vi "OCV Histogram 4309.vi"(8 "Error In":errorcluster, 10 "Results Input":T4={"V ch0 Array"=[], "V ch1 Array"=[], "V ch2 Array"=[], "V ch3 Array"=[], "V ch4 Array"=[], "Elapsed Time (ms)"=11164, "DMM Fault Array"=[]}) -> (0 "Error Out":errorcluster, 1 "mean values of channels":dbl[](array[numeric])=[-6.648192609520545e-06, -2.6579412172609335e-06, 5.730660716698524e-06, 9.480335334891014e-06, -2.6031729589807576e-07] format="%#_7p", 2 "std dev":dbl=4.593584714427233e-07 format="%.3p", 3 "range":dbl=1.8604783993401584e-06 format="%.3p", 4 "Results Output":T3={"ch3 range"=1.5284304409643419e-06, "ch3 std dev"=3.7432297421944963e-07, "ch3 mean"=9.480335334891014e-06, "Histogram Graph ch3"={"X Values"=[8.804122636382775e-06, 8.956965680479209e-06, 9.109808724575643e-06, 9.262651768672077e-06, 9.415494812768511e-06, 9.568337856864946e-06, 9.72118090096138e-06, 9.874023945057814e-06, 1.0026866989154248e-05, 1.0179710033250682e-05], "Histogram: h(x)"=[2, 4, 3, 7, 5, 3, 7, 6, 1, 2]}, "ch2 range"=1.9041594218219493e-06, "ch2 std dev"=4.1579103732429095e-07, "ch2 mean"=5.730660716698524e-06, "Histogram Graph ch2"={"X Values"=[4.8417078226500296e-06, 5.032123764832224e-06, 5.222539707014419e-06, 5.412955649196613e-06, 5.603371591378808e-06, 5.7937875335610025e-06, 5.984203475743197e-06, 6.174619417925392e-06, 6.365035360107586e-06, 6.555451302289781e-06], "Histogram: h(x)"=[2, 2, 4, 3, 5, 8, 9, 5, 1, 1]}, "ch1 range"=1.7442902903444177e-06, "ch1 std dev"=4.468204660544414e-07, "ch1 mean"=-2.6579412172609335e-06, "Histogram Graph ch1"={"X Values"=[-3.3982864936427982e-06, -3.2238574646083565e-06, -3.0494284355739147e-06, -2.874999406539473e-06, -2.700570377505031e-06, -2.5261413484705894e-06, -2.3517123194361476e-06, -2.177283290401706e-06, -2.002854261367264e-06, -1.8284252323328223e-06], "Histogram: h(x)"=[4, 3, 5, 1, 6, 8, 4, 5, 3, 1]}, "ch0 range"=1.9838415017287296e-06, "ch0 std dev"=5.022029434534627e-07, "ch0 mean"=-6.648192609520545e-06, "Histogram Graph ch0"={"X Values"=[-7.4214795585101575e-06, -7.223095408337285e-06, -7.024711258164412e-06, -6.82632710799154e-06, -6.627942957818667e-06, -6.4295588076457944e-06, -6.231174657472922e-06, -6.032790507300049e-06, -5.8344063571271766e-06, -5.636022206954304e-06], "Histogram: h(x)"=[5, 3, 4, 6, 4, 8, 4, 1, 4, 1]}, "Waveform Chart ch1"=[-2.622437675041801e-06, -2.1054414953660847e-06, -2.3277676624794484e-06, -2.558376653803712e-06, -2.2236999675494533e-06, -2.589016451053761e-06, -2.6354278960691e-06, -2.7367192087189563e-06, -2.424017879995447e-06, -3.0489161443253215e-06, -3.1442148467963687e-06, -2.4032855210096374e-06, -2.569647882839888e-06, -2.4698150005498013e-06, -3.0781658817195746e-06, -2.377010372332436e-06, -2.0435595699758798e-06, -2.106839167327596e-06, -1.7412107178156014e-06, -3.2480049993772076e-06, -1.9805074376907754e-06, -2.5608807141114243e-06, -2.18054640635336e-06, -3.099457174386434e-06, -3.102303246629032e-06, -3.2920758007788295e-06, -3.3778499352142414e-06, -3.3187560901861313e-06, -3.484840052811922e-06, -3.485501008160019e-06, -2.8728971850629594e-06, -2.6623123946996634e-06, -2.187546597757112e-06, -2.5467930720162336e-06, -2.7862697099761513e-06, -2.528638777412977e-06, -2.0537236385737207e-06, -2.5329982714180255e-06, -2.7424337661967574e-06, -3.067742416854491e-06], "Waveform Chart ch2"=[5.544446756924017e-06, 5.893818847440082e-06, 5.6959361744068e-06, 6.353655436755351e-06, 6.650659273380882e-06, 6.187390686867271e-06, 6.20360970192913e-06, 5.7770612172558695e-06, 5.816303483036932e-06, 5.681492261411933e-06, 5.92762437831725e-06, 6.190843181120228e-06, 5.928079790707314e-06, 6.068116911256402e-06, 6.161619546592655e-06, 5.5543262999422065e-06, 6.17040032539053e-06, 5.4655577958543896e-06, 5.76704970728763e-06, 6.0194055222271105e-06, 5.783390336812049e-06, 5.768011867723238e-06, 6.0153044120154e-06, 6.001437704705948e-06, 5.911709913790112e-06, 5.830095407868431e-06, 5.25398022881523e-06, 5.15697143423068e-06, 4.826305970962092e-06, 5.462550730311096e-06, 5.059430867978049e-06, 5.682513029845579e-06, 5.851683523904261e-06, 5.099226732675129e-06, 5.2309820281174504e-06, 5.22374278950658e-06, 5.829274618675769e-06, 4.746499851558932e-06, 5.396447289671177e-06, 6.039472630669777e-06], "Waveform Chart ch0"=[-6.482741875349764e-06, -6.609674165618734e-06, -6.233203080218623e-06, -6.613210951394088e-06, -5.909245924550351e-06, -6.1328996888307884e-06, -6.358200673203053e-06, -6.870973185430456e-06, -6.243427483099904e-06, -5.953840097279857e-06, -6.577614794730629e-06, -5.768388563769013e-06, -5.889962020259323e-06, -5.91212430154465e-06, -6.419565311385181e-06, -6.50829315132552e-06, -5.536830131867864e-06, -6.271011369459595e-06, -6.937542782195293e-06, -7.44168991871554e-06, -6.8984467501811205e-06, -7.4441074466820366e-06, -6.884514522294152e-06, -7.229455884586274e-06, -7.204633996616539e-06, -7.520671633596594e-06, -7.348344858091178e-06, -7.026224856705287e-06, -6.4957495291395714e-06, -6.9697185324009035e-06, -6.64170832689038e-06, -6.516226556717238e-06, -6.80187883727134e-06, -7.473746530800666e-06, -6.8019074543289836e-06, -6.421730747707948e-06, -6.915517716049444e-06, -7.233306065769019e-06, -6.9335647318597554e-06, -6.495809932905111e-06], "Waveform Chart ch3"=[9.329772359568193e-06, 9.772186603754015e-06, 9.974785258468733e-06, 1.02561315552989e-05, 9.495402230894659e-06, 9.736598828932665e-06, 9.898850155608759e-06, 1.0197036488504313e-05, 9.305987891150035e-06, 9.316802834906767e-06, 9.746712874470878e-06, 9.737416581604666e-06, 9.867514527065477e-06, 9.509080464808271e-06, 9.481845866845764e-06, 9.70755176396829e-06, 8.885838770613302e-06, 9.475699672125386e-06, 9.258180372816345e-06, 9.834891872602234e-06, 9.402243918552161e-06, 9.713205786936326e-06, 9.876491292911543e-06, 9.871789580104262e-06, 9.650930388911628e-06, 9.41118365911455e-06, 9.575353492249282e-06, 9.196921234035763e-06, 9.15123272945548e-06, 8.949563027841687e-06, 9.474861956745276e-06, 8.825224921180636e-06, 8.727701114334558e-06, 9.16860173648142e-06, 8.905227736485157e-06, 9.144446889757383e-06, 8.885482293855075e-06, 9.859395612279415e-06, 9.32444154185109e-06, 9.310827508550253e-06]} {"ch3 range" format="%#_6p"; "ch3 std dev" format="%#.3p"; "ch3 mean" format="%#.6p"; "ch2 range" format="%#_6p"; "ch2 std dev" format="%#.3p"; "ch2 mean" format="%#.6p"; "ch1 range" format="%#_6p"; "ch1 std dev" format="%#.3p"; "ch1 mean" format="%#.6p"; "ch0 range" format="%#_6p"; "ch0 std dev" format="%#.3p"; "ch0 mean" format="%#.6p"}, 5 "Elapsed Time (ms)":u32)   [LabVIEW 2019]
uses:
  OCVResults.ctl
  Chart_Graph_Mean_Range_StdDev.ctl
  VIs/MeasurementServer_OCVRawData.ctl
  VIs/MeasurementServer_ErrorOutData.ctl
  <vilib>/Analysis/baseanly.llb/Mean (DBL).vi
  <vilib>/Analysis/NI_AALBase.lvlib
  <vilib>/gmath/NI_Gmath.lvlib
  VIs/labview-grpc-measurement-server.lvlib
panel:
  in  "OCVResults":T1[](array[typedef])=[{"battery1voltage"=3.4816353, "battery2voltage"=3.4830456, "battery3voltage"=3.4783695, "battery4voltage"=3.482367, "battery5voltage"=3.4843996, "battery6voltage"=0.0, "battery7voltage"=0.0, "battery8voltage"=0.0, "battery9voltage"=0.0, "battery10voltage"=0.0, "battery11voltage"=0.0, "battery12voltage"=0.0, "battery13voltage"=0.0, "battery14voltage"=0.0, "battery15voltage"=0.0, "battery16voltage"=0.0, "battery17voltage"=0.0, "battery18voltage"=0.0, "battery19voltage"=0.0, "battery20voltage"=0.0, "battery21voltage"=0.0, "battery22voltage"=0.0, "battery23voltage"=0.0, "battery24voltage"=0.0, "ErrorOutData"={"ErrorCode"=0, "ErrorMessage"=""}}, {"battery1voltage"=3.4816356, "battery2voltage"=3.4830368, "battery3voltage"=3.4783683, "battery4voltage"=3.4823706, "battery5voltage"=3.4844058, "battery6voltage"=0.0, "battery7voltage"=0.0, "battery8voltage"=0.0, "battery9voltage"=0.0, "battery10voltage"=0.0, "battery11voltage"=0.0, "battery12voltage"=0.0, "battery13voltage"=0.0, "battery14voltage"=0.0, "battery15voltage"=0.0, "battery16voltage"=0.0, "battery17voltage"=0.0, "battery18voltage"=0.0, "battery19voltage"=0.0, "battery20voltage"=0.0, "battery21voltage"=0.0, "battery22voltage"=0.0, "battery23voltage"=0.0, "battery24voltage"=0.0, "ErrorOutData"={"ErrorCode"=0, "ErrorMessage"=""}}, {"battery1voltage"=3.4816363, "battery2voltage"=3.4830387, "battery3voltage"=3.478373, "battery4voltage"=3.4823644, "battery5voltage"=3.4844077, "battery6voltage"=0.0, "battery7voltage"=0.0, "battery8voltage"=0.0, "battery9voltage"=0.0, "battery10voltage"=0.0, "battery11voltage"=0.0, "battery12voltage"=0.0, "battery13voltage"=0.0, "battery14voltage"=0.0, "battery15voltage"=0.0, "battery16voltage"=0.0, "battery17voltage"=0.0, "battery18voltage"=0.0, "battery19voltage"=0.0, "battery20voltage"=0.0, "battery21voltage"=0.0, "battery22voltage"=0.0, "battery23voltage"=0.0, "battery24voltage"=0.0, "ErrorOutData"={"ErrorCode"=0, "ErrorMessage"=""}}, {"battery1voltage"=3.4816382, "battery2voltage"=3.4830468, "battery3voltage"=3.478372, "battery4voltage"=3.4823663, "battery5voltage"=3.4844036, "battery6voltage"=0.0, "battery7voltage"=0.0, "battery8voltage"=0.0, "battery9voltage"=0.0, "battery10voltage"=0.0, "battery11voltage"=0.0, "battery12voltage"=0.0, "battery13voltage"=0.0, "battery14voltage"=0.0, "battery15voltage"=0.0, "battery16voltage"=0.0, "battery17voltage"=0.0, "battery18voltage"=0.0, "battery19voltage"=0.0, "battery20voltage"=0.0, "battery21voltage"=0.0, "battery22voltage"=0.0, "battery23voltage"=0.0, "battery24voltage"=0.0, "ErrorOutData"={"ErrorCode"=0, "ErrorMessage"=""}}, {"battery1voltage"=3.4816408, "battery2voltage"=3.4830465, "battery3voltage"=3.478378, "battery4voltage"=3.48237, "battery5voltage"=3.4843988, "battery6voltage"=0.0, "battery7voltage"=0.0, "battery8voltage"=0.0, "battery9voltage"=0.0, "battery10voltage"=0.0, "battery11voltage"=0.0, "battery12voltage"=0.0, "battery13voltage"=0.0, "battery14voltage"=0.0, "battery15voltage"=0.0, "battery16voltage"=0.0, "battery17voltage"=0.0, "battery18voltage"=0.0, "battery19voltage"=0.0, "battery20voltage"=0.0, "battery21voltage"=0.0, "battery22voltage"=0.0, "battery23voltage"=0.0, "battery24voltage"=0.0, "ErrorOutData"={"ErrorCode"=0, "ErrorMessage"=""}}, {"battery1voltage"=3.48164, "battery2voltage"=3.4830382, "battery3voltage"=3.4783747, "battery4voltage"=3.4823658, "battery5voltage"=3.4843998, "battery6voltage"=0.0, "battery7voltage"=0.0, "battery8voltage"=0.0, "battery9voltage"=0.0, "battery10voltage"=0.0, "battery11voltage"=0.0, "battery12voltage"=0.0, "battery13voltage"=0.0, "battery14voltage"=0.0, "battery15voltage"=0.0, "battery16voltage"=0.0, "battery17voltage"=0.0, "battery18voltage"=0.0, "battery19voltage"=0.0, "battery20voltage"=0.0, "battery21voltage"=0.0, "battery22voltage"=0.0, "battery23voltage"=0.0, "battery24voltage"=0.0, "ErrorOutData"={"ErrorCode"=0, "ErrorMessage"=""}}, {"battery1voltage"=3.481639, "battery2voltage"=3.4830444, "battery3voltage"=3.4783697, "battery4voltage"=3.482369, "battery5voltage"=3.4844058, "battery6voltage"=0.0, "battery7voltage"=0.0, "battery8voltage"=0.0, "battery9voltage"=0.0, "battery10voltage"=0.0, "battery11voltage"=0.0, "battery12voltage"=0.0, "battery13voltage"=0.0, "battery14voltage"=0.0, "battery15voltage"=0.0, "battery16voltage"=0.0, "battery17voltage"=0.0, "battery18voltage"=0.0, "battery19voltage"=0.0, "battery20voltage"=0.0, "battery21voltage"=0.0, "battery22voltage"=0.0, "battery23voltage"=0.0, "battery24voltage"=0.0, "ErrorOutData"={"ErrorCode"=0, "ErrorMessage"=""}}, {"battery1voltage"=3.4816341, "battery2voltage"=3.483041, "battery3voltage"=3.4783704, "battery4voltage"=3.4823651, "battery5voltage"=3.4844072, "battery6voltage"=0.0, "battery7voltage"=0.0, "battery8voltage"=0.0, "battery9voltage"=0.0, "battery10voltage"=0.0, "battery11voltage"=0.0, "battery12voltage"=0.0, "battery13voltage"=0.0, "battery14voltage"=0.0, "battery15voltage"=0.0, "battery16voltage"=0.0, "battery17voltage"=0.0, "battery18voltage"=0.0, "battery19voltage"=0.0, "battery20voltage"=0.0, "battery21voltage"=0.0, "battery22voltage"=0.0, "battery23voltage"=0.0, "battery24voltage"=0.0, "ErrorOutData"={"ErrorCode"=0, "ErrorMessage"=""}}, {"battery1voltage"=3.481641, "battery2voltage"=3.4830418, "battery3voltage"=3.4783719, "battery4voltage"=3.482372, "battery5voltage"=3.4844098, "battery6voltage"=0.0, "battery7voltage"=0.0, "battery8voltage"=0.0, "battery9voltage"=0.0, "battery10voltage"=0.0, "battery11voltage"=0.0, "battery12voltage"=0.0, "battery13voltage"=0.0, "battery14voltage"=0.0, "battery15voltage"=0.0, "battery16voltage"=0.0, "battery17voltage"=0.0, "battery18voltage"=0.0, "battery19voltage"=0.0, "battery20voltage"=0.0, "battery21voltage"=0.0, "battery22voltage"=0.0, "battery23voltage"=0.0, "battery24voltage"=0.0, "ErrorOutData"={"ErrorCode"=0, "ErrorMessage"=""}}, {"battery1voltage"=3.4816356, "battery2voltage"=3.4830396, "battery3voltage"=3.478371, "battery4voltage"=3.4823728, "battery5voltage"=3.4844012, "battery6voltage"=0.0, "battery7voltage"=0.0, "battery8voltage"=0.0, "battery9voltage"=0.0, "battery10voltage"=0.0, "battery11voltage"=0.0, "battery12voltage"=0.0, "battery13voltage"=0.0, "battery14voltage"=0.0, "battery15voltage"=0.0, "battery16voltage"=0.0, "battery17voltage"=0.0, "battery18voltage"=0.0, "battery19voltage"=0.0, "battery20voltage"=0.0, "battery21voltage"=0.0, "battery22voltage"=0.0, "battery23voltage"=0.0, "battery24voltage"=0.0, "ErrorOutData"={"ErrorCode"=0, "ErrorMessage"=""}}, {"battery1voltage"=3.4816346, "battery2voltage"=3.483039, "battery3voltage"=3.478373, "battery4voltage"=3.4823637, "battery5voltage"=3.4844048, "battery6voltage"=0.0, "battery7voltage"=0.0, "battery8voltage"=0.0, "battery9voltage"=0.0, "battery10voltage"=0.0, "battery11voltage"=0.0, "battery12voltage"=0.0, "battery13voltage"=0.0, "battery14voltage"=0.0, "battery15voltage"=0.0, "battery16voltage"=0.0, "battery17voltage"=0.0, "battery18voltage"=0.0, "battery19voltage"=0.0, "battery20voltage"=0.0, "battery21voltage"=0.0, "battery22voltage"=0.0, "battery23voltage"=0.0, "battery24voltage"=0.0, "ErrorOutData"={"ErrorCode"=0, "ErrorMessage"=""}}, {"battery1voltage"=3.4816375, "battery2voltage"=3.4830399, "battery3voltage"=3.4783738, "battery4voltage"=3.4823651, "battery5voltage"=3.4844062, "battery6voltage"=0.0, "battery7voltage"=0.0, "battery8voltage"=0.0, "battery9voltage"=0.0, "battery10voltage"=0.0, "battery11voltage"=0.0, "battery12voltage"=0.0, "battery13voltage"=0.0, "battery14voltage"=0.0, "battery15voltage"=0.0, "battery16voltage"=0.0, "battery17voltage"=0.0, "battery18voltage"=0.0, "battery19voltage"=0.0, "battery20voltage"=0.0, "battery21voltage"=0.0, "battery22voltage"=0.0, "battery23voltage"=0.0, "battery24voltage"=0.0, "ErrorOutData"={"ErrorCode"=0, "ErrorMessage"=""}}, {"battery1voltage"=3.4816372, "battery2voltage"=3.4830463, "battery3voltage"=3.478377, "battery4voltage"=3.4823728, "battery5voltage"=3.484404, "battery6voltage"=0.0, "battery7voltage"=0.0, "battery8voltage"=0.0, "battery9voltage"=0.0, "battery10voltage"=0.0, "battery11voltage"=0.0, "battery12voltage"=0.0, "battery13voltage"=0.0, "battery14voltage"=0.0, "battery15voltage"=0.0, "battery16voltage"=0.0, "battery17voltage"=0.0, "battery18voltage"=0.0, "battery19voltage"=0.0, "battery20voltage"=0.0, "battery21voltage"=0.0, "battery22voltage"=0.0, "battery23voltage"=0.0, "battery24voltage"=0.0, "ErrorOutData"={"ErrorCode"=0, "ErrorMessage"=""}}, {"battery1voltage"=3.481637, "battery2voltage"=3.4830413, "battery3voltage"=3.4783728, "battery4voltage"=3.482369, "battery5voltage"=3.484405, "battery6voltage"=0.0, "battery7voltage"=0.0, "battery8voltage"=0.0, "battery9voltage"=0.0, "battery10voltage"=0.0, "battery11voltage"=0.0, "battery12voltage"=0.0, "battery13voltage"=0.0, "battery14voltage"=0.0, "battery15voltage"=0.0, "battery16voltage"=0.0, "battery17voltage"=0.0, "battery18voltage"=0.0, "battery19voltage"=0.0, "battery20voltage"=0.0, "battery21voltage"=0.0, "battery22voltage"=0.0, "battery23voltage"=0.0, "battery24voltage"=0.0, "ErrorOutData"={"ErrorCode"=0, "ErrorMessage"=""}}, {"battery1voltage"=3.4816399, "battery2voltage"=3.4830387, "battery3voltage"=3.4783702, "battery4voltage"=3.4823713, "battery5voltage"=3.4844084, "battery6voltage"=0.0, "battery7voltage"=0.0, "battery8voltage"=0.0, "battery9voltage"=0.0, "battery10voltage"=0.0, "battery11voltage"=0.0, "battery12voltage"=0.0, "battery13voltage"=0.0, "battery14voltage"=0.0, "battery15voltage"=0.0, "battery16voltage"=0.0, "battery17voltage"=0.0, "battery18voltage"=0.0, "battery19voltage"=0.0, "battery20voltage"=0.0, "battery21voltage"=0.0, "battery22voltage"=0.0, "battery23voltage"=0.0, "battery24voltage"=0.0, "ErrorOutData"={"ErrorCode"=0, "ErrorMessage"=""}}, {"battery1voltage"=3.4816375, "battery2voltage"=3.4830422, "battery3voltage"=3.4783688, "battery4voltage"=3.4823675, "battery5voltage"=3.4843993, "battery6voltage"=0.0, "battery7voltage"=0.0, "battery8voltage"=0.0, "battery9voltage"=0.0, "battery10voltage"=0.0, "battery11voltage"=0.0, "battery12voltage"=0.0, "battery13voltage"=0.0, "battery14voltage"=0.0, "battery15voltage"=0.0, "battery16voltage"=0.0, "battery17voltage"=0.0, "battery18voltage"=0.0, "battery19voltage"=0.0, "battery20voltage"=0.0, "battery21voltage"=0.0, "battery22voltage"=0.0, "battery23voltage"=0.0, "battery24voltage"=0.0, "ErrorOutData"={"ErrorCode"=0, "ErrorMessage"=""}}, {"battery1voltage"=3.4816432, "battery2voltage"=3.4830387, "battery3voltage"=3.478373, "battery4voltage"=3.482368, "battery5voltage"=3.484403, "battery6voltage"=0.0, "battery7voltage"=0.0, "battery8voltage"=0.0, "battery9voltage"=0.0, "battery10voltage"=0.0, "battery11voltage"=0.0, "battery12voltage"=0.0, "battery13voltage"=0.0, "battery14voltage"=0.0, "battery15voltage"=0.0, "battery16voltage"=0.0, "battery17voltage"=0.0, "battery18voltage"=0.0, "battery19voltage"=0.0, "battery20voltage"=0.0, "battery21voltage"=0.0, "battery22voltage"=0.0, "battery23voltage"=0.0, "battery24voltage"=0.0, "ErrorOutData"={"ErrorCode"=0, "ErrorMessage"=""}}, {"battery1voltage"=3.4816358, "battery2voltage"=3.483043, "battery3voltage"=3.4783685, "battery4voltage"=3.4823685, "battery5voltage"=3.484403, "battery6voltage"=0.0, "battery7voltage"=0.0, "battery8voltage"=0.0, "battery9voltage"=0.0, "battery10voltage"=0.0, "battery11voltage"=0.0, "battery12voltage"=0.0, "battery13voltage"=0.0, "battery14voltage"=0.0, "battery15voltage"=0.0, "battery16voltage"=0.0, "battery17voltage"=0.0, "battery18voltage"=0.0, "battery19voltage"=0.0, "battery20voltage"=0.0, "battery21voltage"=0.0, "battery22voltage"=0.0, "battery23voltage"=0.0, "battery24voltage"=0.0, "ErrorOutData"={"ErrorCode"=0, "ErrorMessage"=""}}, {"battery1voltage"=3.4816375, "battery2voltage"=3.483041, "battery3voltage"=3.4783714, "battery4voltage"=3.4823701, "battery5voltage"=3.484405, "battery6voltage"=0.0, "battery7voltage"=0.0, "battery8voltage"=0.0, "battery9voltage"=0.0, "battery10voltage"=0.0, "battery11voltage"=0.0, "battery12voltage"=0.0, "battery13voltage"=0.0, "battery14voltage"=0.0, "battery15voltage"=0.0, "battery16voltage"=0.0, "battery17voltage"=0.0, "battery18voltage"=0.0, "battery19voltage"=0.0, "battery20voltage"=0.0, "battery21voltage"=0.0, "battery22voltage"=0.0, "battery23voltage"=0.0, "battery24voltage"=0.0, "ErrorOutData"={"ErrorCode"=0, "ErrorMessage"=""}}, {"battery1voltage"=3.48164, "battery2voltage"=3.4830444, "battery3voltage"=3.4783697, "battery4voltage"=3.4823718, "battery5voltage"=3.4844031, "battery6voltage"=0.0, "battery7voltage"=0.0, "battery8voltage"=0.0, "battery9voltage"=0.0, "battery10voltage"=0.0, "battery11voltage"=0.0, "battery12voltage"=0.0, "battery13voltage"=0.0, "battery14voltage"=0.0, "battery15voltage"=0.0, "battery16voltage"=0.0, "battery17voltage"=0.0, "battery18voltage"=0.0, "battery19voltage"=0.0, "battery20voltage"=0.0, "battery21voltage"=0.0, "battery22voltage"=0.0, "battery23voltage"=0.0, "battery24voltage"=0.0, "ErrorOutData"={"ErrorCode"=0, "ErrorMessage"=""}}, {"battery1voltage"=3.4816394, "battery2voltage"=3.4830453, "battery3voltage"=3.4783723, "battery4voltage"=3.4823713, "battery5voltage"=3.4843984, "battery6voltage"=0.0, "battery7voltage"=0.0, "battery8voltage"=0.0, "battery9voltage"=0.0, "battery10voltage"=0.0, "battery11voltage"=0.0, "battery12voltage"=0.0, "battery13voltage"=0.0, "battery14voltage"=0.0, "battery15voltage"=0.0, "battery16voltage"=0.0, "battery17voltage"=0.0, "battery18voltage"=0.0, "battery19voltage"=0.0, "battery20voltage"=0.0, "battery21voltage"=0.0, "battery22voltage"=0.0, "battery23voltage"=0.0, "battery24voltage"=0.0, "ErrorOutData"={"ErrorCode"=0, "ErrorMessage"=""}}, {"battery1voltage"=3.4816341, "battery2voltage"=3.4830413, "battery3voltage"=3.4783728, "battery4voltage"=3.4823737, "battery5voltage"=3.4844046, "battery6voltage"=0.0, "battery7voltage"=0.0, "battery8voltage"=0.0, "battery9voltage"=0.0, "battery10voltage"=0.0, "battery11voltage"=0.0, "battery12voltage"=0.0, "battery13voltage"=0.0, "battery14voltage"=0.0, "battery15voltage"=0.0, "battery16voltage"=0.0, "battery17voltage"=0.0, "battery18voltage"=0.0, "battery19voltage"=0.0, "battery20voltage"=0.0, "battery21voltage"=0.0, "battery22voltage"=0.0, "battery23voltage"=0.0, "battery24voltage"=0.0, "ErrorOutData"={"ErrorCode"=0, "ErrorMessage"=""}}, {"battery1voltage"=3.4816387, "battery2voltage"=3.4830446, "battery3voltage"=3.4783685, "battery4voltage"=3.482368, "battery5voltage"=3.4844067, "battery6voltage"=0.0, "battery7voltage"=0.0, "battery8voltage"=0.0, "battery9voltage"=0.0, "battery10voltage"=0.0, "battery11voltage"=0.0, "battery12voltage"=0.0, "battery13voltage"=0.0, "battery14voltage"=0.0, "battery15voltage"=0.0, "battery16voltage"=0.0, "battery17voltage"=0.0, "battery18voltage"=0.0, "battery19voltage"=0.0, "battery20voltage"=0.0, "battery21voltage"=0.0, "battery22voltage"=0.0, "battery23voltage"=0.0, "battery24voltage"=0.0, "ErrorOutData"={"ErrorCode"=0, "ErrorMessage"=""}}, {"battery1voltage"=3.4816349, "battery2voltage"=3.48304, "battery3voltage"=3.4783728, "battery4voltage"=3.482367, "battery5voltage"=3.4844062, "battery6voltage"=0.0, "battery7voltage"=0.0, "battery8voltage"=0.0, "battery9voltage"=0.0, "battery10voltage"=0.0, "battery11voltage"=0.0, "battery12voltage"=0.0, "battery13voltage"=0.0, "battery14voltage"=0.0, "battery15voltage"=0.0, "battery16voltage"=0.0, "battery17voltage"=0.0, "battery18voltage"=0.0, "battery19voltage"=0.0, "battery20voltage"=0.0, "battery21voltage"=0.0, "battery22voltage"=0.0, "battery23voltage"=0.0, "battery24voltage"=0.0, "ErrorOutData"={"ErrorCode"=0, "ErrorMessage"=""}}, {"battery1voltage"=3.4816382, "battery2voltage"=3.483041, "battery3voltage"=3.4783733, "battery4voltage"=3.4823716, "battery5voltage"=3.4844053, "battery6voltage"=0.0, "battery7voltage"=0.0, "battery8voltage"=0.0, "battery9voltage"=0.0, "battery10voltage"=0.0, "battery11voltage"=0.0, "battery12voltage"=0.0, "battery13voltage"=0.0, "battery14voltage"=0.0, "battery15voltage"=0.0, "battery16voltage"=0.0, "battery17voltage"=0.0, "battery18voltage"=0.0, "battery19voltage"=0.0, "battery20voltage"=0.0, "battery21voltage"=0.0, "battery22voltage"=0.0, "battery23voltage"=0.0, "battery24voltage"=0.0, "ErrorOutData"={"ErrorCode"=0, "ErrorMessage"=""}}, {"battery1voltage"=3.481638, "battery2voltage"=3.4830427, "battery3voltage"=3.4783704, "battery4voltage"=3.4823666, "battery5voltage"=3.4844048, "battery6voltage"=0.0, "battery7voltage"=0.0, "battery8voltage"=0.0, "battery9voltage"=0.0, "battery10voltage"=0.0, "battery11voltage"=0.0, "battery12voltage"=0.0, "battery13voltage"=0.0, "battery14voltage"=0.0, "battery15voltage"=0.0, "battery16voltage"=0.0, "battery17voltage"=0.0, "battery18voltage"=0.0, "battery19voltage"=0.0, "battery20voltage"=0.0, "battery21voltage"=0.0, "battery22voltage"=0.0, "battery23voltage"=0.0, "battery24voltage"=0.0, "ErrorOutData"={"ErrorCode"=0, "ErrorMessage"=""}}, {"battery1voltage"=3.4816375, "battery2voltage"=3.4830396, "battery3voltage"=3.4783683, "battery4voltage"=3.482369, "battery5voltage"=3.4844077, "battery6voltage"=0.0, "battery7voltage"=0.0, "battery8voltage"=0.0, "battery9voltage"=0.0, "battery10voltage"=0.0, "battery11voltage"=0.0, "battery12voltage"=0.0, "battery13voltage"=0.0, "battery14voltage"=0.0, "battery15voltage"=0.0, "battery16voltage"=0.0, "battery17voltage"=0.0, "battery18voltage"=0.0, "battery19voltage"=0.0, "battery20voltage"=0.0, "battery21voltage"=0.0, "battery22voltage"=0.0, "battery23voltage"=0.0, "battery24voltage"=0.0, "ErrorOutData"={"ErrorCode"=0, "ErrorMessage"=""}}, {"battery1voltage"=3.4816344, "battery2voltage"=3.4830408, "battery3voltage"=3.4783728, "battery4voltage"=3.4823692, "battery5voltage"=3.4844024, "battery6voltage"=0.0, "battery7voltage"=0.0, "battery8voltage"=0.0, "battery9voltage"=0.0, "battery10voltage"=0.0, "battery11voltage"=0.0, "battery12voltage"=0.0, "battery13voltage"=0.0, "battery14voltage"=0.0, "battery15voltage"=0.0, "battery16voltage"=0.0, "battery17voltage"=0.0, "battery18voltage"=0.0, "battery19voltage"=0.0, "battery20voltage"=0.0, "battery21voltage"=0.0, "battery22voltage"=0.0, "battery23voltage"=0.0, "battery24voltage"=0.0, "ErrorOutData"={"ErrorCode"=0, "ErrorMessage"=""}}, {"battery1voltage"=3.4816382, "battery2voltage"=3.483045, "battery3voltage"=3.478367, "battery4voltage"=3.4823682, "battery5voltage"=3.484407, "battery6voltage"=0.0, "battery7voltage"=0.0, "battery8voltage"=0.0, "battery9voltage"=0.0, "battery10voltage"=0.0, "battery11voltage"=0.0, "battery12voltage"=0.0, "battery13voltage"=0.0, "battery14voltage"=0.0, "battery15voltage"=0.0, "battery16voltage"=0.0, "battery17voltage"=0.0, "battery18voltage"=0.0, "battery19voltage"=0.0, "battery20voltage"=0.0, "battery21voltage"=0.0, "battery22voltage"=0.0, "battery23voltage"=0.0, "battery24voltage"=0.0, "ErrorOutData"={"ErrorCode"=0, "ErrorMessage"=""}}, {"battery1voltage"=3.4816399, "battery2voltage"=3.483045, "battery3voltage"=3.4783711, "battery4voltage"=3.482368, "battery5voltage"=3.4843976, "battery6voltage"=0.0, "battery7voltage"=0.0, "battery8voltage"=0.0, "battery9voltage"=0.0, "battery10voltage"=0.0, "battery11voltage"=0.0, "battery12voltage"=0.0, "battery13voltage"=0.0, "battery14voltage"=0.0, "battery15voltage"=0.0, "battery16voltage"=0.0, "battery17voltage"=0.0, "battery18voltage"=0.0, "battery19voltage"=0.0, "battery20voltage"=0.0, "battery21voltage"=0.0, "battery22voltage"=0.0, "battery23voltage"=0.0, "battery24voltage"=0.0, "ErrorOutData"={"ErrorCode"=0, "ErrorMessage"=""}}, {"battery1voltage"=3.4816442, "battery2voltage"=3.4830372, "battery3voltage"=3.4783738, "battery4voltage"=3.482372, "battery5voltage"=3.4844053, "battery6voltage"=0.0, "battery7voltage"=0.0, "battery8voltage"=0.0, "battery9voltage"=0.0, "battery10voltage"=0.0, "battery11voltage"=0.0, "battery12voltage"=0.0, "battery13voltage"=0.0, "battery14voltage"=0.0, "battery15voltage"=0.0, "battery16voltage"=0.0, "battery17voltage"=0.0, "battery18voltage"=0.0, "battery19voltage"=0.0, "battery20voltage"=0.0, "battery21voltage"=0.0, "battery22voltage"=0.0, "battery23voltage"=0.0, "battery24voltage"=0.0, "ErrorOutData"={"ErrorCode"=0, "ErrorMessage"=""}}, {"battery1voltage"=3.4816413, "battery2voltage"=3.4830437, "battery3voltage"=3.4783747, "battery4voltage"=3.482368, "battery5voltage"=3.4843984, "battery6voltage"=0.0, "battery7voltage"=0.0, "battery8voltage"=0.0, "battery9voltage"=0.0, "battery10voltage"=0.0, "battery11voltage"=0.0, "battery12voltage"=0.0, "battery13voltage"=0.0, "battery14voltage"=0.0, "battery15voltage"=0.0, "battery16voltage"=0.0, "battery17voltage"=0.0, "battery18voltage"=0.0, "battery19voltage"=0.0, "battery20voltage"=0.0, "battery21voltage"=0.0, "battery22voltage"=0.0, "battery23voltage"=0.0, "battery24voltage"=0.0, "ErrorOutData"={"ErrorCode"=0, "ErrorMessage"=""}}, {"battery1voltage"=3.481636, "battery2voltage"=3.4830418, "battery3voltage"=3.4783738, "battery4voltage"=3.482369, "battery5voltage"=3.4844093, "battery6voltage"=0.0, "battery7voltage"=0.0, "battery8voltage"=0.0, "battery9voltage"=0.0, "battery10voltage"=0.0, "battery11voltage"=0.0, "battery12voltage"=0.0, "battery13voltage"=0.0, "battery14voltage"=0.0, "battery15voltage"=0.0, "battery16voltage"=0.0, "battery17voltage"=0.0, "battery18voltage"=0.0, "battery19voltage"=0.0, "battery20voltage"=0.0, "battery21voltage"=0.0, "battery22voltage"=0.0, "battery23voltage"=0.0, "battery24voltage"=0.0, "ErrorOutData"={"ErrorCode"=0, "ErrorMessage"=""}}, {"battery1voltage"=3.4816372, "battery2voltage"=3.4830408, "battery3voltage"=3.4783714, "battery4voltage"=3.4823658, "battery5voltage"=3.4844065, "battery6voltage"=0.0, "battery7voltage"=0.0, "battery8voltage"=0.0, "battery9voltage"=0.0, "battery10voltage"=0.0, "battery11voltage"=0.0, "battery12voltage"=0.0, "battery13voltage"=0.0, "battery14voltage"=0.0, "battery15voltage"=0.0, "battery16voltage"=0.0, "battery17voltage"=0.0, "battery18voltage"=0.0, "battery19voltage"=0.0, "battery20voltage"=0.0, "battery21voltage"=0.0, "battery22voltage"=0.0, "battery23voltage"=0.0, "battery24voltage"=0.0, "ErrorOutData"={"ErrorCode"=0, "ErrorMessage"=""}}, {"battery1voltage"=3.4816327, "battery2voltage"=3.4830406, "battery3voltage"=3.47837, "battery4voltage"=3.48237, "battery5voltage"=3.4844074, "battery6voltage"=0.0, "battery7voltage"=0.0, "battery8voltage"=0.0, "battery9voltage"=0.0, "battery10voltage"=0.0, "battery11voltage"=0.0, "battery12voltage"=0.0, "battery13voltage"=0.0, "battery14voltage"=0.0, "battery15voltage"=0.0, "battery16voltage"=0.0, "battery17voltage"=0.0, "battery18voltage"=0.0, "battery19voltage"=0.0, "battery20voltage"=0.0, "battery21voltage"=0.0, "battery22voltage"=0.0, "battery23voltage"=0.0, "battery24voltage"=0.0, "ErrorOutData"={"ErrorCode"=0, "ErrorMessage"=""}}, {"battery1voltage"=3.4816341, "battery2voltage"=3.4830384, "battery3voltage"=3.4783652, "battery4voltage"=3.4823718, "battery5voltage"=3.4844053, "battery6voltage"=0.0, "battery7voltage"=0.0, "battery8voltage"=0.0, "battery9voltage"=0.0, "battery10voltage"=0.0, "battery11voltage"=0.0, "battery12voltage"=0.0, "battery13voltage"=0.0, "battery14voltage"=0.0, "battery15voltage"=0.0, "battery16voltage"=0.0, "battery17voltage"=0.0, "battery18voltage"=0.0, "battery19voltage"=0.0, "battery20voltage"=0.0, "battery21voltage"=0.0, "battery22voltage"=0.0, "battery23voltage"=0.0, "battery24voltage"=0.0, "ErrorOutData"={"ErrorCode"=0, "ErrorMessage"=""}}, {"battery1voltage"=3.4816403, "battery2voltage"=3.4830394, "battery3voltage"=3.4783738, "battery4voltage"=3.482369, "battery5voltage"=3.4843953, "battery6voltage"=0.0, "battery7voltage"=0.0, "battery8voltage"=0.0, "battery9voltage"=0.0, "battery10voltage"=0.0, "battery11voltage"=0.0, "battery12voltage"=0.0, "battery13voltage"=0.0, "battery14voltage"=0.0, "battery15voltage"=0.0, "battery16voltage"=0.0, "battery17voltage"=0.0, "battery18voltage"=0.0, "battery19voltage"=0.0, "battery20voltage"=0.0, "battery21voltage"=0.0, "battery22voltage"=0.0, "battery23voltage"=0.0, "battery24voltage"=0.0, "ErrorOutData"={"ErrorCode"=0, "ErrorMessage"=""}}, {"battery1voltage"=3.4816394, "battery2voltage"=3.4830453, "battery3voltage"=3.4783702, "battery4voltage"=3.4823678, "battery5voltage"=3.4844062, "battery6voltage"=0.0, "battery7voltage"=0.0, "battery8voltage"=0.0, "battery9voltage"=0.0, "battery10voltage"=0.0, "battery11voltage"=0.0, "battery12voltage"=0.0, "battery13voltage"=0.0, "battery14voltage"=0.0, "battery15voltage"=0.0, "battery16voltage"=0.0, "battery17voltage"=0.0, "battery18voltage"=0.0, "battery19voltage"=0.0, "battery20voltage"=0.0, "battery21voltage"=0.0, "battery22voltage"=0.0, "battery23voltage"=0.0, "battery24voltage"=0.0, "ErrorOutData"={"ErrorCode"=0, "ErrorMessage"=""}}, {"battery1voltage"=3.4816413, "battery2voltage"=3.4830458, "battery3voltage"=3.478368, "battery4voltage"=3.482369, "battery5voltage"=3.4844098, "battery6voltage"=0.0, "battery7voltage"=0.0, "battery8voltage"=0.0, "battery9voltage"=0.0, "battery10voltage"=0.0, "battery11voltage"=0.0, "battery12voltage"=0.0, "battery13voltage"=0.0, "battery14voltage"=0.0, "battery15voltage"=0.0, "battery16voltage"=0.0, "battery17voltage"=0.0, "battery18voltage"=0.0, "battery19voltage"=0.0, "battery20voltage"=0.0, "battery21voltage"=0.0, "battery22voltage"=0.0, "battery23voltage"=0.0, "battery24voltage"=0.0, "ErrorOutData"={"ErrorCode"=0, "ErrorMessage"=""}}, {"battery1voltage"=3.4816415, "battery2voltage"=3.4830437, "battery3voltage"=3.4783766, "battery4voltage"=3.4823713, "battery5voltage"=3.4844012, "battery6voltage"=0.0, "battery7voltage"=0.0, "battery8voltage"=0.0, "battery9voltage"=0.0, "battery10voltage"=0.0, "battery11voltage"=0.0, "battery12voltage"=0.0, "battery13voltage"=0.0, "battery14voltage"=0.0, "battery15voltage"=0.0, "battery16voltage"=0.0, "battery17voltage"=0.0, "battery18voltage"=0.0, "battery19voltage"=0.0, "battery20voltage"=0.0, "battery21voltage"=0.0, "battery22voltage"=0.0, "battery23voltage"=0.0, "battery24voltage"=0.0, "ErrorOutData"={"ErrorCode"=0, "ErrorMessage"=""}}, {"battery1voltage"=3.4816406, "battery2voltage"=3.4830434, "battery3voltage"=3.4783766, "battery4voltage"=3.4823692, "battery5voltage"=3.4844048, "battery6voltage"=0.0, "battery7voltage"=0.0, "battery8voltage"=0.0, "battery9voltage"=0.0, "battery10voltage"=0.0, "battery11voltage"=0.0, "battery12voltage"=0.0, "battery13voltage"=0.0, "battery14voltage"=0.0, "battery15voltage"=0.0, "battery16voltage"=0.0, "battery17voltage"=0.0, "battery18voltage"=0.0, "battery19voltage"=0.0, "battery20voltage"=0.0, "battery21voltage"=0.0, "battery22voltage"=0.0, "battery23voltage"=0.0, "battery24voltage"=0.0, "ErrorOutData"={"ErrorCode"=0, "ErrorMessage"=""}}, {"battery1voltage"=3.481637, "battery2voltage"=3.4830406, "battery3voltage"=3.478371, "battery4voltage"=3.4823666, "battery5voltage"=3.4844093, "battery6voltage"=0.0, "battery7voltage"=0.0, "battery8voltage"=0.0, "battery9voltage"=0.0, "battery10voltage"=0.0, "battery11voltage"=0.0, "battery12voltage"=0.0, "battery13voltage"=0.0, "battery14voltage"=0.0, "battery15voltage"=0.0, "battery16voltage"=0.0, "battery17voltage"=0.0, "battery18voltage"=0.0, "battery19voltage"=0.0, "battery20voltage"=0.0, "battery21voltage"=0.0, "battery22voltage"=0.0, "battery23voltage"=0.0, "battery24voltage"=0.0, "ErrorOutData"={"ErrorCode"=0, "ErrorMessage"=""}}, {"battery1voltage"=3.4816372, "battery2voltage"=3.4830427, "battery3voltage"=3.4783697, "battery4voltage"=3.4823666, "battery5voltage"=3.4844093, "battery6voltage"=0.0, "battery7voltage"=0.0, "battery8voltage"=0.0, "battery9voltage"=0.0, "battery10voltage"=0.0, "battery11voltage"=0.0, "battery12voltage"=0.0, "battery13voltage"=0.0, "battery14voltage"=0.0, "battery15voltage"=0.0, "battery16voltage"=0.0, "battery17voltage"=0.0, "battery18voltage"=0.0, "battery19voltage"=0.0, "battery20voltage"=0.0, "battery21voltage"=0.0, "battery22voltage"=0.0, "battery23voltage"=0.0, "battery24voltage"=0.0, "ErrorOutData"={"ErrorCode"=0, "ErrorMessage"=""}}, {"battery1voltage"=3.4816396, "battery2voltage"=3.483044, "battery3voltage"=3.4783752, "battery4voltage"=3.4823713, "battery5voltage"=3.4844036, "battery6voltage"=0.0, "battery7voltage"=0.0, "battery8voltage"=0.0, "battery9voltage"=0.0, "battery10voltage"=0.0, "battery11voltage"=0.0, "battery12voltage"=0.0, "battery13voltage"=0.0, "battery14voltage"=0.0, "battery15voltage"=0.0, "battery16voltage"=0.0, "battery17voltage"=0.0, "battery18voltage"=0.0, "battery19voltage"=0.0, "battery20voltage"=0.0, "battery21voltage"=0.0, "battery22voltage"=0.0, "battery23voltage"=0.0, "battery24voltage"=0.0, "ErrorOutData"={"ErrorCode"=0, "ErrorMessage"=""}}, {"battery1voltage"=3.4816391, "battery2voltage"=3.4830427, "battery3voltage"=3.478371, "battery4voltage"=3.482368, "battery5voltage"=3.4844048, "battery6voltage"=0.0, "battery7voltage"=0.0, "battery8voltage"=0.0, "battery9voltage"=0.0, "battery10voltage"=0.0, "battery11voltage"=0.0, "battery12voltage"=0.0, "battery13voltage"=0.0, "battery14voltage"=0.0, "battery15voltage"=0.0, "battery16voltage"=0.0, "battery17voltage"=0.0, "battery18voltage"=0.0, "battery19voltage"=0.0, "battery20voltage"=0.0, "battery21voltage"=0.0, "battery22voltage"=0.0, "battery23voltage"=0.0, "battery24voltage"=0.0, "ErrorOutData"={"ErrorCode"=0, "ErrorMessage"=""}}, {"battery1voltage"=3.481643, "battery2voltage"=3.4830446, "battery3voltage"=3.4783757, "battery4voltage"=3.482366, "battery5voltage"=3.4843988, "battery6voltage"=0.0, "battery7voltage"=0.0, "battery8voltage"=0.0, "battery9voltage"=0.0, "battery10voltage"=0.0, "battery11voltage"=0.0, "battery12voltage"=0.0, "battery13voltage"=0.0, "battery14voltage"=0.0, "battery15voltage"=0.0, "battery16voltage"=0.0, "battery17voltage"=0.0, "battery18voltage"=0.0, "battery19voltage"=0.0, "battery20voltage"=0.0, "battery21voltage"=0.0, "battery22voltage"=0.0, "battery23voltage"=0.0, "battery24voltage"=0.0, "ErrorOutData"={"ErrorCode"=0, "ErrorMessage"=""}}, {"battery1voltage"=3.4816375, "battery2voltage"=3.4830432, "battery3voltage"=3.47837, "battery4voltage"=3.482367, "battery5voltage"=3.4844115, "battery6voltage"=0.0, "battery7voltage"=0.0, "battery8voltage"=0.0, "battery9voltage"=0.0, "battery10voltage"=0.0, "battery11voltage"=0.0, "battery12voltage"=0.0, "battery13voltage"=0.0, "battery14voltage"=0.0, "battery15voltage"=0.0, "battery16voltage"=0.0, "battery17voltage"=0.0, "battery18voltage"=0.0, "battery19voltage"=0.0, "battery20voltage"=0.0, "battery21voltage"=0.0, "battery22voltage"=0.0, "battery23voltage"=0.0, "battery24voltage"=0.0, "ErrorOutData"={"ErrorCode"=0, "ErrorMessage"=""}}, {"battery1voltage"=3.4816341, "battery2voltage"=3.4830444, "battery3voltage"=3.4783678, "battery4voltage"=3.48237, "battery5voltage"=3.4844046, "battery6voltage"=0.0, "battery7voltage"=0.0, "battery8voltage"=0.0, "battery9voltage"=0.0, "battery10voltage"=0.0, "battery11voltage"=0.0, "battery12voltage"=0.0, "battery13voltage"=0.0, "battery14voltage"=0.0, "battery15voltage"=0.0, "battery16voltage"=0.0, "battery17voltage"=0.0, "battery18voltage"=0.0, "battery19voltage"=0.0, "battery20voltage"=0.0, "battery21voltage"=0.0, "battery22voltage"=0.0, "battery23voltage"=0.0, "battery24voltage"=0.0, "ErrorOutData"={"ErrorCode"=0, "ErrorMessage"=""}}, {"battery1voltage"=3.4816446, "battery2voltage"=3.4830422, "battery3voltage"=3.4783723, "battery4voltage"=3.4823694, "battery5voltage"=3.4844015, "battery6voltage"=0.0, "battery7voltage"=0.0, "battery8voltage"=0.0, "battery9voltage"=0.0, "battery10voltage"=0.0, "battery11voltage"=0.0, "battery12voltage"=0.0, "battery13voltage"=0.0, "battery14voltage"=0.0, "battery15voltage"=0.0, "battery16voltage"=0.0, "battery17voltage"=0.0, "battery18voltage"=0.0, "battery19voltage"=0.0, "battery20voltage"=0.0, "battery21voltage"=0.0, "battery22voltage"=0.0, "battery23voltage"=0.0, "battery24voltage"=0.0, "ErrorOutData"={"ErrorCode"=0, "ErrorMessage"=""}}, {"battery1voltage"=3.4816337, "battery2voltage"=3.483039, "battery3voltage"=3.4783669, "battery4voltage"=3.4823694, "battery5voltage"=3.4844108, "battery6voltage"=0.0, "battery7voltage"=0.0, "battery8voltage"=0.0, "battery9voltage"=0.0, "battery10voltage"=0.0, "battery11voltage"=0.0, "battery12voltage"=0.0, "battery13voltage"=0.0, "battery14voltage"=0.0, "battery15voltage"=0.0, "battery16voltage"=0.0, "battery17voltage"=0.0, "battery18voltage"=0.0, "battery19voltage"=0.0, "battery20voltage"=0.0, "battery21voltage"=0.0, "battery22voltage"=0.0, "battery23voltage"=0.0, "battery24voltage"=0.0, "ErrorOutData"={"ErrorCode"=0, "ErrorMessage"=""}}, {"battery1voltage"=3.4816325, "battery2voltage"=3.4830413, "battery3voltage"=3.4783652, "battery4voltage"=3.4823673, "battery5voltage"=3.4844015, "battery6voltage"=0.0, "battery7voltage"=0.0, "battery8voltage"=0.0, "battery9voltage"=0.0, "battery10voltage"=0.0, "battery11voltage"=0.0, "battery12voltage"=0.0, "battery13voltage"=0.0, "battery14voltage"=0.0, "battery15voltage"=0.0, "battery16voltage"=0.0, "battery17voltage"=0.0, "battery18voltage"=0.0, "battery19voltage"=0.0, "battery20voltage"=0.0, "battery21voltage"=0.0, "battery22voltage"=0.0, "battery23voltage"=0.0, "battery24voltage"=0.0, "ErrorOutData"={"ErrorCode"=0, "ErrorMessage"=""}}, {"battery1voltage"=3.4816356, "battery2voltage"=3.483046, "battery3voltage"=3.478368, "battery4voltage"=3.482366, "battery5voltage"=3.4844065, "battery6voltage"=0.0, "battery7voltage"=0.0, "battery8voltage"=0.0, "battery9voltage"=0.0, "battery10voltage"=0.0, "battery11voltage"=0.0, "battery12voltage"=0.0, "battery13voltage"=0.0, "battery14voltage"=0.0, "battery15voltage"=0.0, "battery16voltage"=0.0, "battery17voltage"=0.0, "battery18voltage"=0.0, "battery19voltage"=0.0, "battery20voltage"=0.0, "battery21voltage"=0.0, "battery22voltage"=0.0, "battery23voltage"=0.0, "battery24voltage"=0.0, "ErrorOutData"={"ErrorCode"=0, "ErrorMessage"=""}}, {"battery1voltage"=3.4816365, "battery2voltage"=3.4830458, "battery3voltage"=3.4783702, "battery4voltage"=3.4823682, "battery5voltage"=3.484401, "battery6voltage"=0.0, "battery7voltage"=0.0, "battery8voltage"=0.0, "battery9voltage"=0.0, "battery10voltage"=0.0, "battery11voltage"=0.0, "battery12voltage"=0.0, "battery13voltage"=0.0, "battery14voltage"=0.0, "battery15voltage"=0.0, "battery16voltage"=0.0, "battery17voltage"=0.0, "battery18voltage"=0.0, "battery19voltage"=0.0, "battery20voltage"=0.0, "battery21voltage"=0.0, "battery22voltage"=0.0, "battery23voltage"=0.0, "battery24voltage"=0.0, "ErrorOutData"={"ErrorCode"=0, "ErrorMessage"=""}}, {"battery1voltage"=3.4816322, "battery2voltage"=3.4830444, "battery3voltage"=3.4783752, "battery4voltage"=3.4823666, "battery5voltage"=3.4844022, "battery6voltage"=0.0, "battery7voltage"=0.0, "battery8voltage"=0.0, "battery9voltage"=0.0, "battery10voltage"=0.0, "battery11voltage"=0.0, "battery12voltage"=0.0, "battery13voltage"=0.0, "battery14voltage"=0.0, "battery15voltage"=0.0, "battery16voltage"=0.0, "battery17voltage"=0.0, "battery18voltage"=0.0, "battery19voltage"=0.0, "battery20voltage"=0.0, "battery21voltage"=0.0, "battery22voltage"=0.0, "battery23voltage"=0.0, "battery24voltage"=0.0, "ErrorOutData"={"ErrorCode"=0, "ErrorMessage"=""}}, {"battery1voltage"=3.4816391, "battery2voltage"=3.4830413, "battery3voltage"=3.4783728, "battery4voltage"=3.4823685, "battery5voltage"=3.4844005, "battery6voltage"=0.0, "battery7voltage"=0.0, "battery8voltage"=0.0, "battery9voltage"=0.0, "battery10voltage"=0.0, "battery11voltage"=0.0, "battery12voltage"=0.0, "battery13voltage"=0.0, "battery14voltage"=0.0, "battery15voltage"=0.0, "battery16voltage"=0.0, "battery17voltage"=0.0, "battery18voltage"=0.0, "battery19voltage"=0.0, "battery20voltage"=0.0, "battery21voltage"=0.0, "battery22voltage"=0.0, "battery23voltage"=0.0, "battery24voltage"=0.0, "ErrorOutData"={"ErrorCode"=0, "ErrorMessage"=""}}, {"battery1voltage"=3.481637, "battery2voltage"=3.4830399, "battery3voltage"=3.4783745, "battery4voltage"=3.482366, "battery5voltage"=3.4844046, "battery6voltage"=0.0, "battery7voltage"=0.0, "battery8voltage"=0.0, "battery9voltage"=0.0, "battery10voltage"=0.0, "battery11voltage"=0.0, "battery12voltage"=0.0, "battery13voltage"=0.0, "battery14voltage"=0.0, "battery15voltage"=0.0, "battery16voltage"=0.0, "battery17voltage"=0.0, "battery18voltage"=0.0, "battery19voltage"=0.0, "battery20voltage"=0.0, "battery21voltage"=0.0, "battery22voltage"=0.0, "battery23voltage"=0.0, "battery24voltage"=0.0, "ErrorOutData"={"ErrorCode"=0, "ErrorMessage"=""}}, {"battery1voltage"=3.4816382, "battery2voltage"=3.4830427, "battery3voltage"=3.4783697, "battery4voltage"=3.48237, "battery5voltage"=3.4844015, "battery6voltage"=0.0, "battery7voltage"=0.0, "battery8voltage"=0.0, "battery9voltage"=0.0, "battery10voltage"=0.0, "battery11voltage"=0.0, "battery12voltage"=0.0, "battery13voltage"=0.0, "battery14voltage"=0.0, "battery15voltage"=0.0, "battery16voltage"=0.0, "battery17voltage"=0.0, "battery18voltage"=0.0, "battery19voltage"=0.0, "battery20voltage"=0.0, "battery21voltage"=0.0, "battery22voltage"=0.0, "battery23voltage"=0.0, "battery24voltage"=0.0, "ErrorOutData"={"ErrorCode"=0, "ErrorMessage"=""}}, {"battery1voltage"=3.4816358, "battery2voltage"=3.4830434, "battery3voltage"=3.4783742, "battery4voltage"=3.4823682, "battery5voltage"=3.4844017, "battery6voltage"=0.0, "battery7voltage"=0.0, "battery8voltage"=0.0, "battery9voltage"=0.0, "battery10voltage"=0.0, "battery11voltage"=0.0, "battery12voltage"=0.0, "battery13voltage"=0.0, "battery14voltage"=0.0, "battery15voltage"=0.0, "battery16voltage"=0.0, "battery17voltage"=0.0, "battery18voltage"=0.0, "battery19voltage"=0.0, "battery20voltage"=0.0, "battery21voltage"=0.0, "battery22voltage"=0.0, "battery23voltage"=0.0, "battery24voltage"=0.0, "ErrorOutData"={"ErrorCode"=0, "ErrorMessage"=""}}, {"battery1voltage"=3.4816394, "battery2voltage"=3.483044, "battery3voltage"=3.4783754, "battery4voltage"=3.4823692, "battery5voltage"=3.4844005, "battery6voltage"=0.0, "battery7voltage"=0.0, "battery8voltage"=0.0, "battery9voltage"=0.0, "battery10voltage"=0.0, "battery11voltage"=0.0, "battery12voltage"=0.0, "battery13voltage"=0.0, "battery14voltage"=0.0, "battery15voltage"=0.0, "battery16voltage"=0.0, "battery17voltage"=0.0, "battery18voltage"=0.0, "battery19voltage"=0.0, "battery20voltage"=0.0, "battery21voltage"=0.0, "battery22voltage"=0.0, "battery23voltage"=0.0, "battery24voltage"=0.0, "ErrorOutData"={"ErrorCode"=0, "ErrorMessage"=""}}, {"battery1voltage"=3.481634, "battery2voltage"=3.4830408, "battery3voltage"=3.4783669, "battery4voltage"=3.4823651, "battery5voltage"=3.4844038, "battery6voltage"=0.0, "battery7voltage"=0.0, "battery8voltage"=0.0, "battery9voltage"=0.0, "battery10voltage"=0.0, "battery11voltage"=0.0, "battery12voltage"=0.0, "battery13voltage"=0.0, "battery14voltage"=0.0, "battery15voltage"=0.0, "battery16voltage"=0.0, "battery17voltage"=0.0, "battery18voltage"=0.0, "battery19voltage"=0.0, "battery20voltage"=0.0, "battery21voltage"=0.0, "battery22voltage"=0.0, "battery23voltage"=0.0, "battery24voltage"=0.0, "ErrorOutData"={"ErrorCode"=0, "ErrorMessage"=""}}, {"battery1voltage"=3.4816377, "battery2voltage"=3.4830425, "battery3voltage"=3.4783716, "battery4voltage"=3.482369, "battery5voltage"=3.484401, "battery6voltage"=0.0, "battery7voltage"=0.0, "battery8voltage"=0.0, "battery9voltage"=0.0, "battery10voltage"=0.0, "battery11voltage"=0.0, "battery12voltage"=0.0, "battery13voltage"=0.0, "battery14voltage"=0.0, "battery15voltage"=0.0, "battery16voltage"=0.0, "battery17voltage"=0.0, "battery18voltage"=0.0, "battery19voltage"=0.0, "battery20voltage"=0.0, "battery21voltage"=0.0, "battery22voltage"=0.0, "battery23voltage"=0.0, "battery24voltage"=0.0, "ErrorOutData"={"ErrorCode"=0, "ErrorMessage"=""}}, {"battery1voltage"=3.481638, "battery2voltage"=3.483039, "battery3voltage"=3.4783654, "battery4voltage"=3.48237, "battery5voltage"=3.4844065, "battery6voltage"=0.0, "battery7voltage"=0.0, "battery8voltage"=0.0, "battery9voltage"=0.0, "battery10voltage"=0.0, "battery11voltage"=0.0, "battery12voltage"=0.0, "battery13voltage"=0.0, "battery14voltage"=0.0, "battery15voltage"=0.0, "battery16voltage"=0.0, "battery17voltage"=0.0, "battery18voltage"=0.0, "battery19voltage"=0.0, "battery20voltage"=0.0, "battery21voltage"=0.0, "battery22voltage"=0.0, "battery23voltage"=0.0, "battery24voltage"=0.0, "ErrorOutData"={"ErrorCode"=0, "ErrorMessage"=""}}, {"battery1voltage"=3.4816375, "battery2voltage"=3.4830475, "battery3voltage"=3.4783783, "battery4voltage"=3.4823647, "battery5voltage"=3.4844038, "battery6voltage"=0.0, "battery7voltage"=0.0, "battery8voltage"=0.0, "battery9voltage"=0.0, "battery10voltage"=0.0, "battery11voltage"=0.0, "battery12voltage"=0.0, "battery13voltage"=0.0, "battery14voltage"=0.0, "battery15voltage"=0.0, "battery16voltage"=0.0, "battery17voltage"=0.0, "battery18voltage"=0.0, "battery19voltage"=0.0, "battery20voltage"=0.0, "battery21voltage"=0.0, "battery22voltage"=0.0, "battery23voltage"=0.0, "battery24voltage"=0.0, "ErrorOutData"={"ErrorCode"=0, "ErrorMessage"=""}}, {"battery1voltage"=3.4816403, "battery2voltage"=3.4830472, "battery3voltage"=3.4783723, "battery4voltage"=3.4823694, "battery5voltage"=3.4843976, "battery6voltage"=0.0, "battery7voltage"=0.0, "battery8voltage"=0.0, "battery9voltage"=0.0, "battery10voltage"=0.0, "battery11voltage"=0.0, "battery12voltage"=0.0, "battery13voltage"=0.0, "battery14voltage"=0.0, "battery15voltage"=0.0, "battery16voltage"=0.0, "battery17voltage"=0.0, "battery18voltage"=0.0, "battery19voltage"=0.0, "battery20voltage"=0.0, "battery21voltage"=0.0, "battery22voltage"=0.0, "battery23voltage"=0.0, "battery24voltage"=0.0, "ErrorOutData"={"ErrorCode"=0, "ErrorMessage"=""}}, {"battery1voltage"=3.4816413, "battery2voltage"=3.4830482, "battery3voltage"=3.4783695, "battery4voltage"=3.482367, "battery5voltage"=3.4844043, "battery6voltage"=0.0, "battery7voltage"=0.0, "battery8voltage"=0.0, "battery9voltage"=0.0, "battery10voltage"=0.0, "battery11voltage"=0.0, "battery12voltage"=0.0, "battery13voltage"=0.0, "battery14voltage"=0.0, "battery15voltage"=0.0, "battery16voltage"=0.0, "battery17voltage"=0.0, "battery18voltage"=0.0, "battery19voltage"=0.0, "battery20voltage"=0.0, "battery21voltage"=0.0, "battery22voltage"=0.0, "battery23voltage"=0.0, "battery24voltage"=0.0, "ErrorOutData"={"ErrorCode"=0, "ErrorMessage"=""}}, {"battery1voltage"=3.4816382, "battery2voltage"=3.4830446, "battery3voltage"=3.4783735, "battery4voltage"=3.4823701, "battery5voltage"=3.4843962, "battery6voltage"=0.0, "battery7voltage"=0.0, "battery8voltage"=0.0, "battery9voltage"=0.0, "battery10voltage"=0.0, "battery11voltage"=0.0, "battery12voltage"=0.0, "battery13voltage"=0.0, "battery14voltage"=0.0, "battery15voltage"=0.0, "battery16voltage"=0.0, "battery17voltage"=0.0, "battery18voltage"=0.0, "battery19voltage"=0.0, "battery20voltage"=0.0, "battery21voltage"=0.0, "battery22voltage"=0.0, "battery23voltage"=0.0, "battery24voltage"=0.0, "ErrorOutData"={"ErrorCode"=0, "ErrorMessage"=""}}, {"battery1voltage"=3.481636, "battery2voltage"=3.4830408, "battery3voltage"=3.4783683, "battery4voltage"=3.482367, "battery5voltage"=3.484406, "battery6voltage"=0.0, "battery7voltage"=0.0, "battery8voltage"=0.0, "battery9voltage"=0.0, "battery10voltage"=0.0, "battery11voltage"=0.0, "battery12voltage"=0.0, "battery13voltage"=0.0, "battery14voltage"=0.0, "battery15voltage"=0.0, "battery16voltage"=0.0, "battery17voltage"=0.0, "battery18voltage"=0.0, "battery19voltage"=0.0, "battery20voltage"=0.0, "battery21voltage"=0.0, "battery22voltage"=0.0, "battery23voltage"=0.0, "battery24voltage"=0.0, "ErrorOutData"={"ErrorCode"=0, "ErrorMessage"=""}}, {"battery1voltage"=3.4816418, "battery2voltage"=3.4830418, "battery3voltage"=3.4783669, "battery4voltage"=3.482368, "battery5voltage"=3.484411, "battery6voltage"=0.0, "battery7voltage"=0.0, "battery8voltage"=0.0, "battery9voltage"=0.0, "battery10voltage"=0.0, "battery11voltage"=0.0, "battery12voltage"=0.0, "battery13voltage"=0.0, "battery14voltage"=0.0, "battery15voltage"=0.0, "battery16voltage"=0.0, "battery17voltage"=0.0, "battery18voltage"=0.0, "battery19voltage"=0.0, "battery20voltage"=0.0, "battery21voltage"=0.0, "battery22voltage"=0.0, "battery23voltage"=0.0, "battery24voltage"=0.0, "ErrorOutData"={"ErrorCode"=0, "ErrorMessage"=""}}, {"battery1voltage"=3.4816382, "battery2voltage"=3.483042, "battery3voltage"=3.4783723, "battery4voltage"=3.4823678, "battery5voltage"=3.4844053, "battery6voltage"=0.0, "battery7voltage"=0.0, "battery8voltage"=0.0, "battery9voltage"=0.0, "battery10voltage"=0.0, "battery11voltage"=0.0, "battery12voltage"=0.0, "battery13voltage"=0.0, "battery14voltage"=0.0, "battery15voltage"=0.0, "battery16voltage"=0.0, "battery17voltage"=0.0, "battery18voltage"=0.0, "battery19voltage"=0.0, "battery20voltage"=0.0, "battery21voltage"=0.0, "battery22voltage"=0.0, "battery23voltage"=0.0, "battery24voltage"=0.0, "ErrorOutData"={"ErrorCode"=0, "ErrorMessage"=""}}, {"battery1voltage"=3.4816322, "battery2voltage"=3.4830375, "battery3voltage"=3.478369, "battery4voltage"=3.4823651, "battery5voltage"=3.484405, "battery6voltage"=0.0, "battery7voltage"=0.0, "battery8voltage"=0.0, "battery9voltage"=0.0, "battery10voltage"=0.0, "battery11voltage"=0.0, "battery12voltage"=0.0, "battery13voltage"=0.0, "battery14voltage"=0.0, "battery15voltage"=0.0, "battery16voltage"=0.0, "battery17voltage"=0.0, "battery18voltage"=0.0, "battery19voltage"=0.0, "battery20voltage"=0.0, "battery21voltage"=0.0, "battery22voltage"=0.0, "battery23voltage"=0.0, "battery24voltage"=0.0, "ErrorOutData"={"ErrorCode"=0, "ErrorMessage"=""}}, {"battery1voltage"=3.4816375, "battery2voltage"=3.4830382, "battery3voltage"=3.478371, "battery4voltage"=3.4823635, "battery5voltage"=3.4844062, "battery6voltage"=0.0, "battery7voltage"=0.0, "battery8voltage"=0.0, "battery9voltage"=0.0, "battery10voltage"=0.0, "battery11voltage"=0.0, "battery12voltage"=0.0, "battery13voltage"=0.0, "battery14voltage"=0.0, "battery15voltage"=0.0, "battery16voltage"=0.0, "battery17voltage"=0.0, "battery18voltage"=0.0, "battery19voltage"=0.0, "battery20voltage"=0.0, "battery21voltage"=0.0, "battery22voltage"=0.0, "battery23voltage"=0.0, "battery24voltage"=0.0, "ErrorOutData"={"ErrorCode"=0, "ErrorMessage"=""}}, {"battery1voltage"=3.4816356, "battery2voltage"=3.4830391, "battery3voltage"=3.4783695, "battery4voltage"=3.482366, "battery5voltage"=3.4844058, "battery6voltage"=0.0, "battery7voltage"=0.0, "battery8voltage"=0.0, "battery9voltage"=0.0, "battery10voltage"=0.0, "battery11voltage"=0.0, "battery12voltage"=0.0, "battery13voltage"=0.0, "battery14voltage"=0.0, "battery15voltage"=0.0, "battery16voltage"=0.0, "battery17voltage"=0.0, "battery18voltage"=0.0, "battery19voltage"=0.0, "battery20voltage"=0.0, "battery21voltage"=0.0, "battery22voltage"=0.0, "battery23voltage"=0.0, "battery24voltage"=0.0, "ErrorOutData"={"ErrorCode"=0, "ErrorMessage"=""}}, {"battery1voltage"=3.481642, "battery2voltage"=3.483044, "battery3voltage"=3.4783707, "battery4voltage"=3.482366, "battery5voltage"=3.4844027, "battery6voltage"=0.0, "battery7voltage"=0.0, "battery8voltage"=0.0, "battery9voltage"=0.0, "battery10voltage"=0.0, "battery11voltage"=0.0, "battery12voltage"=0.0, "battery13voltage"=0.0, "battery14voltage"=0.0, "battery15voltage"=0.0, "battery16voltage"=0.0, "battery17voltage"=0.0, "battery18voltage"=0.0, "battery19voltage"=0.0, "battery20voltage"=0.0, "battery21voltage"=0.0, "battery22voltage"=0.0, "battery23voltage"=0.0, "battery24voltage"=0.0, "ErrorOutData"={"ErrorCode"=0, "ErrorMessage"=""}}, {"battery1voltage"=3.4816384, "battery2voltage"=3.483043, "battery3voltage"=3.4783728, "battery4voltage"=3.4823685, "battery5voltage"=3.4844081, "battery6voltage"=0.0, "battery7voltage"=0.0, "battery8voltage"=0.0, "battery9voltage"=0.0, "battery10voltage"=0.0, "battery11voltage"=0.0, "battery12voltage"=0.0, "battery13voltage"=0.0, "battery14voltage"=0.0, "battery15voltage"=0.0, "battery16voltage"=0.0, "battery17voltage"=0.0, "battery18voltage"=0.0, "battery19voltage"=0.0, "battery20voltage"=0.0, "battery21voltage"=0.0, "battery22voltage"=0.0, "battery23voltage"=0.0, "battery24voltage"=0.0, "ErrorOutData"={"ErrorCode"=0, "ErrorMessage"=""}}, {"battery1voltage"=3.4816382, "battery2voltage"=3.4830403, "battery3voltage"=3.4783695, "battery4voltage"=3.4823694, "battery5voltage"=3.4844038, "battery6voltage"=0.0, "battery7voltage"=0.0, "battery8voltage"=0.0, "battery9voltage"=0.0, "battery10voltage"=0.0, "battery11voltage"=0.0, "battery12voltage"=0.0, "battery13voltage"=0.0, "battery14voltage"=0.0, "battery15voltage"=0.0, "battery16voltage"=0.0, "battery17voltage"=0.0, "battery18voltage"=0.0, "battery19voltage"=0.0, "battery20voltage"=0.0, "battery21voltage"=0.0, "battery22voltage"=0.0, "battery23voltage"=0.0, "battery24voltage"=0.0, "ErrorOutData"={"ErrorCode"=0, "ErrorMessage"=""}}, {"battery1voltage"=3.4816365, "battery2voltage"=3.4830384, "battery3voltage"=3.4783714, "battery4voltage"=3.4823656, "battery5voltage"=3.484406, "battery6voltage"=0.0, "battery7voltage"=0.0, "battery8voltage"=0.0, "battery9voltage"=0.0, "battery10voltage"=0.0, "battery11voltage"=0.0, "battery12voltage"=0.0, "battery13voltage"=0.0, "battery14voltage"=0.0, "battery15voltage"=0.0, "battery16voltage"=0.0, "battery17voltage"=0.0, "battery18voltage"=0.0, "battery19voltage"=0.0, "battery20voltage"=0.0, "battery21voltage"=0.0, "battery22voltage"=0.0, "battery23voltage"=0.0, "battery24voltage"=0.0, "ErrorOutData"={"ErrorCode"=0, "ErrorMessage"=""}}, {"battery1voltage"=3.481637, "battery2voltage"=3.4830413, "battery3voltage"=3.478368, "battery4voltage"=3.4823709, "battery5voltage"=3.4844017, "battery6voltage"=0.0, "battery7voltage"=0.0, "battery8voltage"=0.0, "battery9voltage"=0.0, "battery10voltage"=0.0, "battery11voltage"=0.0, "battery12voltage"=0.0, "battery13voltage"=0.0, "battery14voltage"=0.0, "battery15voltage"=0.0, "battery16voltage"=0.0, "battery17voltage"=0.0, "battery18voltage"=0.0, "battery19voltage"=0.0, "battery20voltage"=0.0, "battery21voltage"=0.0, "battery22voltage"=0.0, "battery23voltage"=0.0, "battery24voltage"=0.0, "ErrorOutData"={"ErrorCode"=0, "ErrorMessage"=""}}, {"battery1voltage"=3.4816353, "battery2voltage"=3.483047, "battery3voltage"=3.4783692, "battery4voltage"=3.4823658, "battery5voltage"=3.4844015, "battery6voltage"=0.0, "battery7voltage"=0.0, "battery8voltage"=0.0, "battery9voltage"=0.0, "battery10voltage"=0.0, "battery11voltage"=0.0, "battery12voltage"=0.0, "battery13voltage"=0.0, "battery14voltage"=0.0, "battery15voltage"=0.0, "battery16voltage"=0.0, "battery17voltage"=0.0, "battery18voltage"=0.0, "battery19voltage"=0.0, "battery20voltage"=0.0, "battery21voltage"=0.0, "battery22voltage"=0.0, "battery23voltage"=0.0, "battery24voltage"=0.0, "ErrorOutData"={"ErrorCode"=0, "ErrorMessage"=""}}, {"battery1voltage"=3.4816394, "battery2voltage"=3.4830372, "battery3voltage"=3.4783678, "battery4voltage"=3.4823673, "battery5voltage"=3.4844034, "battery6voltage"=0.0, "battery7voltage"=0.0, "battery8voltage"=0.0, "battery9voltage"=0.0, "battery10voltage"=0.0, "battery11voltage"=0.0, "battery12voltage"=0.0, "battery13voltage"=0.0, "battery14voltage"=0.0, "battery15voltage"=0.0, "battery16voltage"=0.0, "battery17voltage"=0.0, "battery18voltage"=0.0, "battery19voltage"=0.0, "battery20voltage"=0.0, "battery21voltage"=0.0, "battery22voltage"=0.0, "battery23voltage"=0.0, "battery24voltage"=0.0, "ErrorOutData"={"ErrorCode"=0, "ErrorMessage"=""}}, {"battery1voltage"=3.4816382, "battery2voltage"=3.4830408, "battery3voltage"=3.4783669, "battery4voltage"=3.4823682, "battery5voltage"=3.4844112, "battery6voltage"=0.0, "battery7voltage"=0.0, "battery8voltage"=0.0, "battery9voltage"=0.0, "battery10voltage"=0.0, "battery11voltage"=0.0, "battery12voltage"=0.0, "battery13voltage"=0.0, "battery14voltage"=0.0, "battery15voltage"=0.0, "battery16voltage"=0.0, "battery17voltage"=0.0, "battery18voltage"=0.0, "battery19voltage"=0.0, "battery20voltage"=0.0, "battery21voltage"=0.0, "battery22voltage"=0.0, "battery23voltage"=0.0, "battery24voltage"=0.0, "ErrorOutData"={"ErrorCode"=0, "ErrorMessage"=""}}, {"battery1voltage"=3.4816437, "battery2voltage"=3.483042, "battery3voltage"=3.4783704, "battery4voltage"=3.4823694, "battery5voltage"=3.4844022, "battery6voltage"=0.0, "battery7voltage"=0.0, "battery8voltage"=0.0, "battery9voltage"=0.0, "battery10voltage"=0.0, "battery11voltage"=0.0, "battery12voltage"=0.0, "battery13voltage"=0.0, "battery14voltage"=0.0, "battery15voltage"=0.0, "battery16voltage"=0.0, "battery17voltage"=0.0, "battery18voltage"=0.0, "battery19voltage"=0.0, "battery20voltage"=0.0, "battery21voltage"=0.0, "battery22voltage"=0.0, "battery23voltage"=0.0, "battery24voltage"=0.0, "ErrorOutData"={"ErrorCode"=0, "ErrorMessage"=""}}, {"battery1voltage"=3.4816415, "battery2voltage"=3.483049, "battery3voltage"=3.4783702, "battery4voltage"=3.482367, "battery5voltage"=3.4844034, "battery6voltage"=0.0, "battery7voltage"=0.0, "battery8voltage"=0.0, "battery9voltage"=0.0, "battery10voltage"=0.0, "battery11voltage"=0.0, "battery12voltage"=0.0, "battery13voltage"=0.0, "battery14voltage"=0.0, "battery15voltage"=0.0, "battery16voltage"=0.0, "battery17voltage"=0.0, "battery18voltage"=0.0, "battery19voltage"=0.0, "battery20voltage"=0.0, "battery21voltage"=0.0, "battery22voltage"=0.0, "battery23voltage"=0.0, "battery24voltage"=0.0, "ErrorOutData"={"ErrorCode"=0, "ErrorMessage"=""}}, {"battery1voltage"=3.4816375, "battery2voltage"=3.4830372, "battery3voltage"=3.4783695, "battery4voltage"=3.482367, "battery5voltage"=3.4844053, "battery6voltage"=0.0, "battery7voltage"=0.0, "battery8voltage"=0.0, "battery9voltage"=0.0, "battery10voltage"=0.0, "battery11voltage"=0.0, "battery12voltage"=0.0, "battery13voltage"=0.0, "battery14voltage"=0.0, "battery15voltage"=0.0, "battery16voltage"=0.0, "battery17voltage"=0.0, "battery18voltage"=0.0, "battery19voltage"=0.0, "battery20voltage"=0.0, "battery21voltage"=0.0, "battery22voltage"=0.0, "battery23voltage"=0.0, "battery24voltage"=0.0, "ErrorOutData"={"ErrorCode"=0, "ErrorMessage"=""}}, {"battery1voltage"=3.4816375, "battery2voltage"=3.483041, "battery3voltage"=3.4783754, "battery4voltage"=3.4823663, "battery5voltage"=3.4843974, "battery6voltage"=0.0, "battery7voltage"=0.0, "battery8voltage"=0.0, "battery9voltage"=0.0, "battery10voltage"=0.0, "battery11voltage"=0.0, "battery12voltage"=0.0, "battery13voltage"=0.0, "battery14voltage"=0.0, "battery15voltage"=0.0, "battery16voltage"=0.0, "battery17voltage"=0.0, "battery18voltage"=0.0, "battery19voltage"=0.0, "battery20voltage"=0.0, "battery21voltage"=0.0, "battery22voltage"=0.0, "battery23voltage"=0.0, "battery24voltage"=0.0, "ErrorOutData"={"ErrorCode"=0, "ErrorMessage"=""}}, {"battery1voltage"=3.4816418, "battery2voltage"=3.4830368, "battery3voltage"=3.4783688, "battery4voltage"=3.4823596, "battery5voltage"=3.484408, "battery6voltage"=0.0, "battery7voltage"=0.0, "battery8voltage"=0.0, "battery9voltage"=0.0, "battery10voltage"=0.0, "battery11voltage"=0.0, "battery12voltage"=0.0, "battery13voltage"=0.0, "battery14voltage"=0.0, "battery15voltage"=0.0, "battery16voltage"=0.0, "battery17voltage"=0.0, "battery18voltage"=0.0, "battery19voltage"=0.0, "battery20voltage"=0.0, "battery21voltage"=0.0, "battery22voltage"=0.0, "battery23voltage"=0.0, "battery24voltage"=0.0, "ErrorOutData"={"ErrorCode"=0, "ErrorMessage"=""}}, {"battery1voltage"=3.4816406, "battery2voltage"=3.4830463, "battery3voltage"=3.4783697, "battery4voltage"=3.4823644, "battery5voltage"=3.484399, "battery6voltage"=0.0, "battery7voltage"=0.0, "battery8voltage"=0.0, "battery9voltage"=0.0, "battery10voltage"=0.0, "battery11voltage"=0.0, "battery12voltage"=0.0, "battery13voltage"=0.0, "battery14voltage"=0.0, "battery15voltage"=0.0, "battery16voltage"=0.0, "battery17voltage"=0.0, "battery18voltage"=0.0, "battery19voltage"=0.0, "battery20voltage"=0.0, "battery21voltage"=0.0, "battery22voltage"=0.0, "battery23voltage"=0.0, "battery24voltage"=0.0, "ErrorOutData"={"ErrorCode"=0, "ErrorMessage"=""}}, {"battery1voltage"=3.4816408, "battery2voltage"=3.4830425, "battery3voltage"=3.4783728, "battery4voltage"=3.4823697, "battery5voltage"=3.484402, "battery6voltage"=0.0, "battery7voltage"=0.0, "battery8voltage"=0.0, "battery9voltage"=0.0, "battery10voltage"=0.0, "battery11voltage"=0.0, "battery12voltage"=0.0, "battery13voltage"=0.0, "battery14voltage"=0.0, "battery15voltage"=0.0, "battery16voltage"=0.0, "battery17voltage"=0.0, "battery18voltage"=0.0, "battery19voltage"=0.0, "battery20voltage"=0.0, "battery21voltage"=0.0, "battery22voltage"=0.0, "battery23voltage"=0.0, "battery24voltage"=0.0, "ErrorOutData"={"ErrorCode"=0, "ErrorMessage"=""}}, {"battery1voltage"=3.4816415, "battery2voltage"=3.483043, "battery3voltage"=3.4783738, "battery4voltage"=3.4823694, "battery5voltage"=3.4843986, "battery6voltage"=0.0, "battery7voltage"=0.0, "battery8voltage"=0.0, "battery9voltage"=0.0, "battery10voltage"=0.0, "battery11voltage"=0.0, "battery12voltage"=0.0, "battery13voltage"=0.0, "battery14voltage"=0.0, "battery15voltage"=0.0, "battery16voltage"=0.0, "battery17voltage"=0.0, "battery18voltage"=0.0, "battery19voltage"=0.0, "battery20voltage"=0.0, "battery21voltage"=0.0, "battery22voltage"=0.0, "battery23voltage"=0.0, "battery24voltage"=0.0, "ErrorOutData"={"ErrorCode"=0, "ErrorMessage"=""}}, {"battery1voltage"=3.4816391, "battery2voltage"=3.4830441, "battery3voltage"=3.4783683, "battery4voltage"=3.482368, "battery5voltage"=3.4843988, "battery6voltage"=0.0, "battery7voltage"=0.0, "battery8voltage"=0.0, "battery9voltage"=0.0, "battery10voltage"=0.0, "battery11voltage"=0.0, "battery12voltage"=0.0, "battery13voltage"=0.0, "battery14voltage"=0.0, "battery15voltage"=0.0, "battery16voltage"=0.0, "battery17voltage"=0.0, "battery18voltage"=0.0, "battery19voltage"=0.0, "battery20voltage"=0.0, "battery21voltage"=0.0, "battery22voltage"=0.0, "battery23voltage"=0.0, "battery24voltage"=0.0, "ErrorOutData"={"ErrorCode"=0, "ErrorMessage"=""}}, {"battery1voltage"=3.4816394, "battery2voltage"=3.4830391, "battery3voltage"=3.4783738, "battery4voltage"=3.4823668, "battery5voltage"=3.4844034, "battery6voltage"=0.0, "battery7voltage"=0.0, "battery8voltage"=0.0, "battery9voltage"=0.0, "battery10voltage"=0.0, "battery11voltage"=0.0, "battery12voltage"=0.0, "battery13voltage"=0.0, "battery14voltage"=0.0, "battery15voltage"=0.0, "battery16voltage"=0.0, "battery17voltage"=0.0, "battery18voltage"=0.0, "battery19voltage"=0.0, "battery20voltage"=0.0, "battery21voltage"=0.0, "battery22voltage"=0.0, "battery23voltage"=0.0, "battery24voltage"=0.0, "ErrorOutData"={"ErrorCode"=0, "ErrorMessage"=""}}, {"battery1voltage"=3.4816334, "battery2voltage"=3.4830399, "battery3voltage"=3.478371, "battery4voltage"=3.4823647, "battery5voltage"=3.4844007, "battery6voltage"=0.0, "battery7voltage"=0.0, "battery8voltage"=0.0, "battery9voltage"=0.0, "battery10voltage"=0.0, "battery11voltage"=0.0, "battery12voltage"=0.0, "battery13voltage"=0.0, "battery14voltage"=0.0, "battery15voltage"=0.0, "battery16voltage"=0.0, "battery17voltage"=0.0, "battery18voltage"=0.0, "battery19voltage"=0.0, "battery20voltage"=0.0, "battery21voltage"=0.0, "battery22voltage"=0.0, "battery23voltage"=0.0, "battery24voltage"=0.0, "ErrorOutData"={"ErrorCode"=0, "ErrorMessage"=""}}, {"battery1voltage"=3.48164, "battery2voltage"=3.4830377, "battery3voltage"=3.4783707, "battery4voltage"=3.4823644, "battery5voltage"=3.484406, "battery6voltage"=0.0, "battery7voltage"=0.0, "battery8voltage"=0.0, "battery9voltage"=0.0, "battery10voltage"=0.0, "battery11voltage"=0.0, "battery12voltage"=0.0, "battery13voltage"=0.0, "battery14voltage"=0.0, "battery15voltage"=0.0, "battery16voltage"=0.0, "battery17voltage"=0.0, "battery18voltage"=0.0, "battery19voltage"=0.0, "battery20voltage"=0.0, "battery21voltage"=0.0, "battery22voltage"=0.0, "battery23voltage"=0.0, "battery24voltage"=0.0, "ErrorOutData"={"ErrorCode"=0, "ErrorMessage"=""}}, {"battery1voltage"=3.4816394, "battery2voltage"=3.4830437, "battery3voltage"=3.4783745, "battery4voltage"=3.482364, "battery5voltage"=3.4843996, "battery6voltage"=0.0, "battery7voltage"=0.0, "battery8voltage"=0.0, "battery9voltage"=0.0, "battery10voltage"=0.0, "battery11voltage"=0.0, "battery12voltage"=0.0, "battery13voltage"=0.0, "battery14voltage"=0.0, "battery15voltage"=0.0, "battery16voltage"=0.0, "battery17voltage"=0.0, "battery18voltage"=0.0, "battery19voltage"=0.0, "battery20voltage"=0.0, "battery21voltage"=0.0, "battery22voltage"=0.0, "battery23voltage"=0.0, "battery24voltage"=0.0, "ErrorOutData"={"ErrorCode"=0, "ErrorMessage"=""}}, {"battery1voltage"=3.481636, "battery2voltage"=3.48304, "battery3voltage"=3.4783669, "battery4voltage"=3.4823663, "battery5voltage"=3.484407, "battery6voltage"=0.0, "battery7voltage"=0.0, "battery8voltage"=0.0, "battery9voltage"=0.0, "battery10voltage"=0.0, "battery11voltage"=0.0, "battery12voltage"=0.0, "battery13voltage"=0.0, "battery14voltage"=0.0, "battery15voltage"=0.0, "battery16voltage"=0.0, "battery17voltage"=0.0, "battery18voltage"=0.0, "battery19voltage"=0.0, "battery20voltage"=0.0, "battery21voltage"=0.0, "battery22voltage"=0.0, "battery23voltage"=0.0, "battery24voltage"=0.0, "ErrorOutData"={"ErrorCode"=0, "ErrorMessage"=""}}, {"battery1voltage"=3.4816372, "battery2voltage"=3.4830394, "battery3voltage"=3.478374, "battery4voltage"=3.4823635, "battery5voltage"=3.4844058, "battery6voltage"=0.0, "battery7voltage"=0.0, "battery8voltage"=0.0, "battery9voltage"=0.0, "battery10voltage"=0.0, "battery11voltage"=0.0, "battery12voltage"=0.0, "battery13voltage"=0.0, "battery14voltage"=0.0, "battery15voltage"=0.0, "battery16voltage"=0.0, "battery17voltage"=0.0, "battery18voltage"=0.0, "battery19voltage"=0.0, "battery20voltage"=0.0, "battery21voltage"=0.0, "battery22voltage"=0.0, "battery23voltage"=0.0, "battery24voltage"=0.0, "ErrorOutData"={"ErrorCode"=0, "ErrorMessage"=""}}, {"battery1voltage"=3.4816384, "battery2voltage"=3.483045, "battery3voltage"=3.4783728, "battery4voltage"=3.4823613, "battery5voltage"=3.4844007, "battery6voltage"=0.0, "battery7voltage"=0.0, "battery8voltage"=0.0, "battery9voltage"=0.0, "battery10voltage"=0.0, "battery11voltage"=0.0, "battery12voltage"=0.0, "battery13voltage"=0.0, "battery14voltage"=0.0, "battery15voltage"=0.0, "battery16voltage"=0.0, "battery17voltage"=0.0, "battery18voltage"=0.0, "battery19voltage"=0.0, "battery20voltage"=0.0, "battery21voltage"=0.0, "battery22voltage"=0.0, "battery23voltage"=0.0, "battery24voltage"=0.0, "ErrorOutData"={"ErrorCode"=0, "ErrorMessage"=""}}, {"battery1voltage"=3.4816353, "battery2voltage"=3.4830418, "battery3voltage"=3.4783728, "battery4voltage"=3.482367, "battery5voltage"=3.4844005, "battery6voltage"=0.0, "battery7voltage"=0.0, "battery8voltage"=0.0, "battery9voltage"=0.0, "battery10voltage"=0.0, "battery11voltage"=0.0, "battery12voltage"=0.0, "battery13voltage"=0.0, "battery14voltage"=0.0, "battery15voltage"=0.0, "battery16voltage"=0.0, "battery17voltage"=0.0, "battery18voltage"=0.0, "battery19voltage"=0.0, "battery20voltage"=0.0, "battery21voltage"=0.0, "battery22voltage"=0.0, "battery23voltage"=0.0, "battery24voltage"=0.0, "ErrorOutData"={"ErrorCode"=0, "ErrorMessage"=""}}, {"battery1voltage"=3.4816396, "battery2voltage"=3.4830475, "battery3voltage"=3.4783695, "battery4voltage"=3.4823625, "battery5voltage"=3.4844, "battery6voltage"=0.0, "battery7voltage"=0.0, "battery8voltage"=0.0, "battery9voltage"=0.0, "battery10voltage"=0.0, "battery11voltage"=0.0, "battery12voltage"=0.0, "battery13voltage"=0.0, "battery14voltage"=0.0, "battery15voltage"=0.0, "battery16voltage"=0.0, "battery17voltage"=0.0, "battery18voltage"=0.0, "battery19voltage"=0.0, "battery20voltage"=0.0, "battery21voltage"=0.0, "battery22voltage"=0.0, "battery23voltage"=0.0, "battery24voltage"=0.0, "ErrorOutData"={"ErrorCode"=0, "ErrorMessage"=""}}, {"battery1voltage"=3.4816408, "battery2voltage"=3.4830441, "battery3voltage"=3.4783738, "battery4voltage"=3.4823687, "battery5voltage"=3.4844046, "battery6voltage"=0.0, "battery7voltage"=0.0, "battery8voltage"=0.0, "battery9voltage"=0.0, "battery10voltage"=0.0, "battery11voltage"=0.0, "battery12voltage"=0.0, "battery13voltage"=0.0, "battery14voltage"=0.0, "battery15voltage"=0.0, "battery16voltage"=0.0, "battery17voltage"=0.0, "battery18voltage"=0.0, "battery19voltage"=0.0, "battery20voltage"=0.0, "battery21voltage"=0.0, "battery22voltage"=0.0, "battery23voltage"=0.0, "battery24voltage"=0.0, "ErrorOutData"={"ErrorCode"=0, "ErrorMessage"=""}}, {"battery1voltage"=3.481637, "battery2voltage"=3.4830446, "battery3voltage"=3.4783685, "battery4voltage"=3.482369, "battery5voltage"=3.4844081, "battery6voltage"=0.0, "battery7voltage"=0.0, "battery8voltage"=0.0, "battery9voltage"=0.0, "battery10voltage"=0.0, "battery11voltage"=0.0, "battery12voltage"=0.0, "battery13voltage"=0.0, "battery14voltage"=0.0, "battery15voltage"=0.0, "battery16voltage"=0.0, "battery17voltage"=0.0, "battery18voltage"=0.0, "battery19voltage"=0.0, "battery20voltage"=0.0, "battery21voltage"=0.0, "battery22voltage"=0.0, "battery23voltage"=0.0, "battery24voltage"=0.0, "ErrorOutData"={"ErrorCode"=0, "ErrorMessage"=""}}, {"battery1voltage"=3.4816346, "battery2voltage"=3.4830363, "battery3voltage"=3.47837, "battery4voltage"=3.4823632, "battery5voltage"=3.4844027, "battery6voltage"=0.0, "battery7voltage"=0.0, "battery8voltage"=0.0, "battery9voltage"=0.0, "battery10voltage"=0.0, "battery11voltage"=0.0, "battery12voltage"=0.0, "battery13voltage"=0.0, "battery14voltage"=0.0, "battery15voltage"=0.0, "battery16voltage"=0.0, "battery17voltage"=0.0, "battery18voltage"=0.0, "battery19voltage"=0.0, "battery20voltage"=0.0, "battery21voltage"=0.0, "battery22voltage"=0.0, "battery23voltage"=0.0, "battery24voltage"=0.0, "ErrorOutData"={"ErrorCode"=0, "ErrorMessage"=""}}, {"battery1voltage"=3.4816408, "battery2voltage"=3.483043, "battery3voltage"=3.4783766, "battery4voltage"=3.4823682, "battery5voltage"=3.4843986, "battery6voltage"=0.0, "battery7voltage"=0.0, "battery8voltage"=0.0, "battery9voltage"=0.0, "battery10voltage"=0.0, "battery11voltage"=0.0, "battery12voltage"=0.0, "battery13voltage"=0.0, "battery14voltage"=0.0, "battery15voltage"=0.0, "battery16voltage"=0.0, "battery17voltage"=0.0, "battery18voltage"=0.0, "battery19voltage"=0.0, "battery20voltage"=0.0, "battery21voltage"=0.0, "battery22voltage"=0.0, "battery23voltage"=0.0, "battery24voltage"=0.0, "ErrorOutData"={"ErrorCode"=0, "ErrorMessage"=""}}, {"battery1voltage"=3.4816375, "battery2voltage"=3.483044, "battery3voltage"=3.478373, "battery4voltage"=3.4823718, "battery5voltage"=3.4844017, "battery6voltage"=0.0, "battery7voltage"=0.0, "battery8voltage"=0.0, "battery9voltage"=0.0, "battery10voltage"=0.0, "battery11voltage"=0.0, "battery12voltage"=0.0, "battery13voltage"=0.0, "battery14voltage"=0.0, "battery15voltage"=0.0, "battery16voltage"=0.0, "battery17voltage"=0.0, "battery18voltage"=0.0, "battery19voltage"=0.0, "battery20voltage"=0.0, "battery21voltage"=0.0, "battery22voltage"=0.0, "battery23voltage"=0.0, "battery24voltage"=0.0, "ErrorOutData"={"ErrorCode"=0, "ErrorMessage"=""}}, {"battery1voltage"=3.4816356, "battery2voltage"=3.483043, "battery3voltage"=3.4783678, "battery4voltage"=3.4823654, "battery5voltage"=3.4844036, "battery6voltage"=0.0, "battery7voltage"=0.0, "battery8voltage"=0.0, "battery9voltage"=0.0, "battery10voltage"=0.0, "battery11voltage"=0.0, "battery12voltage"=0.0, "battery13voltage"=0.0, "battery14voltage"=0.0, "battery15voltage"=0.0, "battery16voltage"=0.0, "battery17voltage"=0.0, "battery18voltage"=0.0, "battery19voltage"=0.0, "battery20voltage"=0.0, "battery21voltage"=0.0, "battery22voltage"=0.0, "battery23voltage"=0.0, "battery24voltage"=0.0, "ErrorOutData"={"ErrorCode"=0, "ErrorMessage"=""}}, {"battery1voltage"=3.481638, "battery2voltage"=3.4830418, "battery3voltage"=3.4783711, "battery4voltage"=3.48237, "battery5voltage"=3.4843993, "battery6voltage"=0.0, "battery7voltage"=0.0, "battery8voltage"=0.0, "battery9voltage"=0.0, "battery10voltage"=0.0, "battery11voltage"=0.0, "battery12voltage"=0.0, "battery13voltage"=0.0, "battery14voltage"=0.0, "battery15voltage"=0.0, "battery16voltage"=0.0, "battery17voltage"=0.0, "battery18voltage"=0.0, "battery19voltage"=0.0, "battery20voltage"=0.0, "battery21voltage"=0.0, "battery22voltage"=0.0, "battery23voltage"=0.0, "battery24voltage"=0.0, "ErrorOutData"={"ErrorCode"=0, "ErrorMessage"=""}}, {"battery1voltage"=3.4816396, "battery2voltage"=3.4830391, "battery3voltage"=3.478367, "battery4voltage"=3.482371, "battery5voltage"=3.4844043, "battery6voltage"=0.0, "battery7voltage"=0.0, "battery8voltage"=0.0, "battery9voltage"=0.0, "battery10voltage"=0.0, "battery11voltage"=0.0, "battery12voltage"=0.0, "battery13voltage"=0.0, "battery14voltage"=0.0, "battery15voltage"=0.0, "battery16voltage"=0.0, "battery17voltage"=0.0, "battery18voltage"=0.0, "battery19voltage"=0.0, "battery20voltage"=0.0, "battery21voltage"=0.0, "battery22voltage"=0.0, "battery23voltage"=0.0, "battery24voltage"=0.0, "ErrorOutData"={"ErrorCode"=0, "ErrorMessage"=""}}, {"battery1voltage"=3.4816358, "battery2voltage"=3.4830422, "battery3voltage"=3.478368, "battery4voltage"=3.4823675, "battery5voltage"=3.4844017, "battery6voltage"=0.0, "battery7voltage"=0.0, "battery8voltage"=0.0, "battery9voltage"=0.0, "battery10voltage"=0.0, "battery11voltage"=0.0, "battery12voltage"=0.0, "battery13voltage"=0.0, "battery14voltage"=0.0, "battery15voltage"=0.0, "battery16voltage"=0.0, "battery17voltage"=0.0, "battery18voltage"=0.0, "battery19voltage"=0.0, "battery20voltage"=0.0, "battery21voltage"=0.0, "battery22voltage"=0.0, "battery23voltage"=0.0, "battery24voltage"=0.0, "ErrorOutData"={"ErrorCode"=0, "ErrorMessage"=""}}, {"battery1voltage"=3.4816408, "battery2voltage"=3.4830387, "battery3voltage"=3.4783654, "battery4voltage"=3.4823616, "battery5voltage"=3.4844038, "battery6voltage"=0.0, "battery7voltage"=0.0, "battery8voltage"=0.0, "battery9voltage"=0.0, "battery10voltage"=0.0, "battery11voltage"=0.0, "battery12voltage"=0.0, "battery13voltage"=0.0, "battery14voltage"=0.0, "battery15voltage"=0.0, "battery16voltage"=0.0, "battery17voltage"=0.0, "battery18voltage"=0.0, "battery19voltage"=0.0, "battery20voltage"=0.0, "battery21voltage"=0.0, "battery22voltage"=0.0, "battery23voltage"=0.0, "battery24voltage"=0.0, "ErrorOutData"={"ErrorCode"=0, "ErrorMessage"=""}}, {"battery1voltage"=3.4816396, "battery2voltage"=3.4830444, "battery3voltage"=3.478378, "battery4voltage"=3.4823694, "battery5voltage"=3.4844, "battery6voltage"=0.0, "battery7voltage"=0.0, "battery8voltage"=0.0, "battery9voltage"=0.0, "battery10voltage"=0.0, "battery11voltage"=0.0, "battery12voltage"=0.0, "battery13voltage"=0.0, "battery14voltage"=0.0, "battery15voltage"=0.0, "battery16voltage"=0.0, "battery17voltage"=0.0, "battery18voltage"=0.0, "battery19voltage"=0.0, "battery20voltage"=0.0, "battery21voltage"=0.0, "battery22voltage"=0.0, "battery23voltage"=0.0, "battery24voltage"=0.0, "ErrorOutData"={"ErrorCode"=0, "ErrorMessage"=""}}, {"battery1voltage"=3.4816313, "battery2voltage"=3.4830422, "battery3voltage"=3.4783711, "battery4voltage"=3.482364, "battery5voltage"=3.4844058, "battery6voltage"=0.0, "battery7voltage"=0.0, "battery8voltage"=0.0, "battery9voltage"=0.0, "battery10voltage"=0.0, "battery11voltage"=0.0, "battery12voltage"=0.0, "battery13voltage"=0.0, "battery14voltage"=0.0, "battery15voltage"=0.0, "battery16voltage"=0.0, "battery17voltage"=0.0, "battery18voltage"=0.0, "battery19voltage"=0.0, "battery20voltage"=0.0, "battery21voltage"=0.0, "battery22voltage"=0.0, "battery23voltage"=0.0, "battery24voltage"=0.0, "ErrorOutData"={"ErrorCode"=0, "ErrorMessage"=""}}, {"battery1voltage"=3.481634, "battery2voltage"=3.483035, "battery3voltage"=3.4783714, "battery4voltage"=3.4823709, "battery5voltage"=3.4844048, "battery6voltage"=0.0, "battery7voltage"=0.0, "battery8voltage"=0.0, "battery9voltage"=0.0, "battery10voltage"=0.0, "battery11voltage"=0.0, "battery12voltage"=0.0, "battery13voltage"=0.0, "battery14voltage"=0.0, "battery15voltage"=0.0, "battery16voltage"=0.0, "battery17voltage"=0.0, "battery18voltage"=0.0, "battery19voltage"=0.0, "battery20voltage"=0.0, "battery21voltage"=0.0, "battery22voltage"=0.0, "battery23voltage"=0.0, "battery24voltage"=0.0, "ErrorOutData"={"ErrorCode"=0, "ErrorMessage"=""}}, {"battery1voltage"=3.4816365, "battery2voltage"=3.483043, "battery3voltage"=3.478366, "battery4voltage"=3.4823658, "battery5voltage"=3.484407, "battery6voltage"=0.0, "battery7voltage"=0.0, "battery8voltage"=0.0, "battery9voltage"=0.0, "battery10voltage"=0.0, "battery11voltage"=0.0, "battery12voltage"=0.0, "battery13voltage"=0.0, "battery14voltage"=0.0, "battery15voltage"=0.0, "battery16voltage"=0.0, "battery17voltage"=0.0, "battery18voltage"=0.0, "battery19voltage"=0.0, "battery20voltage"=0.0, "battery21voltage"=0.0, "battery22voltage"=0.0, "battery23voltage"=0.0, "battery24voltage"=0.0, "ErrorOutData"={"ErrorCode"=0, "ErrorMessage"=""}}, {"battery1voltage"=3.481638, "battery2voltage"=3.4830425, "battery3voltage"=3.4783754, "battery4voltage"=3.4823692, "battery5voltage"=3.4844003, "battery6voltage"=0.0, "battery7voltage"=0.0, "battery8voltage"=0.0, "battery9voltage"=0.0, "battery10voltage"=0.0, "battery11voltage"=0.0, "battery12voltage"=0.0, "battery13voltage"=0.0, "battery14voltage"=0.0, "battery15voltage"=0.0, "battery16voltage"=0.0, "battery17voltage"=0.0, "battery18voltage"=0.0, "battery19voltage"=0.0, "battery20voltage"=0.0, "battery21voltage"=0.0, "battery22voltage"=0.0, "battery23voltage"=0.0, "battery24voltage"=0.0, "ErrorOutData"={"ErrorCode"=0, "ErrorMessage"=""}}, {"battery1voltage"=3.4816403, "battery2voltage"=3.483042, "battery3voltage"=3.4783745, "battery4voltage"=3.4823651, "battery5voltage"=3.4844043, "battery6voltage"=0.0, "battery7voltage"=0.0, "battery8voltage"=0.0, "battery9voltage"=0.0, "battery10voltage"=0.0, "battery11voltage"=0.0, "battery12voltage"=0.0, "battery13voltage"=0.0, "battery14voltage"=0.0, "battery15voltage"=0.0, "battery16voltage"=0.0, "battery17voltage"=0.0, "battery18voltage"=0.0, "battery19voltage"=0.0, "battery20voltage"=0.0, "battery21voltage"=0.0, "battery22voltage"=0.0, "battery23voltage"=0.0, "battery24voltage"=0.0, "ErrorOutData"={"ErrorCode"=0, "ErrorMessage"=""}}, {"battery1voltage"=3.4816394, "battery2voltage"=3.483042, "battery3voltage"=3.4783716, "battery4voltage"=3.4823654, "battery5voltage"=3.4844031, "battery6voltage"=0.0, "battery7voltage"=0.0, "battery8voltage"=0.0, "battery9voltage"=0.0, "battery10voltage"=0.0, "battery11voltage"=0.0, "battery12voltage"=0.0, "battery13voltage"=0.0, "battery14voltage"=0.0, "battery15voltage"=0.0, "battery16voltage"=0.0, "battery17voltage"=0.0, "battery18voltage"=0.0, "battery19voltage"=0.0, "battery20voltage"=0.0, "battery21voltage"=0.0, "battery22voltage"=0.0, "battery23voltage"=0.0, "battery24voltage"=0.0, "ErrorOutData"={"ErrorCode"=0, "ErrorMessage"=""}}, {"battery1voltage"=3.4816377, "battery2voltage"=3.4830356, "battery3voltage"=3.4783716, "battery4voltage"=3.4823618, "battery5voltage"=3.484405, "battery6voltage"=0.0, "battery7voltage"=0.0, "battery8voltage"=0.0, "battery9voltage"=0.0, "battery10voltage"=0.0, "battery11voltage"=0.0, "battery12voltage"=0.0, "battery13voltage"=0.0, "battery14voltage"=0.0, "battery15voltage"=0.0, "battery16voltage"=0.0, "battery17voltage"=0.0, "battery18voltage"=0.0, "battery19voltage"=0.0, "battery20voltage"=0.0, "battery21voltage"=0.0, "battery22voltage"=0.0, "battery23voltage"=0.0, "battery24voltage"=0.0, "ErrorOutData"={"ErrorCode"=0, "ErrorMessage"=""}}, {"battery1voltage"=3.4816372, "battery2voltage"=3.4830413, "battery3voltage"=3.4783735, "battery4voltage"=3.4823678, "battery5voltage"=3.4844072, "battery6voltage"=0.0, "battery7voltage"=0.0, "battery8voltage"=0.0, "battery9voltage"=0.0, "battery10voltage"=0.0, "battery11voltage"=0.0, "battery12voltage"=0.0, "battery13voltage"=0.0, "battery14voltage"=0.0, "battery15voltage"=0.0, "battery16voltage"=0.0, "battery17voltage"=0.0, "battery18voltage"=0.0, "battery19voltage"=0.0, "battery20voltage"=0.0, "battery21voltage"=0.0, "battery22voltage"=0.0, "battery23voltage"=0.0, "battery24voltage"=0.0, "ErrorOutData"={"ErrorCode"=0, "ErrorMessage"=""}}, {"battery1voltage"=3.4816365, "battery2voltage"=3.4830425, "battery3voltage"=3.4783704, "battery4voltage"=3.4823644, "battery5voltage"=3.484408, "battery6voltage"=0.0, "battery7voltage"=0.0, "battery8voltage"=0.0, "battery9voltage"=0.0, "battery10voltage"=0.0, "battery11voltage"=0.0, "battery12voltage"=0.0, "battery13voltage"=0.0, "battery14voltage"=0.0, "battery15voltage"=0.0, "battery16voltage"=0.0, "battery17voltage"=0.0, "battery18voltage"=0.0, "battery19voltage"=0.0, "battery20voltage"=0.0, "battery21voltage"=0.0, "battery22voltage"=0.0, "battery23voltage"=0.0, "battery24voltage"=0.0, "ErrorOutData"={"ErrorCode"=0, "ErrorMessage"=""}}, {"battery1voltage"=3.4816365, "battery2voltage"=3.483042, "battery3voltage"=3.4783669, "battery4voltage"=3.4823694, "battery5voltage"=3.4844058, "battery6voltage"=0.0, "battery7voltage"=0.0, "battery8voltage"=0.0, "battery9voltage"=0.0, "battery10voltage"=0.0, "battery11voltage"=0.0, "battery12voltage"=0.0, "battery13voltage"=0.0, "battery14voltage"=0.0, "battery15voltage"=0.0, "battery16voltage"=0.0, "battery17voltage"=0.0, "battery18voltage"=0.0, "battery19voltage"=0.0, "battery20voltage"=0.0, "battery21voltage"=0.0, "battery22voltage"=0.0, "battery23voltage"=0.0, "battery24voltage"=0.0, "ErrorOutData"={"ErrorCode"=0, "ErrorMessage"=""}}, {"battery1voltage"=3.4816382, "battery2voltage"=3.4830441, "battery3voltage"=3.4783742, "battery4voltage"=3.4823668, "battery5voltage"=3.4844027, "battery6voltage"=0.0, "battery7voltage"=0.0, "battery8voltage"=0.0, "battery9voltage"=0.0, "battery10voltage"=0.0, "battery11voltage"=0.0, "battery12voltage"=0.0, "battery13voltage"=0.0, "battery14voltage"=0.0, "battery15voltage"=0.0, "battery16voltage"=0.0, "battery17voltage"=0.0, "battery18voltage"=0.0, "battery19voltage"=0.0, "battery20voltage"=0.0, "battery21voltage"=0.0, "battery22voltage"=0.0, "battery23voltage"=0.0, "battery24voltage"=0.0, "ErrorOutData"={"ErrorCode"=0, "ErrorMessage"=""}}, {"battery1voltage"=3.481635, "battery2voltage"=3.4830391, "battery3voltage"=3.4783745, "battery4voltage"=3.482365, "battery5voltage"=3.4843988, "battery6voltage"=0.0, "battery7voltage"=0.0, "battery8voltage"=0.0, "battery9voltage"=0.0, "battery10voltage"=0.0, "battery11voltage"=0.0, "battery12voltage"=0.0, "battery13voltage"=0.0, "battery14voltage"=0.0, "battery15voltage"=0.0, "battery16voltage"=0.0, "battery17voltage"=0.0, "battery18voltage"=0.0, "battery19voltage"=0.0, "battery20voltage"=0.0, "battery21voltage"=0.0, "battery22voltage"=0.0, "battery23voltage"=0.0, "battery24voltage"=0.0, "ErrorOutData"={"ErrorCode"=0, "ErrorMessage"=""}}, {"battery1voltage"=3.481638, "battery2voltage"=3.483047, "battery3voltage"=3.478372, "battery4voltage"=3.4823606, "battery5voltage"=3.4844024, "battery6voltage"=0.0, "battery7voltage"=0.0, "battery8voltage"=0.0, "battery9voltage"=0.0, "battery10voltage"=0.0, "battery11voltage"=0.0, "battery12voltage"=0.0, "battery13voltage"=0.0, "battery14voltage"=0.0, "battery15voltage"=0.0, "battery16voltage"=0.0, "battery17voltage"=0.0, "battery18voltage"=0.0, "battery19voltage"=0.0, "battery20voltage"=0.0, "battery21voltage"=0.0, "battery22voltage"=0.0, "battery23voltage"=0.0, "battery24voltage"=0.0, "ErrorOutData"={"ErrorCode"=0, "ErrorMessage"=""}}, {"battery1voltage"=3.481636, "battery2voltage"=3.4830415, "battery3voltage"=3.4783747, "battery4voltage"=3.4823675, "battery5voltage"=3.4844072, "battery6voltage"=0.0, "battery7voltage"=0.0, "battery8voltage"=0.0, "battery9voltage"=0.0, "battery10voltage"=0.0, "battery11voltage"=0.0, "battery12voltage"=0.0, "battery13voltage"=0.0, "battery14voltage"=0.0, "battery15voltage"=0.0, "battery16voltage"=0.0, "battery17voltage"=0.0, "battery18voltage"=0.0, "battery19voltage"=0.0, "battery20voltage"=0.0, "battery21voltage"=0.0, "battery22voltage"=0.0, "battery23voltage"=0.0, "battery24voltage"=0.0, "ErrorOutData"={"ErrorCode"=0, "ErrorMessage"=""}}, {"battery1voltage"=3.4816415, "battery2voltage"=3.4830403, "battery3voltage"=3.4783728, "battery4voltage"=3.4823725, "battery5voltage"=3.4844048, "battery6voltage"=0.0, "battery7voltage"=0.0, "battery8voltage"=0.0, "battery9voltage"=0.0, "battery10voltage"=0.0, "battery11voltage"=0.0, "battery12voltage"=0.0, "battery13voltage"=0.0, "battery14voltage"=0.0, "battery15voltage"=0.0, "battery16voltage"=0.0, "battery17voltage"=0.0, "battery18voltage"=0.0, "battery19voltage"=0.0, "battery20voltage"=0.0, "battery21voltage"=0.0, "battery22voltage"=0.0, "battery23voltage"=0.0, "battery24voltage"=0.0, "ErrorOutData"={"ErrorCode"=0, "ErrorMessage"=""}}, {"battery1voltage"=3.481636, "battery2voltage"=3.4830406, "battery3voltage"=3.4783697, "battery4voltage"=3.4823642, "battery5voltage"=3.4844031, "battery6voltage"=0.0, "battery7voltage"=0.0, "battery8voltage"=0.0, "battery9voltage"=0.0, "battery10voltage"=0.0, "battery11voltage"=0.0, "battery12voltage"=0.0, "battery13voltage"=0.0, "battery14voltage"=0.0, "battery15voltage"=0.0, "battery16voltage"=0.0, "battery17voltage"=0.0, "battery18voltage"=0.0, "battery19voltage"=0.0, "battery20voltage"=0.0, "battery21voltage"=0.0, "battery22voltage"=0.0, "battery23voltage"=0.0, "battery24voltage"=0.0, "ErrorOutData"={"ErrorCode"=0, "ErrorMessage"=""}}, {"battery1voltage"=3.4816332, "battery2voltage"=3.4830465, "battery3voltage"=3.4783716, "battery4voltage"=3.4823651, "battery5voltage"=3.4843996, "battery6voltage"=0.0, "battery7voltage"=0.0, "battery8voltage"=0.0, "battery9voltage"=0.0, "battery10voltage"=0.0, "battery11voltage"=0.0, "battery12voltage"=0.0, "battery13voltage"=0.0, "battery14voltage"=0.0, "battery15voltage"=0.0, "battery16voltage"=0.0, "battery17voltage"=0.0, "battery18voltage"=0.0, "battery19voltage"=0.0, "battery20voltage"=0.0, "battery21voltage"=0.0, "battery22voltage"=0.0, "battery23voltage"=0.0, "battery24voltage"=0.0, "ErrorOutData"={"ErrorCode"=0, "ErrorMessage"=""}}, {"battery1voltage"=3.4816341, "battery2voltage"=3.4830444, "battery3voltage"=3.4783695, "battery4voltage"=3.4823678, "battery5voltage"=3.4844015, "battery6voltage"=0.0, "battery7voltage"=0.0, "battery8voltage"=0.0, "battery9voltage"=0.0, "battery10voltage"=0.0, "battery11voltage"=0.0, "battery12voltage"=0.0, "battery13voltage"=0.0, "battery14voltage"=0.0, "battery15voltage"=0.0, "battery16voltage"=0.0, "battery17voltage"=0.0, "battery18voltage"=0.0, "battery19voltage"=0.0, "battery20voltage"=0.0, "battery21voltage"=0.0, "battery22voltage"=0.0, "battery23voltage"=0.0, "battery24voltage"=0.0, "ErrorOutData"={"ErrorCode"=0, "ErrorMessage"=""}}, {"battery1voltage"=3.4816382, "battery2voltage"=3.483038, "battery3voltage"=3.478367, "battery4voltage"=3.4823651, "battery5voltage"=3.4843996, "battery6voltage"=0.0, "battery7voltage"=0.0, "battery8voltage"=0.0, "battery9voltage"=0.0, "battery10voltage"=0.0, "battery11voltage"=0.0, "battery12voltage"=0.0, "battery13voltage"=0.0, "battery14voltage"=0.0, "battery15voltage"=0.0, "battery16voltage"=0.0, "battery17voltage"=0.0, "battery18voltage"=0.0, "battery19voltage"=0.0, "battery20voltage"=0.0, "battery21voltage"=0.0, "battery22voltage"=0.0, "battery23voltage"=0.0, "battery24voltage"=0.0, "ErrorOutData"={"ErrorCode"=0, "ErrorMessage"=""}}, {"battery1voltage"=3.4816413, "battery2voltage"=3.4830396, "battery3voltage"=3.4783747, "battery4voltage"=3.4823666, "battery5voltage"=3.4844053, "battery6voltage"=0.0, "battery7voltage"=0.0, "battery8voltage"=0.0, "battery9voltage"=0.0, "battery10voltage"=0.0, "battery11voltage"=0.0, "battery12voltage"=0.0, "battery13voltage"=0.0, "battery14voltage"=0.0, "battery15voltage"=0.0, "battery16voltage"=0.0, "battery17voltage"=0.0, "battery18voltage"=0.0, "battery19voltage"=0.0, "battery20voltage"=0.0, "battery21voltage"=0.0, "battery22voltage"=0.0, "battery23voltage"=0.0, "battery24voltage"=0.0, "ErrorOutData"={"ErrorCode"=0, "ErrorMessage"=""}}, {"battery1voltage"=3.4816377, "battery2voltage"=3.483037, "battery3voltage"=3.4783723, "battery4voltage"=3.4823637, "battery5voltage"=3.4844053, "battery6voltage"=0.0, "battery7voltage"=0.0, "battery8voltage"=0.0, "battery9voltage"=0.0, "battery10voltage"=0.0, "battery11voltage"=0.0, "battery12voltage"=0.0, "battery13voltage"=0.0, "battery14voltage"=0.0, "battery15voltage"=0.0, "battery16voltage"=0.0, "battery17voltage"=0.0, "battery18voltage"=0.0, "battery19voltage"=0.0, "battery20voltage"=0.0, "battery21voltage"=0.0, "battery22voltage"=0.0, "battery23voltage"=0.0, "battery24voltage"=0.0, "ErrorOutData"={"ErrorCode"=0, "ErrorMessage"=""}}, {"battery1voltage"=3.4816337, "battery2voltage"=3.4830418, "battery3voltage"=3.4783666, "battery4voltage"=3.4823608, "battery5voltage"=3.484405, "battery6voltage"=0.0, "battery7voltage"=0.0, "battery8voltage"=0.0, "battery9voltage"=0.0, "battery10voltage"=0.0, "battery11voltage"=0.0, "battery12voltage"=0.0, "battery13voltage"=0.0, "battery14voltage"=0.0, "battery15voltage"=0.0, "battery16voltage"=0.0, "battery17voltage"=0.0, "battery18voltage"=0.0, "battery19voltage"=0.0, "battery20voltage"=0.0, "battery21voltage"=0.0, "battery22voltage"=0.0, "battery23voltage"=0.0, "battery24voltage"=0.0, "ErrorOutData"={"ErrorCode"=0, "ErrorMessage"=""}}, {"battery1voltage"=3.4816344, "battery2voltage"=3.483046, "battery3voltage"=3.4783738, "battery4voltage"=3.4823682, "battery5voltage"=3.4844005, "battery6voltage"=0.0, "battery7voltage"=0.0, "battery8voltage"=0.0, "battery9voltage"=0.0, "battery10voltage"=0.0, "battery11voltage"=0.0, "battery12voltage"=0.0, "battery13voltage"=0.0, "battery14voltage"=0.0, "battery15voltage"=0.0, "battery16voltage"=0.0, "battery17voltage"=0.0, "battery18voltage"=0.0, "battery19voltage"=0.0, "battery20voltage"=0.0, "battery21voltage"=0.0, "battery22voltage"=0.0, "battery23voltage"=0.0, "battery24voltage"=0.0, "ErrorOutData"={"ErrorCode"=0, "ErrorMessage"=""}}, {"battery1voltage"=3.4816356, "battery2voltage"=3.483044, "battery3voltage"=3.4783733, "battery4voltage"=3.4823635, "battery5voltage"=3.4844043, "battery6voltage"=0.0, "battery7voltage"=0.0, "battery8voltage"=0.0, "battery9voltage"=0.0, "battery10voltage"=0.0, "battery11voltage"=0.0, "battery12voltage"=0.0, "battery13voltage"=0.0, "battery14voltage"=0.0, "battery15voltage"=0.0, "battery16voltage"=0.0, "battery17voltage"=0.0, "battery18voltage"=0.0, "battery19voltage"=0.0, "battery20voltage"=0.0, "battery21voltage"=0.0, "battery22voltage"=0.0, "battery23voltage"=0.0, "battery24voltage"=0.0, "ErrorOutData"={"ErrorCode"=0, "ErrorMessage"=""}}, {"battery1voltage"=3.4816418, "battery2voltage"=3.4830456, "battery3voltage"=3.4783714, "battery4voltage"=3.4823654, "battery5voltage"=3.4844022, "battery6voltage"=0.0, "battery7voltage"=0.0, "battery8voltage"=0.0, "battery9voltage"=0.0, "battery10voltage"=0.0, "battery11voltage"=0.0, "battery12voltage"=0.0, "battery13voltage"=0.0, "battery14voltage"=0.0, "battery15voltage"=0.0, "battery16voltage"=0.0, "battery17voltage"=0.0, "battery18voltage"=0.0, "battery19voltage"=0.0, "battery20voltage"=0.0, "battery21voltage"=0.0, "battery22voltage"=0.0, "battery23voltage"=0.0, "battery24voltage"=0.0, "ErrorOutData"={"ErrorCode"=0, "ErrorMessage"=""}}, {"battery1voltage"=3.4816408, "battery2voltage"=3.4830449, "battery3voltage"=3.4783735, "battery4voltage"=3.4823651, "battery5voltage"=3.4844015, "battery6voltage"=0.0, "battery7voltage"=0.0, "battery8voltage"=0.0, "battery9voltage"=0.0, "battery10voltage"=0.0, "battery11voltage"=0.0, "battery12voltage"=0.0, "battery13voltage"=0.0, "battery14voltage"=0.0, "battery15voltage"=0.0, "battery16voltage"=0.0, "battery17voltage"=0.0, "battery18voltage"=0.0, "battery19voltage"=0.0, "battery20voltage"=0.0, "battery21voltage"=0.0, "battery22voltage"=0.0, "battery23voltage"=0.0, "battery24voltage"=0.0, "ErrorOutData"={"ErrorCode"=0, "ErrorMessage"=""}}, {"battery1voltage"=3.4816337, "battery2voltage"=3.4830387, "battery3voltage"=3.478374, "battery4voltage"=3.4823635, "battery5voltage"=3.484406, "battery6voltage"=0.0, "battery7voltage"=0.0, "battery8voltage"=0.0, "battery9voltage"=0.0, "battery10voltage"=0.0, "battery11voltage"=0.0, "battery12voltage"=0.0, "battery13voltage"=0.0, "battery14voltage"=0.0, "battery15voltage"=0.0, "battery16voltage"=0.0, "battery17voltage"=0.0, "battery18voltage"=0.0, "battery19voltage"=0.0, "battery20voltage"=0.0, "battery21voltage"=0.0, "battery22voltage"=0.0, "battery23voltage"=0.0, "battery24voltage"=0.0, "ErrorOutData"={"ErrorCode"=0, "ErrorMessage"=""}}, {"battery1voltage"=3.4816363, "battery2voltage"=3.483043, "battery3voltage"=3.4783645, "battery4voltage"=3.482366, "battery5voltage"=3.484409, "battery6voltage"=0.0, "battery7voltage"=0.0, "battery8voltage"=0.0, "battery9voltage"=0.0, "battery10voltage"=0.0, "battery11voltage"=0.0, "battery12voltage"=0.0, "battery13voltage"=0.0, "battery14voltage"=0.0, "battery15voltage"=0.0, "battery16voltage"=0.0, "battery17voltage"=0.0, "battery18voltage"=0.0, "battery19voltage"=0.0, "battery20voltage"=0.0, "battery21voltage"=0.0, "battery22voltage"=0.0, "battery23voltage"=0.0, "battery24voltage"=0.0, "ErrorOutData"={"ErrorCode"=0, "ErrorMessage"=""}}, {"battery1voltage"=3.481636, "battery2voltage"=3.4830484, "battery3voltage"=3.4783742, "battery4voltage"=3.482362, "battery5voltage"=3.4843972, "battery6voltage"=0.0, "battery7voltage"=0.0, "battery8voltage"=0.0, "battery9voltage"=0.0, "battery10voltage"=0.0, "battery11voltage"=0.0, "battery12voltage"=0.0, "battery13voltage"=0.0, "battery14voltage"=0.0, "battery15voltage"=0.0, "battery16voltage"=0.0, "battery17voltage"=0.0, "battery18voltage"=0.0, "battery19voltage"=0.0, "battery20voltage"=0.0, "battery21voltage"=0.0, "battery22voltage"=0.0, "battery23voltage"=0.0, "battery24voltage"=0.0, "ErrorOutData"={"ErrorCode"=0, "ErrorMessage"=""}}, {"battery1voltage"=3.481641, "battery2voltage"=3.4830406, "battery3voltage"=3.4783664, "battery4voltage"=3.4823654, "battery5voltage"=3.4843993, "battery6voltage"=0.0, "battery7voltage"=0.0, "battery8voltage"=0.0, "battery9voltage"=0.0, "battery10voltage"=0.0, "battery11voltage"=0.0, "battery12voltage"=0.0, "battery13voltage"=0.0, "battery14voltage"=0.0, "battery15voltage"=0.0, "battery16voltage"=0.0, "battery17voltage"=0.0, "battery18voltage"=0.0, "battery19voltage"=0.0, "battery20voltage"=0.0, "battery21voltage"=0.0, "battery22voltage"=0.0, "battery23voltage"=0.0, "battery24voltage"=0.0, "ErrorOutData"={"ErrorCode"=0, "ErrorMessage"=""}}, {"battery1voltage"=3.4816375, "battery2voltage"=3.4830456, "battery3voltage"=3.4783711, "battery4voltage"=3.4823697, "battery5voltage"=3.4843976, "battery6voltage"=0.0, "battery7voltage"=0.0, "battery8voltage"=0.0, "battery9voltage"=0.0, "battery10voltage"=0.0, "battery11voltage"=0.0, "battery12voltage"=0.0, "battery13voltage"=0.0, "battery14voltage"=0.0, "battery15voltage"=0.0, "battery16voltage"=0.0, "battery17voltage"=0.0, "battery18voltage"=0.0, "battery19voltage"=0.0, "battery20voltage"=0.0, "battery21voltage"=0.0, "battery22voltage"=0.0, "battery23voltage"=0.0, "battery24voltage"=0.0, "ErrorOutData"={"ErrorCode"=0, "ErrorMessage"=""}}, {"battery1voltage"=3.4816408, "battery2voltage"=3.4830403, "battery3voltage"=3.478377, "battery4voltage"=3.4823678, "battery5voltage"=3.484401, "battery6voltage"=0.0, "battery7voltage"=0.0, "battery8voltage"=0.0, "battery9voltage"=0.0, "battery10voltage"=0.0, "battery11voltage"=0.0, "battery12voltage"=0.0, "battery13voltage"=0.0, "battery14voltage"=0.0, "battery15voltage"=0.0, "battery16voltage"=0.0, "battery17voltage"=0.0, "battery18voltage"=0.0, "battery19voltage"=0.0, "battery20voltage"=0.0, "battery21voltage"=0.0, "battery22voltage"=0.0, "battery23voltage"=0.0, "battery24voltage"=0.0, "ErrorOutData"={"ErrorCode"=0, "ErrorMessage"=""}}, {"battery1voltage"=3.4816346, "battery2voltage"=3.483044, "battery3voltage"=3.4783707, "battery4voltage"=3.482368, "battery5voltage"=3.484405, "battery6voltage"=0.0, "battery7voltage"=0.0, "battery8voltage"=0.0, "battery9voltage"=0.0, "battery10voltage"=0.0, "battery11voltage"=0.0, "battery12voltage"=0.0, "battery13voltage"=0.0, "battery14voltage"=0.0, "battery15voltage"=0.0, "battery16voltage"=0.0, "battery17voltage"=0.0, "battery18voltage"=0.0, "battery19voltage"=0.0, "battery20voltage"=0.0, "battery21voltage"=0.0, "battery22voltage"=0.0, "battery23voltage"=0.0, "battery24voltage"=0.0, "ErrorOutData"={"ErrorCode"=0, "ErrorMessage"=""}}, {"battery1voltage"=3.4816341, "battery2voltage"=3.4830408, "battery3voltage"=3.4783692, "battery4voltage"=3.4823656, "battery5voltage"=3.4844005, "battery6voltage"=0.0, "battery7voltage"=0.0, "battery8voltage"=0.0, "battery9voltage"=0.0, "battery10voltage"=0.0, "battery11voltage"=0.0, "battery12voltage"=0.0, "battery13voltage"=0.0, "battery14voltage"=0.0, "battery15voltage"=0.0, "battery16voltage"=0.0, "battery17voltage"=0.0, "battery18voltage"=0.0, "battery19voltage"=0.0, "battery20voltage"=0.0, "battery21voltage"=0.0, "battery22voltage"=0.0, "battery23voltage"=0.0, "battery24voltage"=0.0, "ErrorOutData"={"ErrorCode"=0, "ErrorMessage"=""}}, {"battery1voltage"=3.4816403, "battery2voltage"=3.4830394, "battery3voltage"=3.478372, "battery4voltage"=3.4823704, "battery5voltage"=3.4844024, "battery6voltage"=0.0, "battery7voltage"=0.0, "battery8voltage"=0.0, "battery9voltage"=0.0, "battery10voltage"=0.0, "battery11voltage"=0.0, "battery12voltage"=0.0, "battery13voltage"=0.0, "battery14voltage"=0.0, "battery15voltage"=0.0, "battery16voltage"=0.0, "battery17voltage"=0.0, "battery18voltage"=0.0, "battery19voltage"=0.0, "battery20voltage"=0.0, "battery21voltage"=0.0, "battery22voltage"=0.0, "battery23voltage"=0.0, "battery24voltage"=0.0, "ErrorOutData"={"ErrorCode"=0, "ErrorMessage"=""}}, {"battery1voltage"=3.4816408, "battery2voltage"=3.483041, "battery3voltage"=3.4783754, "battery4voltage"=3.4823687, "battery5voltage"=3.4843972, "battery6voltage"=0.0, "battery7voltage"=0.0, "battery8voltage"=0.0, "battery9voltage"=0.0, "battery10voltage"=0.0, "battery11voltage"=0.0, "battery12voltage"=0.0, "battery13voltage"=0.0, "battery14voltage"=0.0, "battery15voltage"=0.0, "battery16voltage"=0.0, "battery17voltage"=0.0, "battery18voltage"=0.0, "battery19voltage"=0.0, "battery20voltage"=0.0, "battery21voltage"=0.0, "battery22voltage"=0.0, "battery23voltage"=0.0, "battery24voltage"=0.0, "ErrorOutData"={"ErrorCode"=0, "ErrorMessage"=""}}, {"battery1voltage"=3.4816437, "battery2voltage"=3.4830434, "battery3voltage"=3.4783714, "battery4voltage"=3.482368, "battery5voltage"=3.4844015, "battery6voltage"=0.0, "battery7voltage"=0.0, "battery8voltage"=0.0, "battery9voltage"=0.0, "battery10voltage"=0.0, "battery11voltage"=0.0, "battery12voltage"=0.0, "battery13voltage"=0.0, "battery14voltage"=0.0, "battery15voltage"=0.0, "battery16voltage"=0.0, "battery17voltage"=0.0, "battery18voltage"=0.0, "battery19voltage"=0.0, "battery20voltage"=0.0, "battery21voltage"=0.0, "battery22voltage"=0.0, "battery23voltage"=0.0, "battery24voltage"=0.0, "ErrorOutData"={"ErrorCode"=0, "ErrorMessage"=""}}, {"battery1voltage"=3.4816349, "battery2voltage"=3.4830441, "battery3voltage"=3.4783683, "battery4voltage"=3.4823687, "battery5voltage"=3.4844038, "battery6voltage"=0.0, "battery7voltage"=0.0, "battery8voltage"=0.0, "battery9voltage"=0.0, "battery10voltage"=0.0, "battery11voltage"=0.0, "battery12voltage"=0.0, "battery13voltage"=0.0, "battery14voltage"=0.0, "battery15voltage"=0.0, "battery16voltage"=0.0, "battery17voltage"=0.0, "battery18voltage"=0.0, "battery19voltage"=0.0, "battery20voltage"=0.0, "battery21voltage"=0.0, "battery22voltage"=0.0, "battery23voltage"=0.0, "battery24voltage"=0.0, "ErrorOutData"={"ErrorCode"=0, "ErrorMessage"=""}}, {"battery1voltage"=3.481637, "battery2voltage"=3.4830406, "battery3voltage"=3.4783692, "battery4voltage"=3.4823644, "battery5voltage"=3.4843986, "battery6voltage"=0.0, "battery7voltage"=0.0, "battery8voltage"=0.0, "battery9voltage"=0.0, "battery10voltage"=0.0, "battery11voltage"=0.0, "battery12voltage"=0.0, "battery13voltage"=0.0, "battery14voltage"=0.0, "battery15voltage"=0.0, "battery16voltage"=0.0, "battery17voltage"=0.0, "battery18voltage"=0.0, "battery19voltage"=0.0, "battery20voltage"=0.0, "battery21voltage"=0.0, "battery22voltage"=0.0, "battery23voltage"=0.0, "battery24voltage"=0.0, "ErrorOutData"={"ErrorCode"=0, "ErrorMessage"=""}}, {"battery1voltage"=3.4816344, "battery2voltage"=3.4830406, "battery3voltage"=3.4783664, "battery4voltage"=3.4823673, "battery5voltage"=3.4844007, "battery6voltage"=0.0, "battery7voltage"=0.0, "battery8voltage"=0.0, "battery9voltage"=0.0, "battery10voltage"=0.0, "battery11voltage"=0.0, "battery12voltage"=0.0, "battery13voltage"=0.0, "battery14voltage"=0.0, "battery15voltage"=0.0, "battery16voltage"=0.0, "battery17voltage"=0.0, "battery18voltage"=0.0, "battery19voltage"=0.0, "battery20voltage"=0.0, "battery21voltage"=0.0, "battery22voltage"=0.0, "battery23voltage"=0.0, "battery24voltage"=0.0, "ErrorOutData"={"ErrorCode"=0, "ErrorMessage"=""}}, {"battery1voltage"=3.481637, "battery2voltage"=3.4830468, "battery3voltage"=3.4783728, "battery4voltage"=3.4823682, "battery5voltage"=3.4843998, "battery6voltage"=0.0, "battery7voltage"=0.0, "battery8voltage"=0.0, "battery9voltage"=0.0, "battery10voltage"=0.0, "battery11voltage"=0.0, "battery12voltage"=0.0, "battery13voltage"=0.0, "battery14voltage"=0.0, "battery15voltage"=0.0, "battery16voltage"=0.0, "battery17voltage"=0.0, "battery18voltage"=0.0, "battery19voltage"=0.0, "battery20voltage"=0.0, "battery21voltage"=0.0, "battery22voltage"=0.0, "battery23voltage"=0.0, "battery24voltage"=0.0, "ErrorOutData"={"ErrorCode"=0, "ErrorMessage"=""}}, {"battery1voltage"=3.4816344, "battery2voltage"=3.483043, "battery3voltage"=3.4783688, "battery4voltage"=3.48237, "battery5voltage"=3.4844058, "battery6voltage"=0.0, "battery7voltage"=0.0, "battery8voltage"=0.0, "battery9voltage"=0.0, "battery10voltage"=0.0, "battery11voltage"=0.0, "battery12voltage"=0.0, "battery13voltage"=0.0, "battery14voltage"=0.0, "battery15voltage"=0.0, "battery16voltage"=0.0, "battery17voltage"=0.0, "battery18voltage"=0.0, "battery19voltage"=0.0, "battery20voltage"=0.0, "battery21voltage"=0.0, "battery22voltage"=0.0, "battery23voltage"=0.0, "battery24voltage"=0.0, "ErrorOutData"={"ErrorCode"=0, "ErrorMessage"=""}}, {"battery1voltage"=3.4816406, "battery2voltage"=3.4830477, "battery3voltage"=3.4783762, "battery4voltage"=3.4823701, "battery5voltage"=3.4844017, "battery6voltage"=0.0, "battery7voltage"=0.0, "battery8voltage"=0.0, "battery9voltage"=0.0, "battery10voltage"=0.0, "battery11voltage"=0.0, "battery12voltage"=0.0, "battery13voltage"=0.0, "battery14voltage"=0.0, "battery15voltage"=0.0, "battery16voltage"=0.0, "battery17voltage"=0.0, "battery18voltage"=0.0, "battery19voltage"=0.0, "battery20voltage"=0.0, "battery21voltage"=0.0, "battery22voltage"=0.0, "battery23voltage"=0.0, "battery24voltage"=0.0, "ErrorOutData"={"ErrorCode"=0, "ErrorMessage"=""}}, {"battery1voltage"=3.4816418, "battery2voltage"=3.4830415, "battery3voltage"=3.478373, "battery4voltage"=3.4823663, "battery5voltage"=3.4843976, "battery6voltage"=0.0, "battery7voltage"=0.0, "battery8voltage"=0.0, "battery9voltage"=0.0, "battery10voltage"=0.0, "battery11voltage"=0.0, "battery12voltage"=0.0, "battery13voltage"=0.0, "battery14voltage"=0.0, "battery15voltage"=0.0, "battery16voltage"=0.0, "battery17voltage"=0.0, "battery18voltage"=0.0, "battery19voltage"=0.0, "battery20voltage"=0.0, "battery21voltage"=0.0, "battery22voltage"=0.0, "battery23voltage"=0.0, "battery24voltage"=0.0, "ErrorOutData"={"ErrorCode"=0, "ErrorMessage"=""}}, {"battery1voltage"=3.481639, "battery2voltage"=3.483044, "battery3voltage"=3.4783707, "battery4voltage"=3.4823632, "battery5voltage"=3.4843986, "battery6voltage"=0.0, "battery7voltage"=0.0, "battery8voltage"=0.0, "battery9voltage"=0.0, "battery10voltage"=0.0, "battery11voltage"=0.0, "battery12voltage"=0.0, "battery13voltage"=0.0, "battery14voltage"=0.0, "battery15voltage"=0.0, "battery16voltage"=0.0, "battery17voltage"=0.0, "battery18voltage"=0.0, "battery19voltage"=0.0, "battery20voltage"=0.0, "battery21voltage"=0.0, "battery22voltage"=0.0, "battery23voltage"=0.0, "battery24voltage"=0.0, "ErrorOutData"={"ErrorCode"=0, "ErrorMessage"=""}}, {"battery1voltage"=3.481636, "battery2voltage"=3.4830396, "battery3voltage"=3.4783642, "battery4voltage"=3.482362, "battery5voltage"=3.4844024, "battery6voltage"=0.0, "battery7voltage"=0.0, "battery8voltage"=0.0, "battery9voltage"=0.0, "battery10voltage"=0.0, "battery11voltage"=0.0, "battery12voltage"=0.0, "battery13voltage"=0.0, "battery14voltage"=0.0, "battery15voltage"=0.0, "battery16voltage"=0.0, "battery17voltage"=0.0, "battery18voltage"=0.0, "battery19voltage"=0.0, "battery20voltage"=0.0, "battery21voltage"=0.0, "battery22voltage"=0.0, "battery23voltage"=0.0, "battery24voltage"=0.0, "ErrorOutData"={"ErrorCode"=0, "ErrorMessage"=""}}, {"battery1voltage"=3.4816332, "battery2voltage"=3.483045, "battery3voltage"=3.4783719, "battery4voltage"=3.4823678, "battery5voltage"=3.4844031, "battery6voltage"=0.0, "battery7voltage"=0.0, "battery8voltage"=0.0, "battery9voltage"=0.0, "battery10voltage"=0.0, "battery11voltage"=0.0, "battery12voltage"=0.0, "battery13voltage"=0.0, "battery14voltage"=0.0, "battery15voltage"=0.0, "battery16voltage"=0.0, "battery17voltage"=0.0, "battery18voltage"=0.0, "battery19voltage"=0.0, "battery20voltage"=0.0, "battery21voltage"=0.0, "battery22voltage"=0.0, "battery23voltage"=0.0, "battery24voltage"=0.0, "ErrorOutData"={"ErrorCode"=0, "ErrorMessage"=""}}, {"battery1voltage"=3.481638, "battery2voltage"=3.4830458, "battery3voltage"=3.4783735, "battery4voltage"=3.4823663, "battery5voltage"=3.4843988, "battery6voltage"=0.0, "battery7voltage"=0.0, "battery8voltage"=0.0, "battery9voltage"=0.0, "battery10voltage"=0.0, "battery11voltage"=0.0, "battery12voltage"=0.0, "battery13voltage"=0.0, "battery14voltage"=0.0, "battery15voltage"=0.0, "battery16voltage"=0.0, "battery17voltage"=0.0, "battery18voltage"=0.0, "battery19voltage"=0.0, "battery20voltage"=0.0, "battery21voltage"=0.0, "battery22voltage"=0.0, "battery23voltage"=0.0, "battery24voltage"=0.0, "ErrorOutData"={"ErrorCode"=0, "ErrorMessage"=""}}, {"battery1voltage"=3.4816372, "battery2voltage"=3.4830472, "battery3voltage"=3.4783738, "battery4voltage"=3.482365, "battery5voltage"=3.4843976, "battery6voltage"=0.0, "battery7voltage"=0.0, "battery8voltage"=0.0, "battery9voltage"=0.0, "battery10voltage"=0.0, "battery11voltage"=0.0, "battery12voltage"=0.0, "battery13voltage"=0.0, "battery14voltage"=0.0, "battery15voltage"=0.0, "battery16voltage"=0.0, "battery17voltage"=0.0, "battery18voltage"=0.0, "battery19voltage"=0.0, "battery20voltage"=0.0, "battery21voltage"=0.0, "battery22voltage"=0.0, "battery23voltage"=0.0, "battery24voltage"=0.0, "ErrorOutData"={"ErrorCode"=0, "ErrorMessage"=""}}, {"battery1voltage"=3.481633, "battery2voltage"=3.4830394, "battery3voltage"=3.4783714, "battery4voltage"=3.4823642, "battery5voltage"=3.4843976, "battery6voltage"=0.0, "battery7voltage"=0.0, "battery8voltage"=0.0, "battery9voltage"=0.0, "battery10voltage"=0.0, "battery11voltage"=0.0, "battery12voltage"=0.0, "battery13voltage"=0.0, "battery14voltage"=0.0, "battery15voltage"=0.0, "battery16voltage"=0.0, "battery17voltage"=0.0, "battery18voltage"=0.0, "battery19voltage"=0.0, "battery20voltage"=0.0, "battery21voltage"=0.0, "battery22voltage"=0.0, "battery23voltage"=0.0, "battery24voltage"=0.0, "ErrorOutData"={"ErrorCode"=0, "ErrorMessage"=""}}, {"battery1voltage"=3.4816353, "battery2voltage"=3.4830425, "battery3voltage"=3.4783754, "battery4voltage"=3.4823697, "battery5voltage"=3.4844024, "battery6voltage"=0.0, "battery7voltage"=0.0, "battery8voltage"=0.0, "battery9voltage"=0.0, "battery10voltage"=0.0, "battery11voltage"=0.0, "battery12voltage"=0.0, "battery13voltage"=0.0, "battery14voltage"=0.0, "battery15voltage"=0.0, "battery16voltage"=0.0, "battery17voltage"=0.0, "battery18voltage"=0.0, "battery19voltage"=0.0, "battery20voltage"=0.0, "battery21voltage"=0.0, "battery22voltage"=0.0, "battery23voltage"=0.0, "battery24voltage"=0.0, "ErrorOutData"={"ErrorCode"=0, "ErrorMessage"=""}}, {"battery1voltage"=3.4816415, "battery2voltage"=3.4830449, "battery3voltage"=3.4783792, "battery4voltage"=3.4823642, "battery5voltage"=3.4843974, "battery6voltage"=0.0, "battery7voltage"=0.0, "battery8voltage"=0.0, "battery9voltage"=0.0, "battery10voltage"=0.0, "battery11voltage"=0.0, "battery12voltage"=0.0, "battery13voltage"=0.0, "battery14voltage"=0.0, "battery15voltage"=0.0, "battery16voltage"=0.0, "battery17voltage"=0.0, "battery18voltage"=0.0, "battery19voltage"=0.0, "battery20voltage"=0.0, "battery21voltage"=0.0, "battery22voltage"=0.0, "battery23voltage"=0.0, "battery24voltage"=0.0, "ErrorOutData"={"ErrorCode"=0, "ErrorMessage"=""}}, {"battery1voltage"=3.4816365, "battery2voltage"=3.4830422, "battery3voltage"=3.4783711, "battery4voltage"=3.4823658, "battery5voltage"=3.4844017, "battery6voltage"=0.0, "battery7voltage"=0.0, "battery8voltage"=0.0, "battery9voltage"=0.0, "battery10voltage"=0.0, "battery11voltage"=0.0, "battery12voltage"=0.0, "battery13voltage"=0.0, "battery14voltage"=0.0, "battery15voltage"=0.0, "battery16voltage"=0.0, "battery17voltage"=0.0, "battery18voltage"=0.0, "battery19voltage"=0.0, "battery20voltage"=0.0, "battery21voltage"=0.0, "battery22voltage"=0.0, "battery23voltage"=0.0, "battery24voltage"=0.0, "ErrorOutData"={"ErrorCode"=0, "ErrorMessage"=""}}, {"battery1voltage"=3.481645, "battery2voltage"=3.4830458, "battery3voltage"=3.4783716, "battery4voltage"=3.4823675, "battery5voltage"=3.4844, "battery6voltage"=0.0, "battery7voltage"=0.0, "battery8voltage"=0.0, "battery9voltage"=0.0, "battery10voltage"=0.0, "battery11voltage"=0.0, "battery12voltage"=0.0, "battery13voltage"=0.0, "battery14voltage"=0.0, "battery15voltage"=0.0, "battery16voltage"=0.0, "battery17voltage"=0.0, "battery18voltage"=0.0, "battery19voltage"=0.0, "battery20voltage"=0.0, "battery21voltage"=0.0, "battery22voltage"=0.0, "battery23voltage"=0.0, "battery24voltage"=0.0, "ErrorOutData"={"ErrorCode"=0, "ErrorMessage"=""}}, {"battery1voltage"=3.4816349, "battery2voltage"=3.4830406, "battery3voltage"=3.47837, "battery4voltage"=3.482364, "battery5voltage"=3.4844055, "battery6voltage"=0.0, "battery7voltage"=0.0, "battery8voltage"=0.0, "battery9voltage"=0.0, "battery10voltage"=0.0, "battery11voltage"=0.0, "battery12voltage"=0.0, "battery13voltage"=0.0, "battery14voltage"=0.0, "battery15voltage"=0.0, "battery16voltage"=0.0, "battery17voltage"=0.0, "battery18voltage"=0.0, "battery19voltage"=0.0, "battery20voltage"=0.0, "battery21voltage"=0.0, "battery22voltage"=0.0, "battery23voltage"=0.0, "battery24voltage"=0.0, "ErrorOutData"={"ErrorCode"=0, "ErrorMessage"=""}}, {"battery1voltage"=3.481638, "battery2voltage"=3.483042, "battery3voltage"=3.4783695, "battery4voltage"=3.4823694, "battery5voltage"=3.4844022, "battery6voltage"=0.0, "battery7voltage"=0.0, "battery8voltage"=0.0, "battery9voltage"=0.0, "battery10voltage"=0.0, "battery11voltage"=0.0, "battery12voltage"=0.0, "battery13voltage"=0.0, "battery14voltage"=0.0, "battery15voltage"=0.0, "battery16voltage"=0.0, "battery17voltage"=0.0, "battery18voltage"=0.0, "battery19voltage"=0.0, "battery20voltage"=0.0, "battery21voltage"=0.0, "battery22voltage"=0.0, "battery23voltage"=0.0, "battery24voltage"=0.0, "ErrorOutData"={"ErrorCode"=0, "ErrorMessage"=""}}, {"battery1voltage"=3.4816444, "battery2voltage"=3.4830453, "battery3voltage"=3.478374, "battery4voltage"=3.4823692, "battery5voltage"=3.4843988, "battery6voltage"=0.0, "battery7voltage"=0.0, "battery8voltage"=0.0, "battery9voltage"=0.0, "battery10voltage"=0.0, "battery11voltage"=0.0, "battery12voltage"=0.0, "battery13voltage"=0.0, "battery14voltage"=0.0, "battery15voltage"=0.0, "battery16voltage"=0.0, "battery17voltage"=0.0, "battery18voltage"=0.0, "battery19voltage"=0.0, "battery20voltage"=0.0, "battery21voltage"=0.0, "battery22voltage"=0.0, "battery23voltage"=0.0, "battery24voltage"=0.0, "ErrorOutData"={"ErrorCode"=0, "ErrorMessage"=""}}, {"battery1voltage"=3.481642, "battery2voltage"=3.483049, "battery3voltage"=3.4783735, "battery4voltage"=3.482372, "battery5voltage"=3.4843962, "battery6voltage"=0.0, "battery7voltage"=0.0, "battery8voltage"=0.0, "battery9voltage"=0.0, "battery10voltage"=0.0, "battery11voltage"=0.0, "battery12voltage"=0.0, "battery13voltage"=0.0, "battery14voltage"=0.0, "battery15voltage"=0.0, "battery16voltage"=0.0, "battery17voltage"=0.0, "battery18voltage"=0.0, "battery19voltage"=0.0, "battery20voltage"=0.0, "battery21voltage"=0.0, "battery22voltage"=0.0, "battery23voltage"=0.0, "battery24voltage"=0.0, "ErrorOutData"={"ErrorCode"=0, "ErrorMessage"=""}}, {"battery1voltage"=3.4816356, "battery2voltage"=3.4830408, "battery3voltage"=3.4783733, "battery4voltage"=3.482364, "battery5voltage"=3.4844062, "battery6voltage"=0.0, "battery7voltage"=0.0, "battery8voltage"=0.0, "battery9voltage"=0.0, "battery10voltage"=0.0, "battery11voltage"=0.0, "battery12voltage"=0.0, "battery13voltage"=0.0, "battery14voltage"=0.0, "battery15voltage"=0.0, "battery16voltage"=0.0, "battery17voltage"=0.0, "battery18voltage"=0.0, "battery19voltage"=0.0, "battery20voltage"=0.0, "battery21voltage"=0.0, "battery22voltage"=0.0, "battery23voltage"=0.0, "battery24voltage"=0.0, "ErrorOutData"={"ErrorCode"=0, "ErrorMessage"=""}}, {"battery1voltage"=3.481642, "battery2voltage"=3.483041, "battery3voltage"=3.4783692, "battery4voltage"=3.4823654, "battery5voltage"=3.4843974, "battery6voltage"=0.0, "battery7voltage"=0.0, "battery8voltage"=0.0, "battery9voltage"=0.0, "battery10voltage"=0.0, "battery11voltage"=0.0, "battery12voltage"=0.0, "battery13voltage"=0.0, "battery14voltage"=0.0, "battery15voltage"=0.0, "battery16voltage"=0.0, "battery17voltage"=0.0, "battery18voltage"=0.0, "battery19voltage"=0.0, "battery20voltage"=0.0, "battery21voltage"=0.0, "battery22voltage"=0.0, "battery23voltage"=0.0, "battery24voltage"=0.0, "ErrorOutData"={"ErrorCode"=0, "ErrorMessage"=""}}, {"battery1voltage"=3.4816377, "battery2voltage"=3.4830406, "battery3voltage"=3.4783766, "battery4voltage"=3.4823654, "battery5voltage"=3.484399, "battery6voltage"=0.0, "battery7voltage"=0.0, "battery8voltage"=0.0, "battery9voltage"=0.0, "battery10voltage"=0.0, "battery11voltage"=0.0, "battery12voltage"=0.0, "battery13voltage"=0.0, "battery14voltage"=0.0, "battery15voltage"=0.0, "battery16voltage"=0.0, "battery17voltage"=0.0, "battery18voltage"=0.0, "battery19voltage"=0.0, "battery20voltage"=0.0, "battery21voltage"=0.0, "battery22voltage"=0.0, "battery23voltage"=0.0, "battery24voltage"=0.0, "ErrorOutData"={"ErrorCode"=0, "ErrorMessage"=""}}, {"battery1voltage"=3.4816396, "battery2voltage"=3.4830458, "battery3voltage"=3.4783735, "battery4voltage"=3.4823637, "battery5voltage"=3.4843974, "battery6voltage"=0.0, "battery7voltage"=0.0, "battery8voltage"=0.0, "battery9voltage"=0.0, "battery10voltage"=0.0, "battery11voltage"=0.0, "battery12voltage"=0.0, "battery13voltage"=0.0, "battery14voltage"=0.0, "battery15voltage"=0.0, "battery16voltage"=0.0, "battery17voltage"=0.0, "battery18voltage"=0.0, "battery19voltage"=0.0, "battery20voltage"=0.0, "battery21voltage"=0.0, "battery22voltage"=0.0, "battery23voltage"=0.0, "battery24voltage"=0.0, "ErrorOutData"={"ErrorCode"=0, "ErrorMessage"=""}}, {"battery1voltage"=3.4816408, "battery2voltage"=3.4830508, "battery3voltage"=3.4783719, "battery4voltage"=3.482367, "battery5voltage"=3.484396, "battery6voltage"=0.0, "battery7voltage"=0.0, "battery8voltage"=0.0, "battery9voltage"=0.0, "battery10voltage"=0.0, "battery11voltage"=0.0, "battery12voltage"=0.0, "battery13voltage"=0.0, "battery14voltage"=0.0, "battery15voltage"=0.0, "battery16voltage"=0.0, "battery17voltage"=0.0, "battery18voltage"=0.0, "battery19voltage"=0.0, "battery20voltage"=0.0, "battery21voltage"=0.0, "battery22voltage"=0.0, "battery23voltage"=0.0, "battery24voltage"=0.0, "ErrorOutData"={"ErrorCode"=0, "ErrorMessage"=""}}, {"battery1voltage"=3.4816327, "battery2voltage"=3.4830399, "battery3voltage"=3.4783666, "battery4voltage"=3.4823623, "battery5voltage"=3.4844003, "battery6voltage"=0.0, "battery7voltage"=0.0, "battery8voltage"=0.0, "battery9voltage"=0.0, "battery10voltage"=0.0, "battery11voltage"=0.0, "battery12voltage"=0.0, "battery13voltage"=0.0, "battery14voltage"=0.0, "battery15voltage"=0.0, "battery16voltage"=0.0, "battery17voltage"=0.0, "battery18voltage"=0.0, "battery19voltage"=0.0, "battery20voltage"=0.0, "battery21voltage"=0.0, "battery22voltage"=0.0, "battery23voltage"=0.0, "battery24voltage"=0.0, "ErrorOutData"={"ErrorCode"=0, "ErrorMessage"=""}}, {"battery1voltage"=3.4816408, "battery2voltage"=3.483039, "battery3voltage"=3.4783654, "battery4voltage"=3.482365, "battery5voltage"=3.4844074, "battery6voltage"=0.0, "battery7voltage"=0.0, "battery8voltage"=0.0, "battery9voltage"=0.0, "battery10voltage"=0.0, "battery11voltage"=0.0, "battery12voltage"=0.0, "battery13voltage"=0.0, "battery14voltage"=0.0, "battery15voltage"=0.0, "battery16voltage"=0.0, "battery17voltage"=0.0, "battery18voltage"=0.0, "battery19voltage"=0.0, "battery20voltage"=0.0, "battery21voltage"=0.0, "battery22voltage"=0.0, "battery23voltage"=0.0, "battery24voltage"=0.0, "ErrorOutData"={"ErrorCode"=0, "ErrorMessage"=""}}, {"battery1voltage"=3.4816368, "battery2voltage"=3.483042, "battery3voltage"=3.478371, "battery4voltage"=3.4823625, "battery5voltage"=3.4844034, "battery6voltage"=0.0, "battery7voltage"=0.0, "battery8voltage"=0.0, "battery9voltage"=0.0, "battery10voltage"=0.0, "battery11voltage"=0.0, "battery12voltage"=0.0, "battery13voltage"=0.0, "battery14voltage"=0.0, "battery15voltage"=0.0, "battery16voltage"=0.0, "battery17voltage"=0.0, "battery18voltage"=0.0, "battery19voltage"=0.0, "battery20voltage"=0.0, "battery21voltage"=0.0, "battery22voltage"=0.0, "battery23voltage"=0.0, "battery24voltage"=0.0, "ErrorOutData"={"ErrorCode"=0, "ErrorMessage"=""}}, {"battery1voltage"=3.481637, "battery2voltage"=3.4830418, "battery3voltage"=3.4783726, "battery4voltage"=3.4823656, "battery5voltage"=3.484401, "battery6voltage"=0.0, "battery7voltage"=0.0, "battery8voltage"=0.0, "battery9voltage"=0.0, "battery10voltage"=0.0, "battery11voltage"=0.0, "battery12voltage"=0.0, "battery13voltage"=0.0, "battery14voltage"=0.0, "battery15voltage"=0.0, "battery16voltage"=0.0, "battery17voltage"=0.0, "battery18voltage"=0.0, "battery19voltage"=0.0, "battery20voltage"=0.0, "battery21voltage"=0.0, "battery22voltage"=0.0, "battery23voltage"=0.0, "battery24voltage"=0.0, "ErrorOutData"={"ErrorCode"=0, "ErrorMessage"=""}}, {"battery1voltage"=3.4816332, "battery2voltage"=3.4830406, "battery3voltage"=3.4783666, "battery4voltage"=3.482365, "battery5voltage"=3.4844058, "battery6voltage"=0.0, "battery7voltage"=0.0, "battery8voltage"=0.0, "battery9voltage"=0.0, "battery10voltage"=0.0, "battery11voltage"=0.0, "battery12voltage"=0.0, "battery13voltage"=0.0, "battery14voltage"=0.0, "battery15voltage"=0.0, "battery16voltage"=0.0, "battery17voltage"=0.0, "battery18voltage"=0.0, "battery19voltage"=0.0, "battery20voltage"=0.0, "battery21voltage"=0.0, "battery22voltage"=0.0, "battery23voltage"=0.0, "battery24voltage"=0.0, "ErrorOutData"={"ErrorCode"=0, "ErrorMessage"=""}}, {"battery1voltage"=3.481636, "battery2voltage"=3.483039, "battery3voltage"=3.4783719, "battery4voltage"=3.4823658, "battery5voltage"=3.4844055, "battery6voltage"=0.0, "battery7voltage"=0.0, "battery8voltage"=0.0, "battery9voltage"=0.0, "battery10voltage"=0.0, "battery11voltage"=0.0, "battery12voltage"=0.0, "battery13voltage"=0.0, "battery14voltage"=0.0, "battery15voltage"=0.0, "battery16voltage"=0.0, "battery17voltage"=0.0, "battery18voltage"=0.0, "battery19voltage"=0.0, "battery20voltage"=0.0, "battery21voltage"=0.0, "battery22voltage"=0.0, "battery23voltage"=0.0, "battery24voltage"=0.0, "ErrorOutData"={"ErrorCode"=0, "ErrorMessage"=""}}, {"battery1voltage"=3.481638, "battery2voltage"=3.4830458, "battery3voltage"=3.4783742, "battery4voltage"=3.4823635, "battery5voltage"=3.4843984, "battery6voltage"=0.0, "battery7voltage"=0.0, "battery8voltage"=0.0, "battery9voltage"=0.0, "battery10voltage"=0.0, "battery11voltage"=0.0, "battery12voltage"=0.0, "battery13voltage"=0.0, "battery14voltage"=0.0, "battery15voltage"=0.0, "battery16voltage"=0.0, "battery17voltage"=0.0, "battery18voltage"=0.0, "battery19voltage"=0.0, "battery20voltage"=0.0, "battery21voltage"=0.0, "battery22voltage"=0.0, "battery23voltage"=0.0, "battery24voltage"=0.0, "ErrorOutData"={"ErrorCode"=0, "ErrorMessage"=""}}, {"battery1voltage"=3.4816399, "battery2voltage"=3.4830425, "battery3voltage"=3.478365, "battery4voltage"=3.4823668, "battery5voltage"=3.4843957, "battery6voltage"=0.0, "battery7voltage"=0.0, "battery8voltage"=0.0, "battery9voltage"=0.0, "battery10voltage"=0.0, "battery11voltage"=0.0, "battery12voltage"=0.0, "battery13voltage"=0.0, "battery14voltage"=0.0, "battery15voltage"=0.0, "battery16voltage"=0.0, "battery17voltage"=0.0, "battery18voltage"=0.0, "battery19voltage"=0.0, "battery20voltage"=0.0, "battery21voltage"=0.0, "battery22voltage"=0.0, "battery23voltage"=0.0, "battery24voltage"=0.0, "ErrorOutData"={"ErrorCode"=0, "ErrorMessage"=""}}, {"battery1voltage"=3.4816365, "battery2voltage"=3.4830365, "battery3voltage"=3.478368, "battery4voltage"=3.4823666, "battery5voltage"=3.484402, "battery6voltage"=0.0, "battery7voltage"=0.0, "battery8voltage"=0.0, "battery9voltage"=0.0, "battery10voltage"=0.0, "battery11voltage"=0.0, "battery12voltage"=0.0, "battery13voltage"=0.0, "battery14voltage"=0.0, "battery15voltage"=0.0, "battery16voltage"=0.0, "battery17voltage"=0.0, "battery18voltage"=0.0, "battery19voltage"=0.0, "battery20voltage"=0.0, "battery21voltage"=0.0, "battery22voltage"=0.0, "battery23voltage"=0.0, "battery24voltage"=0.0, "ErrorOutData"={"ErrorCode"=0, "ErrorMessage"=""}}, {"battery1voltage"=3.4816375, "battery2voltage"=3.483047, "battery3voltage"=3.4783728, "battery4voltage"=3.482368, "battery5voltage"=3.4843996, "battery6voltage"=0.0, "battery7voltage"=0.0, "battery8voltage"=0.0, "battery9voltage"=0.0, "battery10voltage"=0.0, "battery11voltage"=0.0, "battery12voltage"=0.0, "battery13voltage"=0.0, "battery14voltage"=0.0, "battery15voltage"=0.0, "battery16voltage"=0.0, "battery17voltage"=0.0, "battery18voltage"=0.0, "battery19voltage"=0.0, "battery20voltage"=0.0, "battery21voltage"=0.0, "battery22voltage"=0.0, "battery23voltage"=0.0, "battery24voltage"=0.0, "ErrorOutData"={"ErrorCode"=0, "ErrorMessage"=""}}, {"battery1voltage"=3.4816287, "battery2voltage"=3.4830418, "battery3voltage"=3.4783697, "battery4voltage"=3.4823678, "battery5voltage"=3.484405, "battery6voltage"=0.0, "battery7voltage"=0.0, "battery8voltage"=0.0, "battery9voltage"=0.0, "battery10voltage"=0.0, "battery11voltage"=0.0, "battery12voltage"=0.0, "battery13voltage"=0.0, "battery14voltage"=0.0, "battery15voltage"=0.0, "battery16voltage"=0.0, "battery17voltage"=0.0, "battery18voltage"=0.0, "battery19voltage"=0.0, "battery20voltage"=0.0, "battery21voltage"=0.0, "battery22voltage"=0.0, "battery23voltage"=0.0, "battery24voltage"=0.0, "ErrorOutData"={"ErrorCode"=0, "ErrorMessage"=""}}, {"battery1voltage"=3.481641, "battery2voltage"=3.4830432, "battery3voltage"=3.4783702, "battery4voltage"=3.482362, "battery5voltage"=3.484401, "battery6voltage"=0.0, "battery7voltage"=0.0, "battery8voltage"=0.0, "battery9voltage"=0.0, "battery10voltage"=0.0, "battery11voltage"=0.0, "battery12voltage"=0.0, "battery13voltage"=0.0, "battery14voltage"=0.0, "battery15voltage"=0.0, "battery16voltage"=0.0, "battery17voltage"=0.0, "battery18voltage"=0.0, "battery19voltage"=0.0, "battery20voltage"=0.0, "battery21voltage"=0.0, "battery22voltage"=0.0, "battery23voltage"=0.0, "battery24voltage"=0.0, "ErrorOutData"={"ErrorCode"=0, "ErrorMessage"=""}}, {"battery1voltage"=3.4816341, "battery2voltage"=3.4830415, "battery3voltage"=3.478375, "battery4voltage"=3.4823651, "battery5voltage"=3.4844015, "battery6voltage"=0.0, "battery7voltage"=0.0, "battery8voltage"=0.0, "battery9voltage"=0.0, "battery10voltage"=0.0, "battery11voltage"=0.0, "battery12voltage"=0.0, "battery13voltage"=0.0, "battery14voltage"=0.0, "battery15voltage"=0.0, "battery16voltage"=0.0, "battery17voltage"=0.0, "battery18voltage"=0.0, "battery19voltage"=0.0, "battery20voltage"=0.0, "battery21voltage"=0.0, "battery22voltage"=0.0, "battery23voltage"=0.0, "battery24voltage"=0.0, "ErrorOutData"={"ErrorCode"=0, "ErrorMessage"=""}}, {"battery1voltage"=3.4816413, "battery2voltage"=3.483046, "battery3voltage"=3.4783719, "battery4voltage"=3.4823654, "battery5voltage"=3.4843998, "battery6voltage"=0.0, "battery7voltage"=0.0, "battery8voltage"=0.0, "battery9voltage"=0.0, "battery10voltage"=0.0, "battery11voltage"=0.0, "battery12voltage"=0.0, "battery13voltage"=0.0, "battery14voltage"=0.0, "battery15voltage"=0.0, "battery16voltage"=0.0, "battery17voltage"=0.0, "battery18voltage"=0.0, "battery19voltage"=0.0, "battery20voltage"=0.0, "battery21voltage"=0.0, "battery22voltage"=0.0, "battery23voltage"=0.0, "battery24voltage"=0.0, "ErrorOutData"={"ErrorCode"=0, "ErrorMessage"=""}}, {"battery1voltage"=3.4816396, "battery2voltage"=3.4830406, "battery3voltage"=3.478369, "battery4voltage"=3.4823692, "battery5voltage"=3.484404, "battery6voltage"=0.0, "battery7voltage"=0.0, "battery8voltage"=0.0, "battery9voltage"=0.0, "battery10voltage"=0.0, "battery11voltage"=0.0, "battery12voltage"=0.0, "battery13voltage"=0.0, "battery14voltage"=0.0, "battery15voltage"=0.0, "battery16voltage"=0.0, "battery17voltage"=0.0, "battery18voltage"=0.0, "battery19voltage"=0.0, "battery20voltage"=0.0, "battery21voltage"=0.0, "battery22voltage"=0.0, "battery23voltage"=0.0, "battery24voltage"=0.0, "ErrorOutData"={"ErrorCode"=0, "ErrorMessage"=""}}, {"battery1voltage"=3.4816425, "battery2voltage"=3.4830418, "battery3voltage"=3.4783697, "battery4voltage"=3.4823673, "battery5voltage"=3.4844031, "battery6voltage"=0.0, "battery7voltage"=0.0, "battery8voltage"=0.0, "battery9voltage"=0.0, "battery10voltage"=0.0, "battery11voltage"=0.0, "battery12voltage"=0.0, "battery13voltage"=0.0, "battery14voltage"=0.0, "battery15voltage"=0.0, "battery16voltage"=0.0, "battery17voltage"=0.0, "battery18voltage"=0.0, "battery19voltage"=0.0, "battery20voltage"=0.0, "battery21voltage"=0.0, "battery22voltage"=0.0, "battery23voltage"=0.0, "battery24voltage"=0.0, "ErrorOutData"={"ErrorCode"=0, "ErrorMessage"=""}}, {"battery1voltage"=3.4816406, "battery2voltage"=3.4830463, "battery3voltage"=3.4783733, "battery4voltage"=3.4823668, "battery5voltage"=3.4844012, "battery6voltage"=0.0, "battery7voltage"=0.0, "battery8voltage"=0.0, "battery9voltage"=0.0, "battery10voltage"=0.0, "battery11voltage"=0.0, "battery12voltage"=0.0, "battery13voltage"=0.0, "battery14voltage"=0.0, "battery15voltage"=0.0, "battery16voltage"=0.0, "battery17voltage"=0.0, "battery18voltage"=0.0, "battery19voltage"=0.0, "battery20voltage"=0.0, "battery21voltage"=0.0, "battery22voltage"=0.0, "battery23voltage"=0.0, "battery24voltage"=0.0, "ErrorOutData"={"ErrorCode"=0, "ErrorMessage"=""}}, {"battery1voltage"=3.481635, "battery2voltage"=3.4830434, "battery3voltage"=3.478371, "battery4voltage"=3.4823666, "battery5voltage"=3.484403, "battery6voltage"=0.0, "battery7voltage"=0.0, "battery8voltage"=0.0, "battery9voltage"=0.0, "battery10voltage"=0.0, "battery11voltage"=0.0, "battery12voltage"=0.0, "battery13voltage"=0.0, "battery14voltage"=0.0, "battery15voltage"=0.0, "battery16voltage"=0.0, "battery17voltage"=0.0, "battery18voltage"=0.0, "battery19voltage"=0.0, "battery20voltage"=0.0, "battery21voltage"=0.0, "battery22voltage"=0.0, "battery23voltage"=0.0, "battery24voltage"=0.0, "ErrorOutData"={"ErrorCode"=0, "ErrorMessage"=""}}, {"battery1voltage"=3.4816413, "battery2voltage"=3.4830415, "battery3voltage"=3.4783785, "battery4voltage"=3.482364, "battery5voltage"=3.4843998, "battery6voltage"=0.0, "battery7voltage"=0.0, "battery8voltage"=0.0, "battery9voltage"=0.0, "battery10voltage"=0.0, "battery11voltage"=0.0, "battery12voltage"=0.0, "battery13voltage"=0.0, "battery14voltage"=0.0, "battery15voltage"=0.0, "battery16voltage"=0.0, "battery17voltage"=0.0, "battery18voltage"=0.0, "battery19voltage"=0.0, "battery20voltage"=0.0, "battery21voltage"=0.0, "battery22voltage"=0.0, "battery23voltage"=0.0, "battery24voltage"=0.0, "ErrorOutData"={"ErrorCode"=0, "ErrorMessage"=""}}, {"battery1voltage"=3.4816387, "battery2voltage"=3.4830422, "battery3voltage"=3.47837, "battery4voltage"=3.4823673, "battery5voltage"=3.4844034, "battery6voltage"=0.0, "battery7voltage"=0.0, "battery8voltage"=0.0, "battery9voltage"=0.0, "battery10voltage"=0.0, "battery11voltage"=0.0, "battery12voltage"=0.0, "battery13voltage"=0.0, "battery14voltage"=0.0, "battery15voltage"=0.0, "battery16voltage"=0.0, "battery17voltage"=0.0, "battery18voltage"=0.0, "battery19voltage"=0.0, "battery20voltage"=0.0, "battery21voltage"=0.0, "battery22voltage"=0.0, "battery23voltage"=0.0, "battery24voltage"=0.0, "ErrorOutData"={"ErrorCode"=0, "ErrorMessage"=""}}, {"battery1voltage"=3.4816396, "battery2voltage"=3.4830437, "battery3voltage"=3.4783735, "battery4voltage"=3.4823701, "battery5voltage"=3.484399, "battery6voltage"=0.0, "battery7voltage"=0.0, "battery8voltage"=0.0, "battery9voltage"=0.0, "battery10voltage"=0.0, "battery11voltage"=0.0, "battery12voltage"=0.0, "battery13voltage"=0.0, "battery14voltage"=0.0, "battery15voltage"=0.0, "battery16voltage"=0.0, "battery17voltage"=0.0, "battery18voltage"=0.0, "battery19voltage"=0.0, "battery20voltage"=0.0, "battery21voltage"=0.0, "battery22voltage"=0.0, "battery23voltage"=0.0, "battery24voltage"=0.0, "ErrorOutData"={"ErrorCode"=0, "ErrorMessage"=""}}, {"battery1voltage"=3.4816391, "battery2voltage"=3.4830413, "battery3voltage"=3.4783726, "battery4voltage"=3.4823651, "battery5voltage"=3.484402, "battery6voltage"=0.0, "battery7voltage"=0.0, "battery8voltage"=0.0, "battery9voltage"=0.0, "battery10voltage"=0.0, "battery11voltage"=0.0, "battery12voltage"=0.0, "battery13voltage"=0.0, "battery14voltage"=0.0, "battery15voltage"=0.0, "battery16voltage"=0.0, "battery17voltage"=0.0, "battery18voltage"=0.0, "battery19voltage"=0.0, "battery20voltage"=0.0, "battery21voltage"=0.0, "battery22voltage"=0.0, "battery23voltage"=0.0, "battery24voltage"=0.0, "ErrorOutData"={"ErrorCode"=0, "ErrorMessage"=""}}, {"battery1voltage"=3.4816377, "battery2voltage"=3.4830375, "battery3voltage"=3.4783683, "battery4voltage"=3.4823647, "battery5voltage"=3.4844048, "battery6voltage"=0.0, "battery7voltage"=0.0, "battery8voltage"=0.0, "battery9voltage"=0.0, "battery10voltage"=0.0, "battery11voltage"=0.0, "battery12voltage"=0.0, "battery13voltage"=0.0, "battery14voltage"=0.0, "battery15voltage"=0.0, "battery16voltage"=0.0, "battery17voltage"=0.0, "battery18voltage"=0.0, "battery19voltage"=0.0, "battery20voltage"=0.0, "battery21voltage"=0.0, "battery22voltage"=0.0, "battery23voltage"=0.0, "battery24voltage"=0.0, "ErrorOutData"={"ErrorCode"=0, "ErrorMessage"=""}}, {"battery1voltage"=3.4816406, "battery2voltage"=3.4830425, "battery3voltage"=3.4783697, "battery4voltage"=3.4823635, "battery5voltage"=3.484403, "battery6voltage"=0.0, "battery7voltage"=0.0, "battery8voltage"=0.0, "battery9voltage"=0.0, "battery10voltage"=0.0, "battery11voltage"=0.0, "battery12voltage"=0.0, "battery13voltage"=0.0, "battery14voltage"=0.0, "battery15voltage"=0.0, "battery16voltage"=0.0, "battery17voltage"=0.0, "battery18voltage"=0.0, "battery19voltage"=0.0, "battery20voltage"=0.0, "battery21voltage"=0.0, "battery22voltage"=0.0, "battery23voltage"=0.0, "battery24voltage"=0.0, "ErrorOutData"={"ErrorCode"=0, "ErrorMessage"=""}}, {"battery1voltage"=3.481641, "battery2voltage"=3.4830472, "battery3voltage"=3.4783764, "battery4voltage"=3.4823675, "battery5voltage"=3.484406, "battery6voltage"=0.0, "battery7voltage"=0.0, "battery8voltage"=0.0, "battery9voltage"=0.0, "battery10voltage"=0.0, "battery11voltage"=0.0, "battery12voltage"=0.0, "battery13voltage"=0.0, "battery14voltage"=0.0, "battery15voltage"=0.0, "battery16voltage"=0.0, "battery17voltage"=0.0, "battery18voltage"=0.0, "battery19voltage"=0.0, "battery20voltage"=0.0, "battery21voltage"=0.0, "battery22voltage"=0.0, "battery23voltage"=0.0, "battery24voltage"=0.0, "ErrorOutData"={"ErrorCode"=0, "ErrorMessage"=""}}, {"battery1voltage"=3.4816406, "battery2voltage"=3.4830382, "battery3voltage"=3.478367, "battery4voltage"=3.4823632, "battery5voltage"=3.4844096, "battery6voltage"=0.0, "battery7voltage"=0.0, "battery8voltage"=0.0, "battery9voltage"=0.0, "battery10voltage"=0.0, "battery11voltage"=0.0, "battery12voltage"=0.0, "battery13voltage"=0.0, "battery14voltage"=0.0, "battery15voltage"=0.0, "battery16voltage"=0.0, "battery17voltage"=0.0, "battery18voltage"=0.0, "battery19voltage"=0.0, "battery20voltage"=0.0, "battery21voltage"=0.0, "battery22voltage"=0.0, "battery23voltage"=0.0, "battery24voltage"=0.0, "ErrorOutData"={"ErrorCode"=0, "ErrorMessage"=""}}, {"battery1voltage"=3.481635, "battery2voltage"=3.4830372, "battery3voltage"=3.47837, "battery4voltage"=3.4823704, "battery5voltage"=3.484407, "battery6voltage"=0.0, "battery7voltage"=0.0, "battery8voltage"=0.0, "battery9voltage"=0.0, "battery10voltage"=0.0, "battery11voltage"=0.0, "battery12voltage"=0.0, "battery13voltage"=0.0, "battery14voltage"=0.0, "battery15voltage"=0.0, "battery16voltage"=0.0, "battery17voltage"=0.0, "battery18voltage"=0.0, "battery19voltage"=0.0, "battery20voltage"=0.0, "battery21voltage"=0.0, "battery22voltage"=0.0, "battery23voltage"=0.0, "battery24voltage"=0.0, "ErrorOutData"={"ErrorCode"=0, "ErrorMessage"=""}}, {"battery1voltage"=3.4816337, "battery2voltage"=3.483038, "battery3voltage"=3.4783702, "battery4voltage"=3.4823666, "battery5voltage"=3.4844046, "battery6voltage"=0.0, "battery7voltage"=0.0, "battery8voltage"=0.0, "battery9voltage"=0.0, "battery10voltage"=0.0, "battery11voltage"=0.0, "battery12voltage"=0.0, "battery13voltage"=0.0, "battery14voltage"=0.0, "battery15voltage"=0.0, "battery16voltage"=0.0, "battery17voltage"=0.0, "battery18voltage"=0.0, "battery19voltage"=0.0, "battery20voltage"=0.0, "battery21voltage"=0.0, "battery22voltage"=0.0, "battery23voltage"=0.0, "battery24voltage"=0.0, "ErrorOutData"={"ErrorCode"=0, "ErrorMessage"=""}}]
  in  "Results Cluster":T3={"ch3 range"=1.5284304409643419e-06, "ch3 std dev"=3.7432297421944963e-07, "ch3 mean"=9.480335334891014e-06, "Histogram Graph ch3"={"X Values"=[8.804122636382775e-06, 8.956965680479209e-06, 9.109808724575643e-06, 9.262651768672077e-06, 9.415494812768511e-06, 9.568337856864946e-06, 9.72118090096138e-06, 9.874023945057814e-06, 1.0026866989154248e-05, 1.0179710033250682e-05], "Histogram: h(x)"=[2, 4, 3, 7, 5, 3, 7, 6, 1, 2]}, "ch2 range"=1.9041594218219493e-06, "ch2 std dev"=4.1579103732429095e-07, "ch2 mean"=5.730660716698524e-06, "Histogram Graph ch2"={"X Values"=[4.8417078226500296e-06, 5.032123764832224e-06, 5.222539707014419e-06, 5.412955649196613e-06, 5.603371591378808e-06, 5.7937875335610025e-06, 5.984203475743197e-06, 6.174619417925392e-06, 6.365035360107586e-06, 6.555451302289781e-06], "Histogram: h(x)"=[2, 2, 4, 3, 5, 8, 9, 5, 1, 1]}, "ch1 range"=1.7442902903444177e-06, "ch1 std dev"=4.468204660544414e-07, "ch1 mean"=-2.6579412172609335e-06, "Histogram Graph ch1"={"X Values"=[-3.3982864936427982e-06, -3.2238574646083565e-06, -3.0494284355739147e-06, -2.874999406539473e-06, -2.700570377505031e-06, -2.5261413484705894e-06, -2.3517123194361476e-06, -2.177283290401706e-06, -2.002854261367264e-06, -1.8284252323328223e-06], "Histogram: h(x)"=[4, 3, 5, 1, 6, 8, 4, 5, 3, 1]}, "ch0 range"=1.9838415017287296e-06, "ch0 std dev"=5.022029434534627e-07, "ch0 mean"=-6.648192609520545e-06, "Histogram Graph ch0"={"X Values"=[-7.4214795585101575e-06, -7.223095408337285e-06, -7.024711258164412e-06, -6.82632710799154e-06, -6.627942957818667e-06, -6.4295588076457944e-06, -6.231174657472922e-06, -6.032790507300049e-06, -5.8344063571271766e-06, -5.636022206954304e-06], "Histogram: h(x)"=[5, 3, 4, 6, 4, 8, 4, 1, 4, 1]}, "Waveform Chart ch1"=[-2.622437675041801e-06, -2.1054414953660847e-06, -2.3277676624794484e-06, -2.558376653803712e-06, -2.2236999675494533e-06, -2.589016451053761e-06, -2.6354278960691e-06, -2.7367192087189563e-06, -2.424017879995447e-06, -3.0489161443253215e-06, -3.1442148467963687e-06, -2.4032855210096374e-06, -2.569647882839888e-06, -2.4698150005498013e-06, -3.0781658817195746e-06, -2.377010372332436e-06, -2.0435595699758798e-06, -2.106839167327596e-06, -1.7412107178156014e-06, -3.2480049993772076e-06, -1.9805074376907754e-06, -2.5608807141114243e-06, -2.18054640635336e-06, -3.099457174386434e-06, -3.102303246629032e-06, -3.2920758007788295e-06, -3.3778499352142414e-06, -3.3187560901861313e-06, -3.484840052811922e-06, -3.485501008160019e-06, -2.8728971850629594e-06, -2.6623123946996634e-06, -2.187546597757112e-06, -2.5467930720162336e-06, -2.7862697099761513e-06, -2.528638777412977e-06, -2.0537236385737207e-06, -2.5329982714180255e-06, -2.7424337661967574e-06, -3.067742416854491e-06], "Waveform Chart ch2"=[5.544446756924017e-06, 5.893818847440082e-06, 5.6959361744068e-06, 6.353655436755351e-06, 6.650659273380882e-06, 6.187390686867271e-06, 6.20360970192913e-06, 5.7770612172558695e-06, 5.816303483036932e-06, 5.681492261411933e-06, 5.92762437831725e-06, 6.190843181120228e-06, 5.928079790707314e-06, 6.068116911256402e-06, 6.161619546592655e-06, 5.5543262999422065e-06, 6.17040032539053e-06, 5.4655577958543896e-06, 5.76704970728763e-06, 6.0194055222271105e-06, 5.783390336812049e-06, 5.768011867723238e-06, 6.0153044120154e-06, 6.001437704705948e-06, 5.911709913790112e-06, 5.830095407868431e-06, 5.25398022881523e-06, 5.15697143423068e-06, 4.826305970962092e-06, 5.462550730311096e-06, 5.059430867978049e-06, 5.682513029845579e-06, 5.851683523904261e-06, 5.099226732675129e-06, 5.2309820281174504e-06, 5.22374278950658e-06, 5.829274618675769e-06, 4.746499851558932e-06, 5.396447289671177e-06, 6.039472630669777e-06], "Waveform Chart ch0"=[-6.482741875349764e-06, -6.609674165618734e-06, -6.233203080218623e-06, -6.613210951394088e-06, -5.909245924550351e-06, -6.1328996888307884e-06, -6.358200673203053e-06, -6.870973185430456e-06, -6.243427483099904e-06, -5.953840097279857e-06, -6.577614794730629e-06, -5.768388563769013e-06, -5.889962020259323e-06, -5.91212430154465e-06, -6.419565311385181e-06, -6.50829315132552e-06, -5.536830131867864e-06, -6.271011369459595e-06, -6.937542782195293e-06, -7.44168991871554e-06, -6.8984467501811205e-06, -7.4441074466820366e-06, -6.884514522294152e-06, -7.229455884586274e-06, -7.204633996616539e-06, -7.520671633596594e-06, -7.348344858091178e-06, -7.026224856705287e-06, -6.4957495291395714e-06, -6.9697185324009035e-06, -6.64170832689038e-06, -6.516226556717238e-06, -6.80187883727134e-06, -7.473746530800666e-06, -6.8019074543289836e-06, -6.421730747707948e-06, -6.915517716049444e-06, -7.233306065769019e-06, -6.9335647318597554e-06, -6.495809932905111e-06], "Waveform Chart ch3"=[9.329772359568193e-06, 9.772186603754015e-06, 9.974785258468733e-06, 1.02561315552989e-05, 9.495402230894659e-06, 9.736598828932665e-06, 9.898850155608759e-06, 1.0197036488504313e-05, 9.305987891150035e-06, 9.316802834906767e-06, 9.746712874470878e-06, 9.737416581604666e-06, 9.867514527065477e-06, 9.509080464808271e-06, 9.481845866845764e-06, 9.70755176396829e-06, 8.885838770613302e-06, 9.475699672125386e-06, 9.258180372816345e-06, 9.834891872602234e-06, 9.402243918552161e-06, 9.713205786936326e-06, 9.876491292911543e-06, 9.871789580104262e-06, 9.650930388911628e-06, 9.41118365911455e-06, 9.575353492249282e-06, 9.196921234035763e-06, 9.15123272945548e-06, 8.949563027841687e-06, 9.474861956745276e-06, 8.825224921180636e-06, 8.727701114334558e-06, 9.16860173648142e-06, 8.905227736485157e-06, 9.144446889757383e-06, 8.885482293855075e-06, 9.859395612279415e-06, 9.32444154185109e-06, 9.310827508550253e-06]} {"ch3 range" format="%#_6p"; "ch3 std dev" format="%#.3p"; "ch3 mean" format="%#.6p"; "ch2 range" format="%#_6p"; "ch2 std dev" format="%#.3p"; "ch2 mean" format="%#.6p"; "ch1 range" format="%#_6p"; "ch1 std dev" format="%#.3p"; "ch1 mean" format="%#.6p"; "ch0 range" format="%#_6p"; "ch0 std dev" format="%#.3p"; "ch0 mean" format="%#.6p"}
  in  "4309 500 Hz":T4={"V ch0 Array"=[], "V ch1 Array"=[], "V ch2 Array"=[], "V ch3 Array"=[], "V ch4 Array"=[], "Elapsed Time (ms)"=11164, "DMM Fault Array"=[]}
  in  "4309 200 Hz":T4={"V ch0 Array"=[], "V ch1 Array"=[], "V ch2 Array"=[], "V ch3 Array"=[], "V ch4 Array"=[], "Elapsed Time (ms)"=11164, "DMM Fault Array"=[]}
  in  "4309 100 Hz":T4={"V ch0 Array"=[], "V ch1 Array"=[], "V ch2 Array"=[], "V ch3 Array"=[], "V ch4 Array"=[], "Elapsed Time (ms)"=11164, "DMM Fault Array"=[]}
  in  "4309 10 Hz":T4={"V ch0 Array"=[], "V ch1 Array"=[], "V ch2 Array"=[], "V ch3 Array"=[], "V ch4 Array"=[], "Elapsed Time (ms)"=11164, "DMM Fault Array"=[]}
  in  "4309 12 Hz":T4={"V ch0 Array"=[], "V ch1 Array"=[], "V ch2 Array"=[], "V ch3 Array"=[], "V ch4 Array"=[], "Elapsed Time (ms)"=11164, "DMM Fault Array"=[]}
  in  "4309 15 Hz":T4={"V ch0 Array"=[], "V ch1 Array"=[], "V ch2 Array"=[], "V ch3 Array"=[], "V ch4 Array"=[], "Elapsed Time (ms)"=11164, "DMM Fault Array"=[]}
  in  "4309 20 Hz":T4={"V ch0 Array"=[], "V ch1 Array"=[], "V ch2 Array"=[], "V ch3 Array"=[], "V ch4 Array"=[], "Elapsed Time (ms)"=11164, "DMM Fault Array"=[]}
  in  "4309 30 Hz":T4={"V ch0 Array"=[], "V ch1 Array"=[], "V ch2 Array"=[], "V ch3 Array"=[], "V ch4 Array"=[], "Elapsed Time (ms)"=11164, "DMM Fault Array"=[]}
  in  "4309 60 Hz":T4={"V ch0 Array"=[], "V ch1 Array"=[], "V ch2 Array"=[], "V ch3 Array"=[], "V ch4 Array"=[], "Elapsed Time (ms)"=11164, "DMM Fault Array"=[]}
  out "ch3 range":dbl=1.5284304409643419e-06 format="%#_6p"
  out "ch3 std dev":dbl=3.7432297421944963e-07 format="%#.3p"
  out "ch3 mean":dbl=9.480335334891014e-06 format="%#.6p"
  out "Histogram Graph ch3":T5(graph)={"X Values"=[8.804122636382775e-06, 8.956965680479209e-06, 9.109808724575643e-06, 9.262651768672077e-06, 9.415494812768511e-06, 9.568337856864946e-06, 9.72118090096138e-06, 9.874023945057814e-06, 1.0026866989154248e-05, 1.0179710033250682e-05], "Histogram: h(x)"=[2, 4, 3, 7, 5, 3, 7, 6, 1, 2]}
  out "ch2 range":dbl=1.9041594218219493e-06 format="%#_6p"
  out "ch2 std dev":dbl=4.1579103732429095e-07 format="%#.3p"
  out "ch2 mean":dbl=5.730660716698524e-06 format="%#.6p"
  out "Histogram Graph ch2":T5(graph)={"X Values"=[4.8417078226500296e-06, 5.032123764832224e-06, 5.222539707014419e-06, 5.412955649196613e-06, 5.603371591378808e-06, 5.7937875335610025e-06, 5.984203475743197e-06, 6.174619417925392e-06, 6.365035360107586e-06, 6.555451302289781e-06], "Histogram: h(x)"=[2, 2, 4, 3, 5, 8, 9, 5, 1, 1]}
  out "ch1 range":dbl=1.7442902903444177e-06 format="%#_6p"
  out "ch1 std dev":dbl=4.468204660544414e-07 format="%#.3p"
  out "ch1 mean":dbl=-2.6579412172609335e-06 format="%#.6p"
  out "Histogram Graph ch1":T5(graph)={"X Values"=[-3.3982864936427982e-06, -3.2238574646083565e-06, -3.0494284355739147e-06, -2.874999406539473e-06, -2.700570377505031e-06, -2.5261413484705894e-06, -2.3517123194361476e-06, -2.177283290401706e-06, -2.002854261367264e-06, -1.8284252323328223e-06], "Histogram: h(x)"=[4, 3, 5, 1, 6, 8, 4, 5, 3, 1]}
  out "ch0 range":dbl=1.9838415017287296e-06 format="%#_6p"
  out "ch0 std dev":dbl=5.022029434534627e-07 format="%#.3p"
  out "ch0 mean":dbl=-6.648192609520545e-06 format="%#.6p"
  out "Histogram Graph ch0":T5(graph)={"X Values"=[-7.4214795585101575e-06, -7.223095408337285e-06, -7.024711258164412e-06, -6.82632710799154e-06, -6.627942957818667e-06, -6.4295588076457944e-06, -6.231174657472922e-06, -6.032790507300049e-06, -5.8344063571271766e-06, -5.636022206954304e-06], "Histogram: h(x)"=[5, 3, 4, 6, 4, 8, 4, 1, 4, 1]}
  out "Waveform Chart ch1":dbl[](graph)=[-2.622437675041801e-06, -2.1054414953660847e-06, -2.3277676624794484e-06, -2.558376653803712e-06, -2.2236999675494533e-06, -2.589016451053761e-06, -2.6354278960691e-06, -2.7367192087189563e-06, -2.424017879995447e-06, -3.0489161443253215e-06, -3.1442148467963687e-06, -2.4032855210096374e-06, -2.569647882839888e-06, -2.4698150005498013e-06, -3.0781658817195746e-06, -2.377010372332436e-06, -2.0435595699758798e-06, -2.106839167327596e-06, -1.7412107178156014e-06, -3.2480049993772076e-06, -1.9805074376907754e-06, -2.5608807141114243e-06, -2.18054640635336e-06, -3.099457174386434e-06, -3.102303246629032e-06, -3.2920758007788295e-06, -3.3778499352142414e-06, -3.3187560901861313e-06, -3.484840052811922e-06, -3.485501008160019e-06, -2.8728971850629594e-06, -2.6623123946996634e-06, -2.187546597757112e-06, -2.5467930720162336e-06, -2.7862697099761513e-06, -2.528638777412977e-06, -2.0537236385737207e-06, -2.5329982714180255e-06, -2.7424337661967574e-06, -3.067742416854491e-06]
  out "Waveform Chart ch2":dbl[](graph)=[5.544446756924017e-06, 5.893818847440082e-06, 5.6959361744068e-06, 6.353655436755351e-06, 6.650659273380882e-06, 6.187390686867271e-06, 6.20360970192913e-06, 5.7770612172558695e-06, 5.816303483036932e-06, 5.681492261411933e-06, 5.92762437831725e-06, 6.190843181120228e-06, 5.928079790707314e-06, 6.068116911256402e-06, 6.161619546592655e-06, 5.5543262999422065e-06, 6.17040032539053e-06, 5.4655577958543896e-06, 5.76704970728763e-06, 6.0194055222271105e-06, 5.783390336812049e-06, 5.768011867723238e-06, 6.0153044120154e-06, 6.001437704705948e-06, 5.911709913790112e-06, 5.830095407868431e-06, 5.25398022881523e-06, 5.15697143423068e-06, 4.826305970962092e-06, 5.462550730311096e-06, 5.059430867978049e-06, 5.682513029845579e-06, 5.851683523904261e-06, 5.099226732675129e-06, 5.2309820281174504e-06, 5.22374278950658e-06, 5.829274618675769e-06, 4.746499851558932e-06, 5.396447289671177e-06, 6.039472630669777e-06]
  out "Waveform Chart ch0":dbl[](graph)=[-6.482741875349764e-06, -6.609674165618734e-06, -6.233203080218623e-06, -6.613210951394088e-06, -5.909245924550351e-06, -6.1328996888307884e-06, -6.358200673203053e-06, -6.870973185430456e-06, -6.243427483099904e-06, -5.953840097279857e-06, -6.577614794730629e-06, -5.768388563769013e-06, -5.889962020259323e-06, -5.91212430154465e-06, -6.419565311385181e-06, -6.50829315132552e-06, -5.536830131867864e-06, -6.271011369459595e-06, -6.937542782195293e-06, -7.44168991871554e-06, -6.8984467501811205e-06, -7.4441074466820366e-06, -6.884514522294152e-06, -7.229455884586274e-06, -7.204633996616539e-06, -7.520671633596594e-06, -7.348344858091178e-06, -7.026224856705287e-06, -6.4957495291395714e-06, -6.9697185324009035e-06, -6.64170832689038e-06, -6.516226556717238e-06, -6.80187883727134e-06, -7.473746530800666e-06, -6.8019074543289836e-06, -6.421730747707948e-06, -6.915517716049444e-06, -7.233306065769019e-06, -6.9335647318597554e-06, -6.495809932905111e-06]
  out "Waveform Chart ch3":dbl[](graph)=[9.329772359568193e-06, 9.772186603754015e-06, 9.974785258468733e-06, 1.02561315552989e-05, 9.495402230894659e-06, 9.736598828932665e-06, 9.898850155608759e-06, 1.0197036488504313e-05, 9.305987891150035e-06, 9.316802834906767e-06, 9.746712874470878e-06, 9.737416581604666e-06, 9.867514527065477e-06, 9.509080464808271e-06, 9.481845866845764e-06, 9.70755176396829e-06, 8.885838770613302e-06, 9.475699672125386e-06, 9.258180372816345e-06, 9.834891872602234e-06, 9.402243918552161e-06, 9.713205786936326e-06, 9.876491292911543e-06, 9.871789580104262e-06, 9.650930388911628e-06, 9.41118365911455e-06, 9.575353492249282e-06, 9.196921234035763e-06, 9.15123272945548e-06, 8.949563027841687e-06, 9.474861956745276e-06, 8.825224921180636e-06, 8.727701114334558e-06, 9.16860173648142e-06, 8.905227736485157e-06, 9.144446889757383e-06, 8.885482293855075e-06, 9.859395612279415e-06, 9.32444154185109e-06, 9.310827508550253e-06]
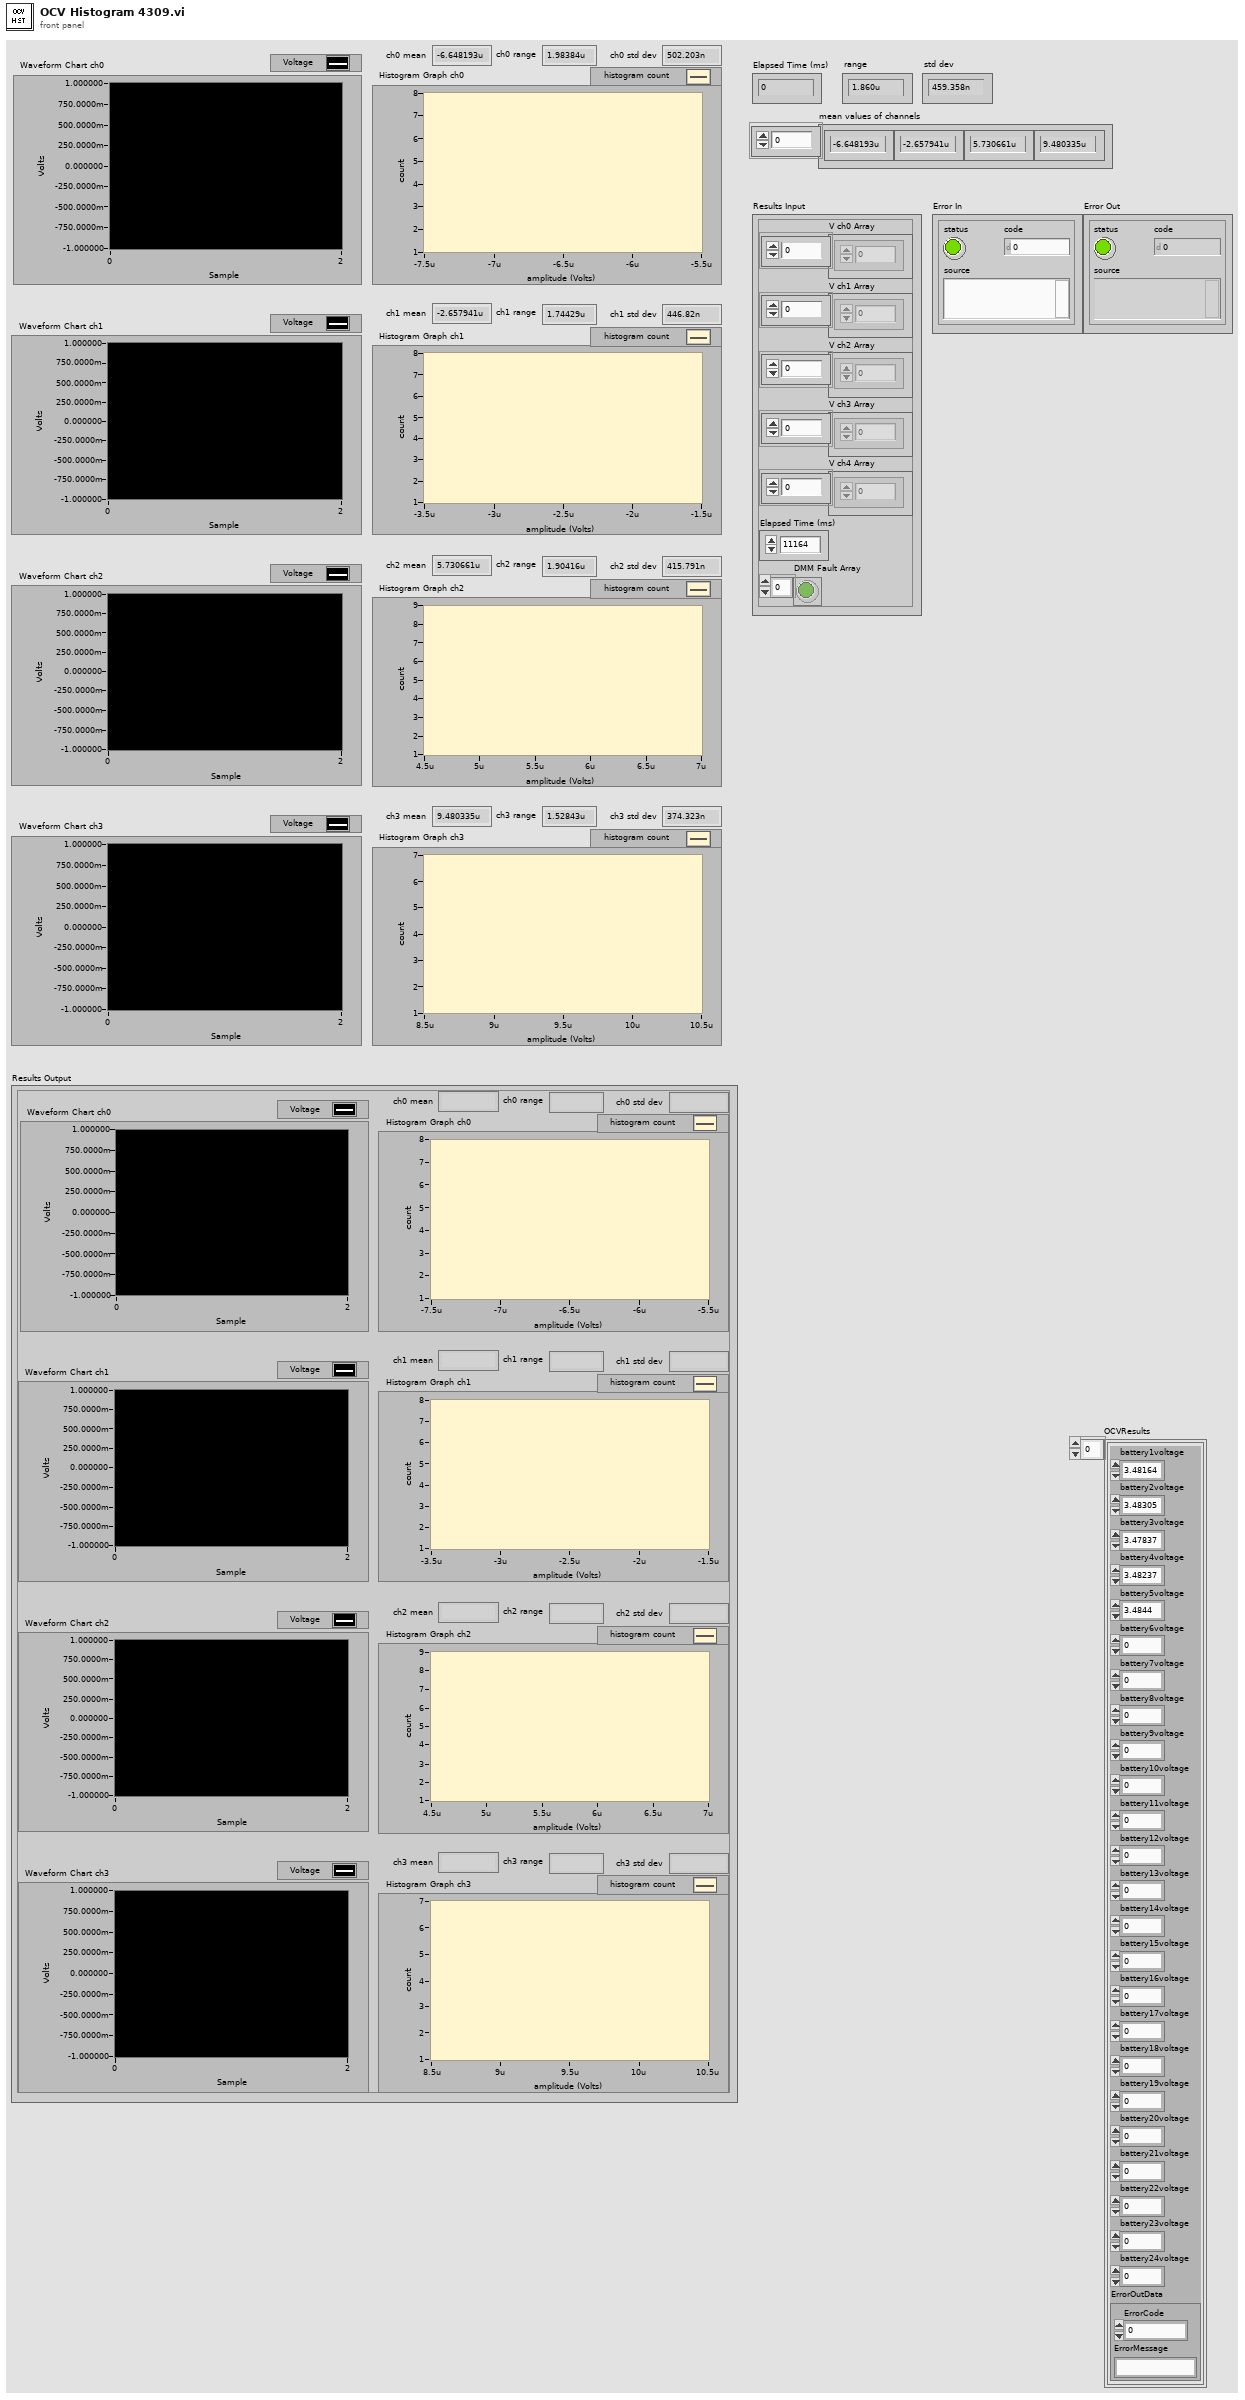
[diagram p1: front panel]
types:
  T1 = typedef "labview-grpc-measurement-server.lvlib/MeasurementServer_OCVRawData.ctl" = cluster{"battery1voltage":sgl, "battery2voltage":sgl, "battery3voltage":sgl, "battery4voltage":sgl, "battery5voltage":sgl, "battery6voltage":sgl, "battery7voltage":sgl, "battery8voltage":sgl, "battery9voltage":sgl, "battery10voltage":sgl, "battery11voltage":sgl, "battery12voltage":sgl, "battery13voltage":sgl, "battery14voltage":sgl, "battery15voltage":sgl, "battery16voltage":sgl, "battery17voltage":sgl, "battery18voltage":sgl, "battery19voltage":sgl, "battery20voltage":sgl, "battery21voltage":sgl, "battery22voltage":sgl, "battery23voltage":sgl, "battery24voltage":sgl, "ErrorOutData":T2}
  T2 = typedef "labview-grpc-measurement-server.lvlib/MeasurementServer_ErrorOutData.ctl" = cluster{"ErrorCode":i32, "ErrorMessage":string}
  T3 = typedef "Chart_Graph_Mean_Range_StdDev.ctl" = cluster{"ch3 range":dbl, "ch3 std dev":dbl, "ch3 mean":dbl, "Histogram Graph ch3":cluster{"X Values":dbl[], "Histogram: h(x)":i32[]}, "ch2 range":dbl, "ch2 std dev":dbl, "ch2 mean":dbl, "Histogram Graph ch2":cluster{"X Values":dbl[], "Histogram: h(x)":i32[]}, "ch1 range":dbl, "ch1 std dev":dbl, "ch1 mean":dbl, "Histogram Graph ch1":cluster{"X Values":dbl[], "Histogram: h(x)":i32[]}, "ch0 range":dbl, "ch0 std dev":dbl, "ch0 mean":dbl, "Histogram Graph ch0":cluster{"X Values":dbl[], "Histogram: h(x)":i32[]}, "Waveform Chart ch1":dbl[], "Waveform Chart ch2":dbl[], "Waveform Chart ch0":dbl[], "Waveform Chart ch3":dbl[]}
  T4 = typedef "OCVResults.ctl" = cluster{"V ch0 Array":dbl[], "V ch1 Array":dbl[], "V ch2 Array":dbl[], "V ch3 Array":dbl[], "V ch4 Array":dbl[], "Elapsed Time (ms)":u32, "DMM Fault Array":bool[]}
  T5 = cluster{"X Values":dbl[], "Histogram: h(x)":i32[]}
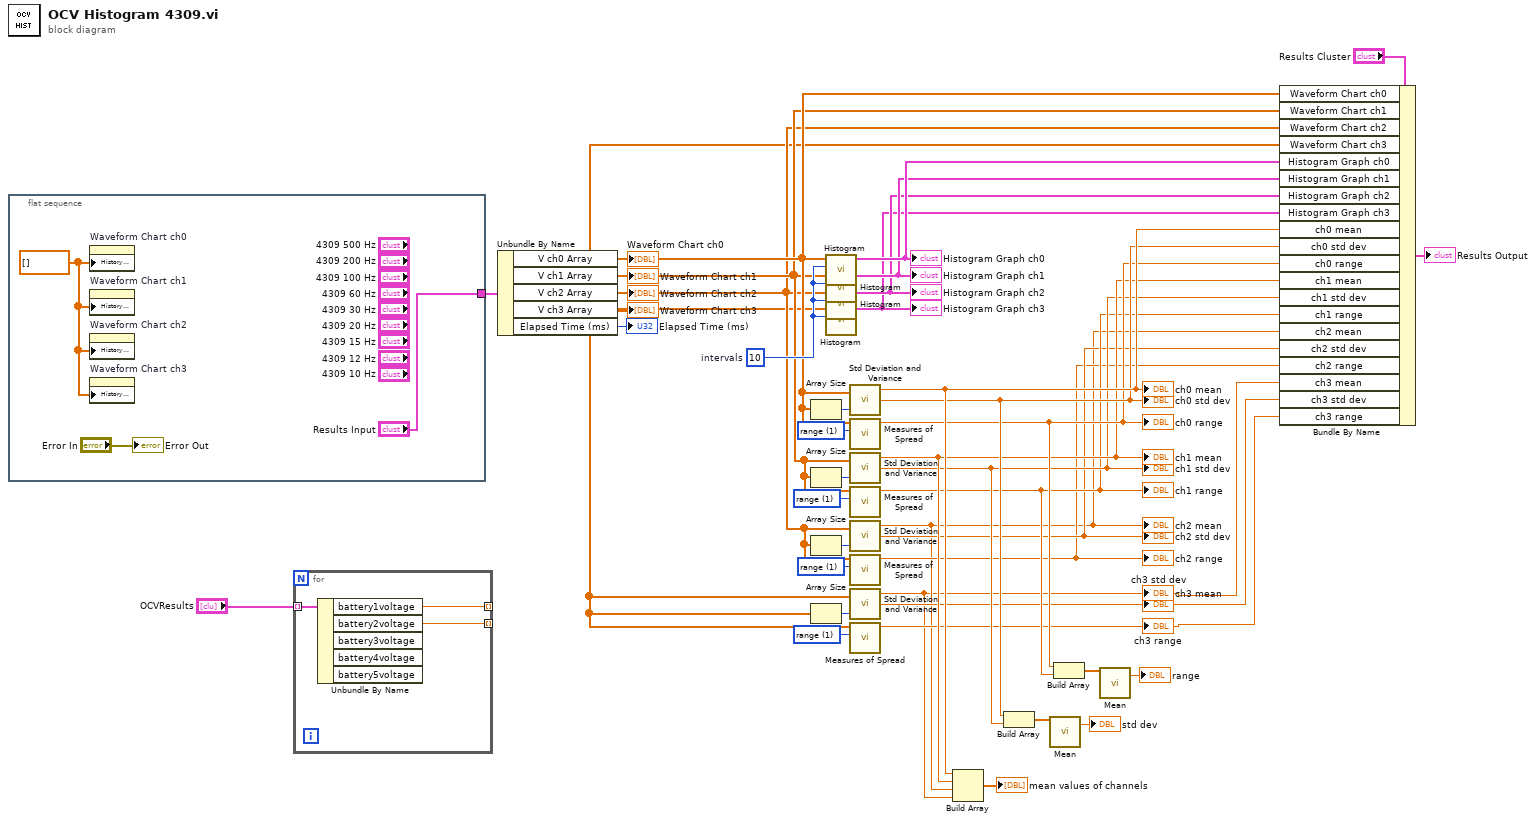
[diagram p0: block diagram]
diagram:
  w31 = 1 items=["standard deviation", "range", "mean absolute deviation", "interquartile range"] ("type")
  w33 = 1 items=["standard deviation", "range", "mean absolute deviation", "interquartile range"] ("type")
  w35 = 1 items=["standard deviation", "range", "mean absolute deviation", "interquartile range"] ("type")
  w37 = 1 items=["standard deviation", "range", "mean absolute deviation", "interquartile range"] ("type")
  w39 = 10  # intervals
  n1 = flat-sequence {
    tunnel: ["Results Input"] -> w25
    frame #0 {
      w42 = dbl[] [] ("History Data")
      n2 = property on="Waveform Chart ch0" class="WFChart (strict)"("History Data"=w42) -> ()  [unwired: 2 in, 2 out]
      n3 = property on="Waveform Chart ch1" class="WFChart (strict)"("History Data"=w42) -> ()  [unwired: 2 in, 2 out]
      n4 = property on="Waveform Chart ch2" class="WFChart (strict)"("History Data"=w42) -> ()  [unwired: 2 in, 2 out]
      n5 = property on="Waveform Chart ch3" class="WFChart (strict)"("History Data"=w42) -> ()  [unwired: 2 in, 2 out]
      "Error Out" <- "Error In"
    }
  }
  n6 = for {
    tunnel: "OCVResults" -> [w45] mode=indexing
    tunnel: [w44] -> _ mode=indexing
    tunnel: [w43] -> _ mode=indexing
    n7 = Unbundle By Name(w45) -> ("battery1voltage"=w44:sgl, "battery2voltage"=w43:sgl)  [unwired: 3 out]
  }
  n8 = Unbundle By Name(w25) -> ("V ch0 Array"=w22:dbl[], "V ch1 Array"=w21:dbl[], "V ch2 Array"=w20:dbl[], "V ch3 Array"=w19:dbl[], "Elapsed Time (ms)"=→"Elapsed Time (ms)":u32)
  "Waveform Chart ch3" <- w19
  "Waveform Chart ch0" <- w22
  "Waveform Chart ch2" <- w20
  "Waveform Chart ch1" <- w21
  n9 = Array Size(array=w22) -> (size(s)=w38:i32)
  n10 = Array Size(array=w21) -> (size(s)=w36:i32)
  n11 = Array Size(array=w20) -> (size(s)=w34:i32)
  n12 = Array Size(array=w19) -> (size(s)=w32:i32)
  n13 = call <vilib>:"Histogram.vi"("intervals"=w39, "X"=w22) -> ("Histogram Graph"=w18:T5)  [unwired: 6 in, 3 out]
  "Histogram Graph ch0" <- w18
  n14 = call <vilib>:"Histogram.vi"("intervals"=w39, "X"=w21) -> ("Histogram Graph"=w17:T5)  [unwired: 6 in, 3 out]
  "Histogram Graph ch1" <- w17
  n15 = call <vilib>:"Histogram.vi"("intervals"=w39, "X"=w20) -> ("Histogram Graph"=w16:T5)  [unwired: 6 in, 3 out]
  "Histogram Graph ch2" <- w16
  n16 = call <vilib>:"Histogram.vi"("intervals"=w39, "X"=w19) -> ("Histogram Graph"=w15:T5)  [unwired: 6 in, 3 out]
  "Histogram Graph ch3" <- w15
  n17 = call <vilib>:"Std Deviation and Variance.vi"("X"=w22, "Weighting (Sample)"=w38) -> ("mean"=w14:dbl, "standard deviation"=w13:dbl)  [unwired: 1 out]
  "ch0 mean" <- w14
  "ch0 std dev" <- w13
  n18 = call <vilib>:"Measures of Spread.vi"("type"=w37, "x array"=w22) -> ("spread value"=w12:dbl)  [unwired: 8 in, 1 out]
  "ch0 range" <- w12
  n19 = call <vilib>:"Std Deviation and Variance.vi"("X"=w21, "Weighting (Sample)"=w36) -> ("mean"=w11:dbl, "standard deviation"=w10:dbl)  [unwired: 1 out]
  "ch1 mean" <- w11
  "ch1 std dev" <- w10
  n20 = call <vilib>:"Measures of Spread.vi"("type"=w35, "x array"=w21) -> ("spread value"=w9:dbl)  [unwired: 8 in, 1 out]
  "ch1 range" <- w9
  n21 = call <vilib>:"Std Deviation and Variance.vi"("X"=w20, "Weighting (Sample)"=w34) -> ("mean"=w3:dbl, "standard deviation"=w8:dbl)  [unwired: 1 out]
  "ch2 mean" <- w3
  "ch2 std dev" <- w8
  n22 = call <vilib>:"Measures of Spread.vi"("type"=w33, "x array"=w20) -> ("spread value"=w7:dbl)  [unwired: 8 in, 1 out]
  "ch2 range" <- w7
  n23 = call <vilib>:"Std Deviation and Variance.vi"("X"=w19, "Weighting (Sample)"=w32) -> ("mean"=w2:dbl, "standard deviation"=w6:dbl)  [unwired: 1 out]
  "ch3 mean" <- w2
  "ch3 std dev" <- w6
  n24 = call <vilib>:"Measures of Spread.vi"("type"=w31, "x array"=w19) -> ("spread value"=w5:dbl)  [unwired: 8 in, 1 out]
  "ch3 range" <- w5
  n25 = Build Array(w14, w11, w3, w2) -> (→"mean values of channels":dbl[])
  n26 = Build Array(w13, w10) -> (w29:dbl[])
  n27 = call-poly <vilib>:"Mean.vi"("X"=w29) -> ("mean"=→"std dev":dbl)  [unwired: 1 out]
  n28 = Build Array(w12, w9) -> (w27:dbl[])
  n29 = call-poly <vilib>:"Mean.vi"("X"=w27) -> ("mean"=→"range":dbl)  [unwired: 1 out]
  n30 = Bundle By Name(cluster="Results Cluster", "Waveform Chart ch0"=w22, "Waveform Chart ch1"=w21, "Waveform Chart ch2"=w20, "Waveform Chart ch3"=w19, "Histogram Graph ch0"=w18, "Histogram Graph ch1"=w17, "Histogram Graph ch2"=w16, "Histogram Graph ch3"=w15, "ch0 mean"=w14, "ch0 std dev"=w13, "ch0 range"=w12, "ch1 mean"=w11, "ch1 std dev"=w10, "ch1 range"=w9, "ch2 mean"=w3, "ch2 std dev"=w8, "ch2 range"=w7, "ch3 mean"=w2, "ch3 std dev"=w6, "ch3 range"=w5) -> (→"Results Output":T3)
